vi "数据编码.vi"(0 "table输入":string(combo), 5 "错误常量 2":errorcluster caption="错误输入", 9 "QN":string, 13 "MN":string, 14 "PW":string) -> (4 "错误常量":errorcluster caption="错误输出", 15 "通讯包字符串":string)   [LabVIEW 2016, in "数据传输系统.lvlib"]
panel:
  in  "时间戳 2":string
  out "核查数据发送次数":i32
  out "小时数据发送次数":i32
  out "长度":i32
  in  "数据块":T1
  out "通讯包":T2={"包头（2）"="##", "数据段长度（4）"="", "数据段"="", "CRC校验"="", "包尾"=""}
  # "范例代码：\n\n##0101QN=20160801085857223;ST=32;CN=1062;PW=100000;MN=010000A8900016F000169DC0;Flag=5\n;CP=&&RtdInterval=30&&1C80\\r\\n"
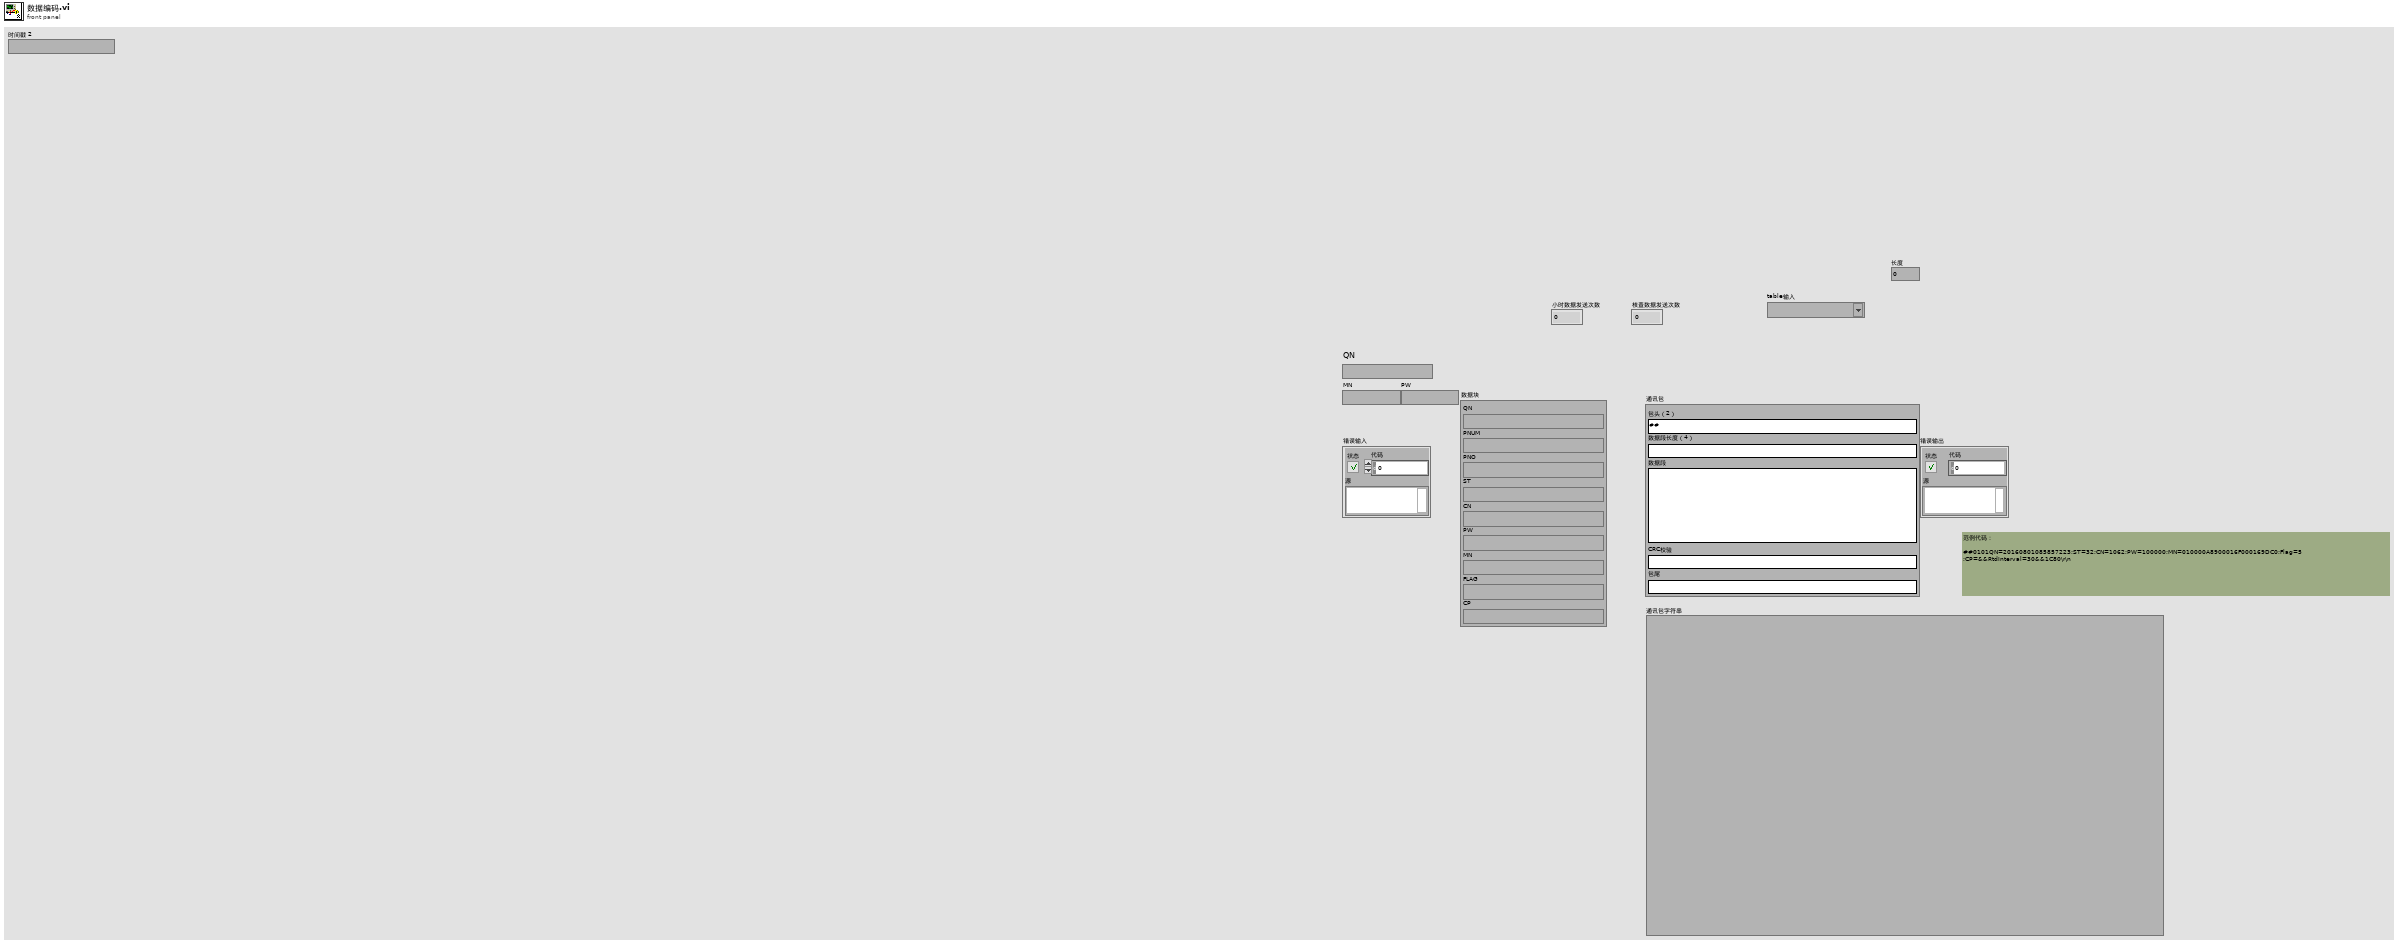
[diagram p1: front panel]
types:
  T1 = cluster{"QN":string, "ST":string, "CN":string, "PW":string, "MN":string, "FLAG":string, "PNUM":string, "PNO":string, "CP":string}
  T2 = cluster{"包头（2）":string, "数据段长度（4）":string, "数据段":string, "CRC校验":string, "包尾":string}
  T3 = cluster{"PH":string[][], "CODCr":string[][], "氨氮":string[][], "CODMn":string[][], "总氮":string[][], "总磷":string[][], "电导率":string[][], "水温":string[][], "DO":string[][], "浊度":string[][], "叶绿素":string[][], "藻密度":string[][], "铜":string[][], "盐度":string[][], "水位":string[][], "流速":string[][], "瞬时流量":string[][], "累计流量":string[][]}
  T4 = cluster{"PH":string[][], "CODCr":string[][], "氨氮":string[][], "CODMn":string[][], "总氮":string[][], "总磷":string[][], "电导率":string[][], "水温":string[][], "DO":string[][], "浊度":string[][], "叶绿素":string[][], "藻密度":string[][], "铜":string[][], "盐度":string[][], "水位":string[][], "流速":string[][], "瞬时流量":string[][], "累积流量":string[][]}
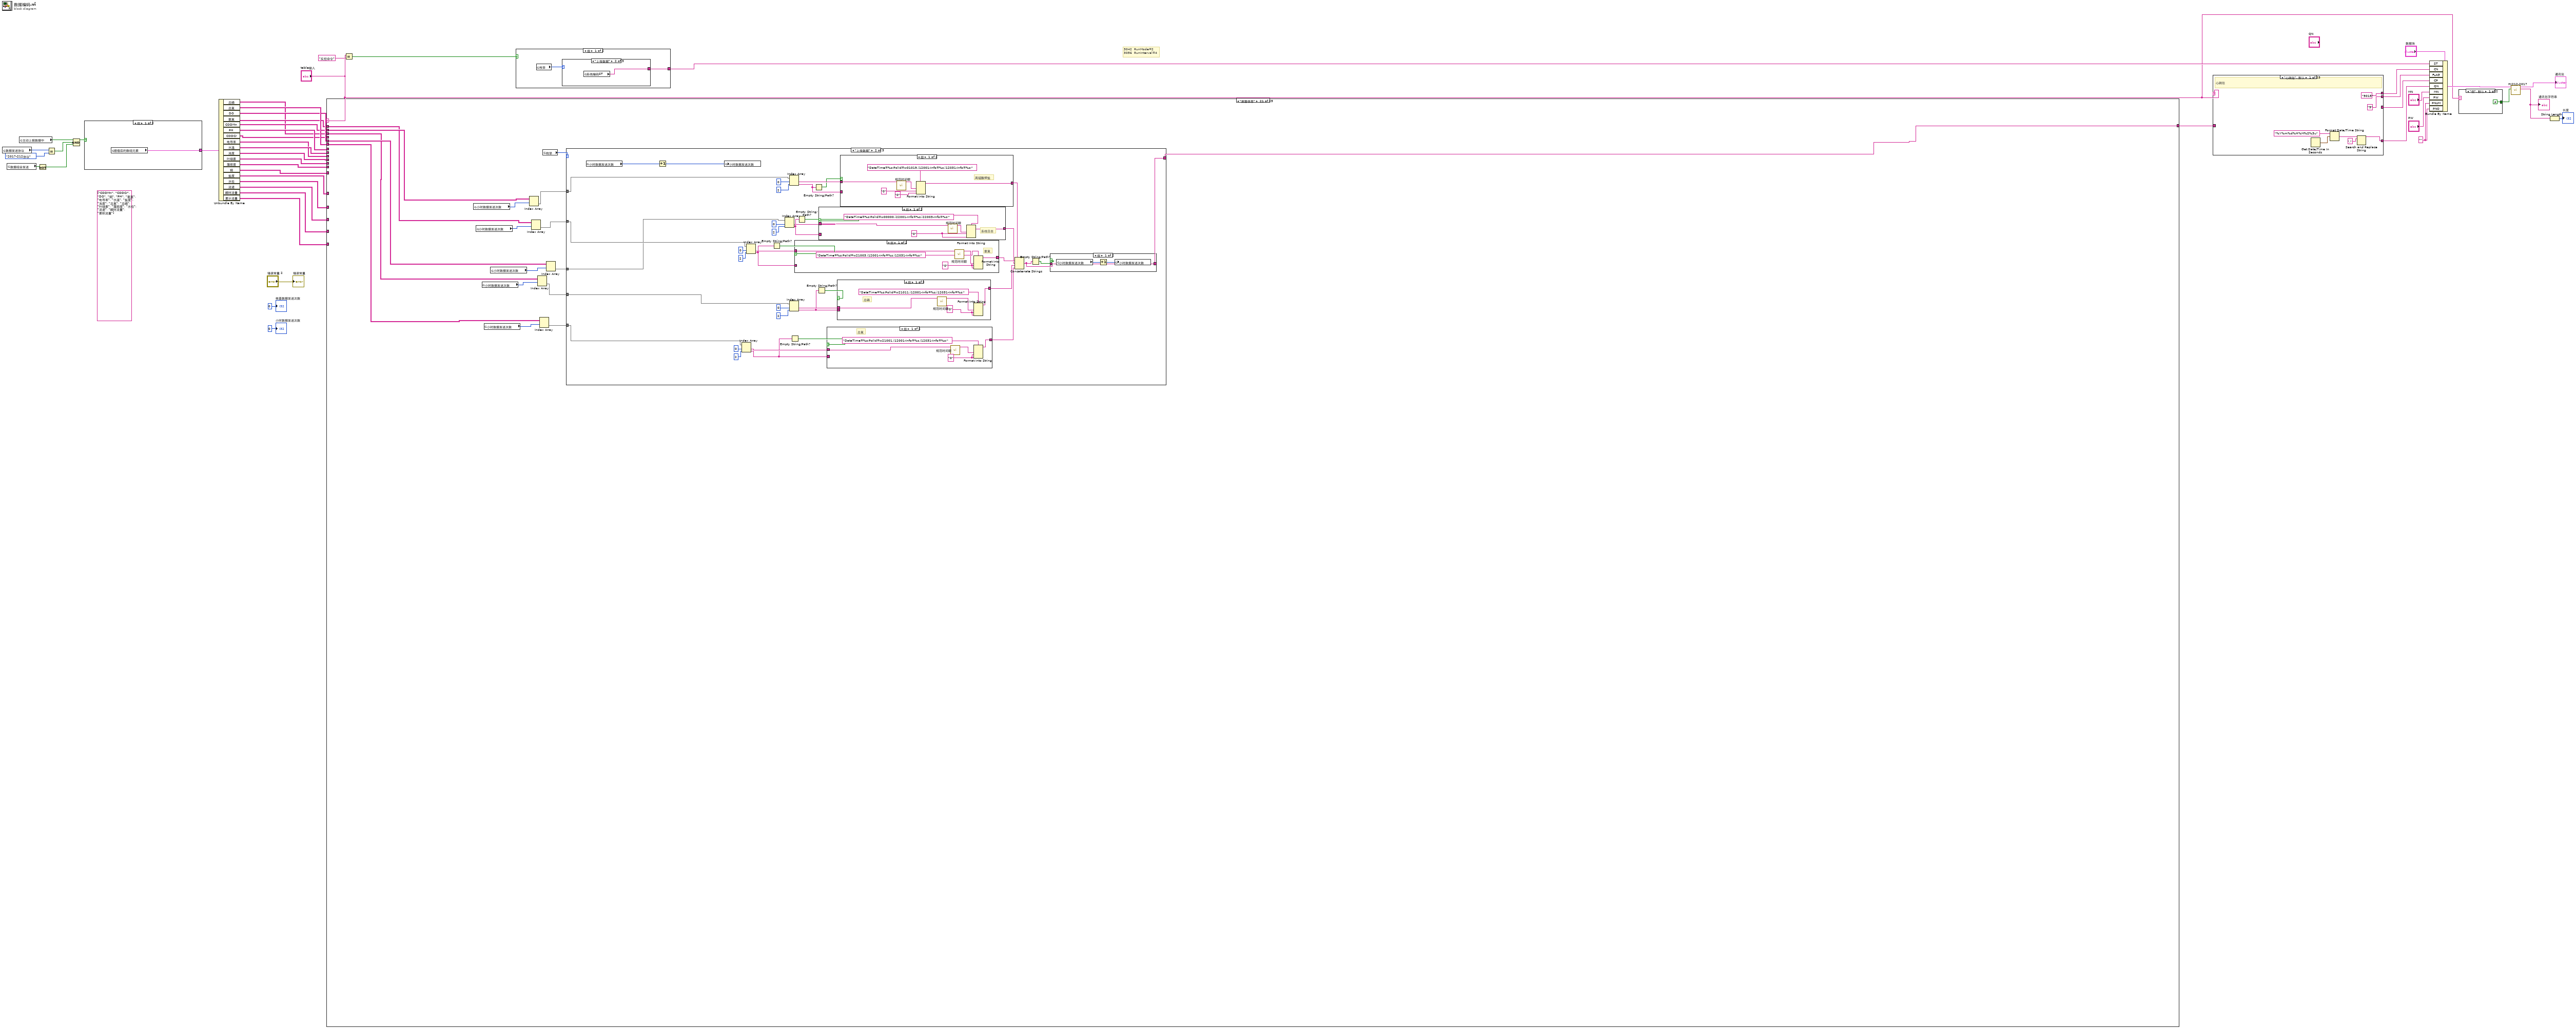
[diagram p0: block diagram]
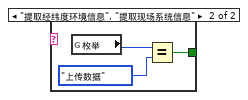
[diagram p2: hidden frame]
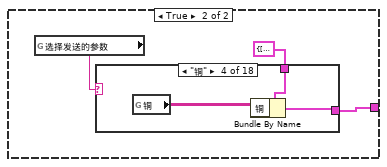
[diagram p3: hidden frame]
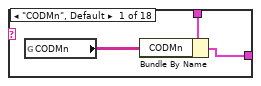
[diagram p4: hidden frame]
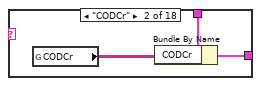
[diagram p5: hidden frame]
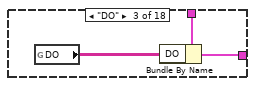
[diagram p6: hidden frame]
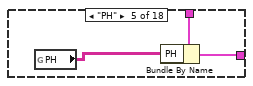
[diagram p7: hidden frame]
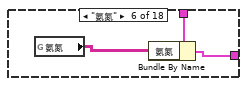
[diagram p8: hidden frame]
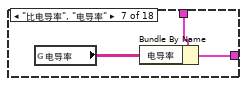
[diagram p9: hidden frame]
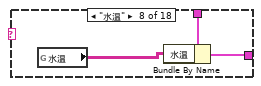
[diagram p10: hidden frame]
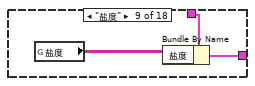
[diagram p11: hidden frame]
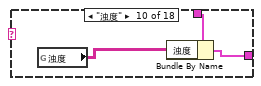
[diagram p12: hidden frame]
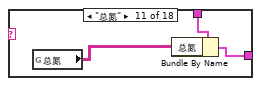
[diagram p13: hidden frame]
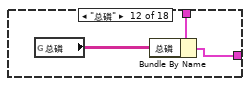
[diagram p14: hidden frame]
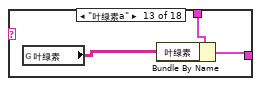
[diagram p15: hidden frame]
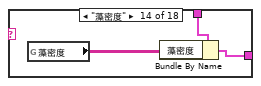
[diagram p16: hidden frame]
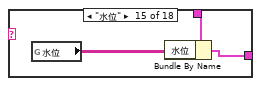
[diagram p17: hidden frame]
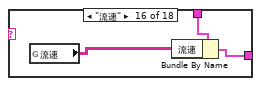
[diagram p18: hidden frame]
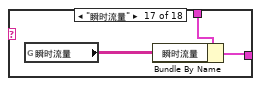
[diagram p19: hidden frame]
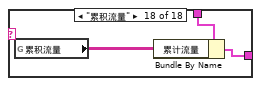
[diagram p20: hidden frame]
diagram:
  (unwired) string[] ["CODMn", "CODCr", "DO", "铜", "PH", "氨氮", "电导率", "水温", "盐度", "浊度", "总氮", "总磷", "叶绿素", "藻密度", "水位", "流速", "瞬时流量", "累积流量"] ("查询参数数组")
  w31 = ""
  # "3042  RunMode=2\n3056  RunInterval=4"
  n1 = global read "断电保存全局.vi" "数据发送协议"() -> (w1:enum16{"2005-212协议", "2017-212协议"})
  n2 = global read "断电保存全局.vi" "数据组合发送"() -> (w3:bool)
  n3 = global read "全局 数据发送重叠.vi" "主动上报数据中"() -> (w17:bool)
  n4 = Not(x=w3) -> (.not. x?=w2:bool)
  n5 = Equal?(x=w1, y=enum16{"2005-212协议", "2017-212协议"}."2017-212协议" ("数据发送版本")) -> (x = y?=w6:bool)
  n6 = Compound Arithmetic op=AND ("复合运算")(w17, w6, w2) -> (w7:bool)
  n7 = case shown="假" w7 {
    tunnel: [w48 w50] -> w18
    frame False {
      n8 = global read "插值后的新数组.vi" "插值后的数组元素"() -> (w48:T4)
    }
    frame True {
      n9 = global read "全局 水样时间.vi" "选择发送的参数"() -> (w51:string)
      n10 = case shown="\"铜\"" w51 {
        tunnel: T3 {"PH"=[], "CODCr"=[], "氨氮"=[], "CODMn"=[], "总氮"=[], "总磷"=[], "电导率"=[], "水温"=[], "DO"=[], "浊度"=[], "叶绿素"=[], "藻密度"=[], "铜"=[], "盐度"=[], "水位"=[], "流速"=[], "瞬时流量"=[], "累计流量"=[]} ("插值后的数组元素") -> [w53 w57 w60 w63 w66 w69 w72 w75 w78 w81 w84 w87 w90 w92 w96 w99 w101 w104]
        tunnel: [w52 w55 w58 w61 w64 w67 w71 w74 w76 w79 w82 w85 w88 w91 w94 w97 w100 w103] -> w50
        frame "CODMn", Default {
          n11 = global read "全局 所有参数.vi" "CODMn"() -> (w54:string[][])
          n12 = Bundle By Name(cluster=w53, "CODMn"=w54) -> (w52:T3)
        }
        frame "CODCr" {
          n13 = global read "全局 所有参数.vi" "CODCr"() -> (w56:string[][])
          n14 = Bundle By Name(cluster=w57, "CODCr"=w56) -> (w55:T3)
        }
        frame "DO" {
          n15 = global read "全局 所有参数.vi" "DO"() -> (w59:string[][])
          n16 = Bundle By Name(cluster=w60, "DO"=w59) -> (w58:T3)
        }
        frame "铜" {
          n17 = global read "全局 所有参数.vi" "铜"() -> (w62:string[][])
          n18 = Bundle By Name(cluster=w63, "铜"=w62) -> (w61:T3)
        }
        frame "PH" {
          n19 = global read "全局 所有参数.vi" "PH"() -> (w65:string[][])
          n20 = Bundle By Name(cluster=w66, "PH"=w65) -> (w64:T3)
        }
        frame "氨氮" {
          n21 = global read "全局 所有参数.vi" "氨氮"() -> (w68:string[][])
          n22 = Bundle By Name(cluster=w69, "氨氮"=w68) -> (w67:T3)
        }
        frame "比电导率", "电导率" {
          n23 = global read "全局 所有参数.vi" "电导率"() -> (w70:string[][])
          n24 = Bundle By Name(cluster=w72, "电导率"=w70) -> (w71:T3)
        }
        frame "水温" {
          n25 = global read "全局 所有参数.vi" "水温"() -> (w73:string[][])
          n26 = Bundle By Name(cluster=w75, "水温"=w73) -> (w74:T3)
        }
        frame "盐度" {
          n27 = global read "全局 所有参数.vi" "盐度"() -> (w77:string[][])
          n28 = Bundle By Name(cluster=w78, "盐度"=w77) -> (w76:T3)
        }
        frame "浊度" {
          n29 = global read "全局 所有参数.vi" "浊度"() -> (w80:string[][])
          n30 = Bundle By Name(cluster=w81, "浊度"=w80) -> (w79:T3)
        }
        frame "总氮" {
          n31 = global read "全局 所有参数.vi" "总氮"() -> (w83:string[][])
          n32 = Bundle By Name(cluster=w84, "总氮"=w83) -> (w82:T3)
        }
        frame "总磷" {
          n33 = global read "全局 所有参数.vi" "总磷"() -> (w86:string[][])
          n34 = Bundle By Name(cluster=w87, "总磷"=w86) -> (w85:T3)
        }
        frame "叶绿素a" {
          n35 = global read "全局 所有参数.vi" "叶绿素"() -> (w89:string[][])
          n36 = Bundle By Name(cluster=w90, "叶绿素"=w89) -> (w88:T3)
        }
        frame "藻密度" {
          n37 = global read "全局 所有参数.vi" "藻密度"() -> (w93:string[][])
          n38 = Bundle By Name(cluster=w92, "藻密度"=w93) -> (w91:T3)
        }
        frame "水位" {
          n39 = global read "全局 所有参数.vi" "水位"() -> (w95:string[][])
          n40 = Bundle By Name(cluster=w96, "水位"=w95) -> (w94:T3)
        }
        frame "流速" {
          n41 = global read "全局 所有参数.vi" "流速"() -> (w98:string[][])
          n42 = Bundle By Name(cluster=w99, "流速"=w98) -> (w97:T3)
        }
        frame "瞬时流量" {
          n43 = global read "全局 所有参数.vi" "瞬时流量"() -> (w102:string[][])
          n44 = Bundle By Name(cluster=w101, "瞬时流量"=w102) -> (w100:T3)
        }
        frame "累积流量" {
          n45 = global read "全局 所有参数.vi" "累积流量"() -> (w105:string[][])
          n46 = Bundle By Name(cluster=w104, "累计流量"=w105) -> (w103:T3)
        }
      }
    }
  }
  n47 = Unbundle By Name(w18) -> ("总磷"=w9:string[][], "总氮"=w14:string[][], "DO"=w13:string[][], "氨氮"=w12:string[][], "CODMn"=w10:string[][], "PH"=w30:string[][], "CODCr"=w11:string[][], "电导率"=w5:string[][], "水温"=w29:string[][], "浊度"=w4:string[][], "叶绿素"=w28:string[][], "藻密度"=w25:string[][], "铜"=w24:string[][], "盐度"=w23:string[][], "水位"=w22:string[][], "流速"=w21:string[][], "瞬时流量"=w20:string[][], "累计流量"=w19:string[][])
  n48 = case shown="\"报警信息\"" "table输入" {
    tunnel: [w107 w111 w126 w147 w170 _ w184 w193 w220 w1717 w2067 w2218 w2390 w2614 w2784 w3041 w3217 w3543 w3639 w3873 w4080 w4186 w4197 w4208 w4219] -> w26
    tunnel: w10 -> [_ _ _ _ _ _ _ _ w218 w1716 w2066 w2230 w2394 w2618 w2788 w3040 w3216 w3542 w3638 w3872 w4079 _ _ _ _]
    tunnel: w12 -> [_ _ _ _ _ _ _ _ w217 w1715 w2065 w2229 w2393 w2617 w2789 w3039 w3215 w3541 w3637 w3871 w4078 _ _ _ _]
    tunnel: w13 -> [_ _ _ _ _ _ _ _ w214 w1714 w2064 w2228 w2372 _ _ _ w3211 w3540 w3636 w3870 w4077 _ _ _ _]
    tunnel: w9 -> [_ _ _ _ _ _ _ _ w209 w1713 w2063 w2227 w2392 w2616 w2787 w3038 w3212 w3539 w3635 w3869 w4076 _ _ _ _]
    tunnel: w14 -> [_ _ _ _ _ _ _ _ w208 w1712 w2062 w2226 w2391 w2615 w2786 w3036 w3214 w3538 w3634 w3868 w4075 _ _ _ _]
    tunnel: w30 -> [_ _ _ _ _ _ _ _ w215 w1711 w2061 w2225 w2376 _ _ _ w3210 _ _ _ _ _ _ _ _]
    tunnel: w11 -> [_ _ _ _ _ _ _ _ w201 w1710 w2060 w2224 w2389 w2613 w2785 w3037 w3213 _ _ w3856 _ _ _ _ _]
    tunnel: w5 -> [_ _ _ _ _ _ _ _ w213 w1709 w2059 w2223 w2369 _ _ _ w3208 _ _ _ _ _ _ _ _]
    tunnel: w29 -> [_ _ _ _ _ _ _ _ w216 w1708 w2058 w2222 _ _ _ _ w3209 _ _ _ _ _ _ _ _]
    tunnel: w4 -> [_ _ _ _ _ _ _ _ w212 w1707 w2057 w2221 w2366 _ _ _ w3207 _ _ _ _ _ _ _ _]
    tunnel: w28 -> [_ _ _ _ _ _ _ _ w211 w1706 w2056 w2220 _ _ _ _ _ _ _ _ _ _ _ _ _]
    tunnel: w25 -> [_ _ _ _ _ _ _ _ w210 w1705 w2055 w2219 _ _ _ _ _ _ _ _ _ _ _ _ _]
    tunnel: w24 -> [_ _ _ _ _ _ _ _ w207 w1675 w2025 w2190 _ _ _ _ _ _ _ _ _ _ _ _ _]
    tunnel: w23 -> [_ _ _ _ _ _ _ _ w206 w1674 w2024 w2189 _ _ _ _ _ _ _ _ _ _ _ _ _]
    tunnel: w22 -> [_ _ _ _ _ _ _ _ w204 _ _ _ _ _ _ _ _ _ _ _ _ _ _ _ _]
    tunnel: w21 -> [_ _ _ _ _ _ _ _ w205 _ _ _ _ _ _ _ _ _ _ _ _ _ _ _ _]
    tunnel: w20 -> [_ _ _ _ _ _ _ _ w203 _ _ _ _ _ _ _ _ _ _ _ _ _ _ _ _]
    tunnel: w19 -> [_ _ _ _ _ _ _ _ w202 _ _ _ _ _ _ _ _ _ _ _ _ _ _ _ _]
    frame "反控命令" {
      n49 = global read "全局 反控命令枚举.vi" "反控命令枚举"() -> (w106:enum16{"返回请求应答", "返回执行结果"})
      n50 = case shown="\"返回请求应答\", 默认" w106 {
        tunnel: ["QnRtn=1" "ExeRtn=1"] -> w107
        frame "返回请求应答", Default {
        }
        frame "返回执行结果" {
        }
      }
    }
    frame "超标留样返回" {
      n51 = global read "全局1.vi" "枚举"() -> (w110:enum16{"返回请求应答", "上传数据", "返回执行结果"})
      n52 = case shown="\"返回请求应答\", 默认" w110 {
        tunnel: ["QnRtn=1" w113 "ExeRtn=1"] -> w111
        frame "返回请求应答", Default {
        }
        frame "上传数据" {
          n53 = global read "全局1.vi" "register values"() -> (w122:u16[])
          n54 = Index Array(array=w122, index=7 ("索引")) -> (element=w115:u16)
          n55 = Get Date/Time In Seconds() -> (seconds since 1Jan1904=w120:timestamp)
          n56 = Number To Decimal String(number=w115) -> (decimal integer string=w116:string)  [unwired: 1 in]
          n57 = Format Date/Time String(time format string (%c)="%Y%m%d%H%M%S" ("时间格式字符串(%c)"), seconds (now)=w120) -> (date/time string=w118:string)  [unwired: 1 in]
          n58 = Format Into String(format string="VaseNo=%s" ("格式字符串"), w116) -> (resulting string=w114:string)  [unwired: 2 in, 1 out]
          n59 = Format Into String(format string="DataTime=%s;%s" ("格式字符串"), w118, w114) -> (resulting string=w113:string)  [unwired: 2 in, 1 out]
        }
        frame "返回执行结果" {
        }
      }
    }
    frame "提取经纬度环境信息" {
      n60 = global read "全局1.vi" "枚举"() -> (w125:enum16{"返回请求应答", "上传数据", "返回执行结果"})
      n61 = case shown="\"返回请求应答\", 默认" w125 {
        tunnel: ["QnRtn=1" w138 "ExeRtn=1"] -> w126
        frame "返回请求应答", Default {
        }
        frame "上传数据" {
          n62 = global read "全局 环境参数.vi" "室温"() -> (w137:string[][])
          n63 = global read "全局 环境参数.vi" "湿度"() -> (w130:string[][])
          n64 = Index Array(array=w137, index (row)=0 ("索引 (行)"), index (col)=1 ("禁用的索引 (列)")) -> (element=w134:string)
          n65 = Index Array(array=w130, index (row)=0 ("索引 (行)"), index (col)=1 ("禁用的索引 (列)")) -> (element=w133:string)
          n66 = Get Date/Time In Seconds() -> (seconds since 1Jan1904=w142:timestamp)
          n67 = Format Date/Time String(time format string (%c)="%Y%m%d%H%M%S" ("时间格式字符串(%c)"), seconds (now)=w142) -> (date/time string=w141:string)  [unwired: 1 in]
          n68 = Format Into String(format string="Temp=%s;" ("格式字符串"), w134) -> (resulting string=w139:string)  [unwired: 2 in, 1 out]
          n69 = Format Into String(format string="Hum=%s;" ("格式字符串"), w133) -> (resulting string=w128:string)  [unwired: 2 in, 1 out]
          n70 = Format Into String(format string="DataTime=%s;%s%s" ("格式字符串"), w141, w139, w128) -> (resulting string=w138:string)  [unwired: 2 in, 1 out]
        }
        frame "返回执行结果" {
        }
      }
    }
    frame "提取现场系统信息" {
      n71 = global read "全局1.vi" "枚举"() -> (w146:enum16{"返回请求应答", "上传数据", "返回执行结果"})
      n72 = case shown="\"上传数据\"" w146 {
        tunnel: ["QnRtn=1" w167 "ExeRtn=1"] -> w147
        frame "返回请求应答", Default {
        }
        frame "上传数据" {
          n73 = global read "全局1.vi" "register values"() -> (w166:u16[])
          n74 = Get Date/Time In Seconds() -> (seconds since 1Jan1904=w152:timestamp)
          n75 = Index Array(array=w166, index #1=0 ("索引"), index #2=6 ("索引")) -> (element #1=w162:u16, element #2=w149:u16)
          n76 = Format Date/Time String(time format string (%c)="%Y%m%d%H%M%S%u" ("时间格式字符串(%c)"), seconds (now)=w152) -> (date/time string=w155:string)  [unwired: 1 in]
          n77 = Number To Decimal String(number=w162) -> (decimal integer string=w164:string)  [unwired: 1 in]
          n78 = Number To Decimal String(number=w149) -> (decimal integer string=w158:string)  [unwired: 1 in]
          n79 = Search and Replace String(input string=w155, search string="." ("搜索字符串")) -> (result string=w151:string)  [unwired: 6 in, 3 out]
          n80 = Format Into String(format string="RunMode=%s;" ("格式字符串"), w164) -> (resulting string=w161:string)  [unwired: 2 in, 1 out]
          n81 = Format Into String(format string="RunInterval=%s;" ("格式字符串"), w158) -> (resulting string=w159:string)  [unwired: 2 in, 1 out]
          n82 = Format Into String(format string="SystemTime=%s;" ("格式字符串"), w151) -> (resulting string=w156:string)  [unwired: 2 in, 1 out]
          n83 = Concatenate Strings(w161, w159, w156) -> (w167:string)
        }
        frame "返回执行结果" {
        }
      }
    }
    frame "提取监测仪表时间" {
      n84 = global read "全局1.vi" "枚举"() -> (w169:enum16{"返回请求应答", "上传数据", "返回执行结果"})
      n85 = case shown="\"上传数据\"" w169 {
        tunnel: ["QnRtn=1" w182 "ExeRtn=1"] -> w170
        frame "返回请求应答", Default {
        }
        frame "上传数据" {
          n86 = global read "全局 提取仪器参数.vi" "仪器编码"() -> (w172:string)
          n87 = Get Date/Time In Seconds() -> (seconds since 1Jan1904=w175:timestamp)
          n88 = Format Date/Time String(time format string (%c)="%Y%m%d%H%M%S%u" ("时间格式字符串(%c)"), seconds (now)=w175) -> (date/time string=w178:string)  [unwired: 1 in]
          n89 = Search and Replace String(input string=w178, search string="." ("搜索字符串")) -> (result string=w174:string)  [unwired: 6 in, 3 out]
          n90 = Format Into String(format string="PolId=%s;" ("格式字符串"), w172) -> (resulting string=w180:string)  [unwired: 2 in, 1 out]
          n91 = Format Into String(format string="SystemTime=%s;" ("格式字符串"), w174) -> (resulting string=w173:string)  [unwired: 2 in, 1 out]
          n92 = Concatenate Strings(w180, w173) -> (w182:string)
        }
        frame "返回执行结果" {
        }
      }
    }
    frame "心跳包", Default {
    }
    frame "提取数采仪时间" {
      (unwired) ""
      n93 = global read "全局1.vi" "枚举"() -> (w185:enum16{"返回请求应答", "上传数据", "返回执行结果"})
      n94 = case shown="\"上传数据\"" w185 {
        tunnel: ["QnRtn=1" w187 "ExeRtn=1"] -> w184
        frame "返回请求应答", Default {
        }
        frame "上传数据" {
          n95 = Get Date/Time In Seconds() -> (seconds since 1Jan1904=w191:timestamp)
          n96 = Format Date/Time String(time format string (%c)="%Y%m%d%H%M%S" ("时间格式字符串(%c)"), seconds (now)=w191) -> (date/time string=w188:string)  [unwired: 1 in]
          n97 = Concatenate Strings("SystemTime=", w188) -> (w187:string)
        }
        frame "返回执行结果" {
        }
      }
    }
    frame "提取实时数据间隔" {
      (unwired) ""
      n98 = global read "全局1.vi" "枚举"() -> (w194:enum16{"返回请求应答", "上传数据", "返回执行结果"})
      n99 = case shown="\"上传数据\"" w194 {
        tunnel: ["QnRtn=1" w198 "ExeRtn=1"] -> w193
        frame "返回请求应答", Default {
        }
        frame "上传数据" {
          n100 = global read "实时数据发送间隔全局.vi" "实时数据发送间隔"() -> (w197:u32)
          n101 = Number To Decimal String(number=w197) -> (decimal integer string=w196:string)  [unwired: 1 in]
          n102 = Concatenate Strings("RtdInterval=", w196) -> (w198:string)
        }
        frame "返回执行结果" {
        }
      }
    }
    frame "实时数据" {
      # "包含质控数据主动上传"
      n103 = global read "全局 实时数据参数.vi" "实时数据参数"() -> (w219:string)
      n104 = case shown="\"水样测试\", 默认" w219 {
        tunnel: [w239 w525 w701 w1022 w1274 w1494] -> w220
        tunnel: w218 -> [w238 w524 w700 w1009 w1272 w1492]
        tunnel: w217 -> [w237 w523 w699 w1010 w1271 w1491]
        tunnel: w216 -> [w236 w522 w698 w1011 _ _]
        tunnel: w215 -> [w235 w521 w697 w1012 w1267 _]
        tunnel: w214 -> [w234 w520 w696 w1013 w1266 _]
        tunnel: w213 -> [w233 w519 w695 w1014 w1265 _]
        tunnel: w212 -> [w232 w518 w694 w1015 w1264 _]
        tunnel: w211 -> [w231 w517 w693 w1016 _ _]
        tunnel: w210 -> [w230 w516 w692 w1017 _ _]
        tunnel: w209 -> [w229 w515 w691 w1018 w1270 w1490]
        tunnel: w208 -> [w228 w514 w690 w1019 w1269 w1489]
        tunnel: w201 -> [w227 w513 w689 w1020 w1268 w1488]
        tunnel: w207 -> [w226 w512 w688 w1008 _ _]
        tunnel: w206 -> [w225 w511 w687 w1007 _ _]
        tunnel: w204 -> [w224 _ _ _ _ _]
        tunnel: w203 -> [w223 _ _ _ _ _]
        tunnel: w202 -> [w222 _ _ _ _ _]
        tunnel: w205 -> [w221 _ _ _ _ _]
        frame "水样测试", Default {
          n105 = global read "全局1.vi" "枚举"() -> (w240:enum16{"返回请求应答", "上传数据", "返回执行结果"})
          n106 = case shown="\"上传数据\"" w240 {
            tunnel: ["QnRtn=1" w328 "ExeRtn=1"] -> w239
            tunnel: w238 -> [_ w340 _]
            tunnel: w237 -> [_ w339 _]
            tunnel: w236 -> [_ w338 _]
            tunnel: w235 -> [_ w337 _]
            tunnel: w234 -> [_ w336 _]
            tunnel: w233 -> [_ w335 _]
            tunnel: w232 -> [_ w334 _]
            tunnel: w231 -> [_ w333 _]
            tunnel: w230 -> [_ w332 _]
            tunnel: w229 -> [_ w331 _]
            tunnel: w228 -> [_ w330 _]
            tunnel: w227 -> [_ w329 _]
            tunnel: w226 -> [_ w287 _]
            tunnel: w225 -> [_ w286 _]
            tunnel: w224 -> [_ w283 _]
            tunnel: w221 -> [_ w282 _]
            tunnel: w223 -> [_ w281 _]
            tunnel: w222 -> [_ w280 _]
            frame "返回请求应答", Default {
            }
            frame "上传数据" {
              # "CODCr"
              # "总氮"
              # "总磷"
              # "PH"
              # "NH3"
              n107 = global read "断电保存全局.vi" "数据发送协议"() -> (w245:enum16{"2005-212协议", "2017-212协议"})
              n108 = global read "断电保存全局.vi" "数据发送协议"() -> (w247:enum16{"2005-212协议", "2017-212协议"})
              n109 = global read "断电保存全局.vi" "数据发送协议"() -> (w250:enum16{"2005-212协议", "2017-212协议"})
              n110 = global read "断电保存全局.vi" "数据发送协议"() -> (w243:enum16{"2005-212协议", "2017-212协议"})
              n111 = global read "断电保存全局.vi" "数据发送协议"() -> (w248:enum16{"2005-212协议", "2017-212协议"})
              n112 = global read "断电保存全局.vi" "数据发送协议"() -> (w249:enum16{"2005-212协议", "2017-212协议"})
              n113 = global read "断电保存全局.vi" "数据发送协议"() -> (w244:enum16{"2005-212协议", "2017-212协议"})
              n114 = global read "断电保存全局.vi" "数据发送协议"() -> (w246:enum16{"2005-212协议", "2017-212协议"})
              n115 = global read "断电保存全局.vi" "数据发送协议"() -> (w242:enum16{"2005-212协议", "2017-212协议"})
              n116 = case shown="\"2017-212协议\", 默认" w243 {
                tunnel: ["060" ("污染物编码") "w21003" ("污染物编码")] -> w324
                frame "2005-212协议" {
                }
                frame "2017-212协议", Default {
                }
              }
              n117 = case shown="\"2005-212协议\"" w245 {
                tunnel: ["001" ("污染物编码") "w01001" ("污染物编码")] -> w317
                frame "2005-212协议" {
                }
                frame "2017-212协议", Default {
                }
              }
              n118 = global read "全局 水样时间.vi" "选择发送的参数"() -> (w265:string)
              n119 = case shown="\"2005-212协议\"" w248 {
                tunnel: ["065" ("污染物编码") "w21001" ("污染物编码")] -> w302
                frame "2005-212协议" {
                }
                frame "2017-212协议", Default {
                }
              }
              n120 = case shown="\"2005-212协议\"" w247 {
                tunnel: ["011" ("污染物编码") "w01018" ("污染物编码")] -> w296
                frame "2005-212协议" {
                }
                frame "2017-212协议", Default {
                }
              }
              n121 = case shown="\"2005-212协议\"" w249 {
                tunnel: ["101" ("污染物编码") "w21011" ("污染物编码")] -> w306
                frame "2005-212协议" {
                }
                frame "2017-212协议", Default {
                }
              }
              n122 = case shown="\"2017-212协议\", 默认" w242 {
                tunnel: w340 -> [_ w352]
                tunnel: ["" ("编码输出") w349] -> w326
                frame "2005-212协议" {
                }
                frame "2017-212协议", Default {
                  # "CODMn"
                  n123 = global read "全局 小时数据发送次数.vi" "小时数据发送次数"() -> (w345:i32)
                  n124 = Index Array(array=w352, index (row)=w345) -> (element=w347:string[])  [unwired: 1 in]
                  n125 = Index Array(array=w347, index #1=3 ("索引"), index #2=0 ("索引"), index #3=5 ("索引")) -> (element #1=w346:string, element #3=w342:string)  [unwired: 1 out]
                  n126 = call "数据编码整合输出.vi"("数据标识"=w342, "数据类型"="-Rtd=", "污染物编码"="w01019", "数据值"=w346) -> ("编码输出"=w349:string)  [unwired: 7 in]
                }
              }
              n127 = case shown="\"铜\"" w265 {
                tunnel: [w486 w487 w488 w489 w490 w491 w492 w493 w494 w495 w496 w497 w498 w499 w500 w501 w502 w503] -> w263
                frame "CODMn", Default {
                  n128 = global read "全局 所有参数.vi" "CODMn"() -> (w486:string[][])
                }
                frame "CODCr" {
                  n129 = global read "全局 所有参数.vi" "CODCr"() -> (w487:string[][])
                }
                frame "DO" {
                  n130 = global read "全局 所有参数.vi" "DO"() -> (w488:string[][])
                }
                frame "铜" {
                  n131 = global read "全局 所有参数.vi" "铜"() -> (w489:string[][])
                }
                frame "PH" {
                  n132 = global read "全局 所有参数.vi" "PH"() -> (w490:string[][])
                }
                frame "氨氮" {
                  n133 = global read "全局 所有参数.vi" "氨氮"() -> (w491:string[][])
                }
                frame "比电导率", "电导率" {
                  n134 = global read "全局 所有参数.vi" "电导率"() -> (w492:string[][])
                }
                frame "水温" {
                  n135 = global read "全局 所有参数.vi" "水温"() -> (w493:string[][])
                }
                frame "盐度" {
                  n136 = global read "全局 所有参数.vi" "盐度"() -> (w494:string[][])
                }
                frame "浊度" {
                  n137 = global read "全局 所有参数.vi" "浊度"() -> (w495:string[][])
                }
                frame "总氮" {
                  n138 = global read "全局 所有参数.vi" "总氮"() -> (w496:string[][])
                }
                frame "总磷" {
                  n139 = global read "全局 所有参数.vi" "总磷"() -> (w497:string[][])
                }
                frame "叶绿素a" {
                  n140 = global read "全局 所有参数.vi" "叶绿素"() -> (w498:string[][])
                }
                frame "藻密度" {
                  n141 = global read "全局 所有参数.vi" "藻密度"() -> (w499:string[][])
                }
                frame "水位" {
                  n142 = global read "全局 所有参数.vi" "水位"() -> (w500:string[][])
                }
                frame "流速" {
                  n143 = global read "全局 所有参数.vi" "流速"() -> (w501:string[][])
                }
                frame "瞬时流量" {
                  n144 = global read "全局 所有参数.vi" "瞬时流量"() -> (w502:string[][])
                }
                frame "累积流量" {
                  n145 = global read "全局 所有参数.vi" "累积流量"() -> (w503:string[][])
                }
              }
              n146 = case shown="\"2017-212协议\", 默认" w246 {
                tunnel: w336 -> [_ w414]
                tunnel: w335 -> [_ w413]
                tunnel: w334 -> [_ w412]
                tunnel: w333 -> [_ w411]
                tunnel: w332 -> [_ w410]
                tunnel: [w364 w405] -> w313
                tunnel: [w364 w400] -> w312
                tunnel: [w364 w395] -> w311
                tunnel: [w364 w390] -> w310
                tunnel: [w364 w385] -> w309
                frame "2005-212协议" {
                  w364 = "" ("编码输出")
                }
                frame "2017-212协议", Default {
                  # "藻密度"
                  # "叶绿素a"
                  # "浊度"
                  # "电导率"
                  # "DO"
                  n147 = global read "全局 小时数据发送次数.vi" "小时数据发送次数"() -> (w380:i32)
                  n148 = global read "全局 小时数据发送次数.vi" "小时数据发送次数"() -> (w381:i32)
                  n149 = global read "全局 小时数据发送次数.vi" "小时数据发送次数"() -> (w382:i32)
                  n150 = global read "全局 小时数据发送次数.vi" "小时数据发送次数"() -> (w383:i32)
                  n151 = global read "全局 小时数据发送次数.vi" "小时数据发送次数"() -> (w384:i32)
                  n152 = Index Array(array=w414, index (row)=w380) -> (element=w409:string[])  [unwired: 1 in]
                  n153 = Index Array(array=w413, index (row)=w381) -> (element=w401:string[])  [unwired: 1 in]
                  n154 = Index Array(array=w412, index (row)=w382) -> (element=w399:string[])  [unwired: 1 in]
                  n155 = Index Array(array=w410, index (row)=w384) -> (element=w386:string[])  [unwired: 1 in]
                  n156 = Index Array(array=w411, index (row)=w383) -> (element=w394:string[])  [unwired: 1 in]
                  n157 = Index Array(array=w409, index #1=5 ("索引"), index #2=3 ("索引")) -> (element #1=w377:string, element #2=w378:string)
                  n158 = Index Array(array=w401, index #1=5 ("索引"), index #2=3 ("索引")) -> (element #1=w376:string, element #2=w375:string)
                  n159 = Index Array(array=w399, index #1=5 ("索引"), index #2=3 ("索引")) -> (element #1=w373:string, element #2=w374:string)
                  n160 = Index Array(array=w386, index #1=5 ("索引"), index #2=3 ("索引")) -> (element #1=w369:string, element #2=w370:string)
                  n161 = Index Array(array=w394, index #1=5 ("索引"), index #2=3 ("索引")) -> (element #1=w372:string, element #2=w371:string)
                  n162 = call "数据编码整合输出.vi"("数据标识"=w377, "数据类型"="-Rtd=", "污染物编码"="w01009", "数据值"=w378) -> ("编码输出"=w405:string)  [unwired: 7 in]
                  n163 = call "数据编码整合输出.vi"("数据标识"=w376, "数据类型"="-Rtd=", "污染物编码"="w01014", "数据值"=w375) -> ("编码输出"=w400:string)  [unwired: 7 in]
                  n164 = call "数据编码整合输出.vi"("数据标识"=w373, "数据类型"="-Rtd=", "污染物编码"="w01003", "数据值"=w374) -> ("编码输出"=w395:string)  [unwired: 7 in]
                  n165 = call "数据编码整合输出.vi"("数据标识"=w369, "数据类型"="-Rtd=", "污染物编码"="w19011", "数据值"=w370) -> ("编码输出"=w385:string)  [unwired: 7 in]
                  n166 = call "数据编码整合输出.vi"("数据标识"=w372, "数据类型"="-Rtd=", "污染物编码"="w01016", "数据值"=w371) -> ("编码输出"=w390:string)  [unwired: 7 in]
                }
              }
              n167 = case shown="\"2017-212协议\", 默认" w244 {
                tunnel: w338 -> [_ w363]
                tunnel: ["" ("编码输出") w358] -> w319
                frame "2005-212协议" {
                }
                frame "2017-212协议", Default {
                  # "水温"
                  n168 = global read "全局 小时数据发送次数.vi" "小时数据发送次数"() -> (w357:i32)
                  n169 = Index Array(array=w363, index (row)=w357) -> (element=w362:string[])  [unwired: 1 in]
                  n170 = Index Array(array=w362, index #1=5 ("索引"), index #2=3 ("索引")) -> (element #1=w355:string, element #2=w356:string)
                  n171 = call "数据编码整合输出.vi"("数据标识"=w355, "数据类型"="-Rtd=", "污染物编码"="w01010", "数据值"=w356) -> ("编码输出"=w358:string)  [unwired: 7 in]
                }
              }
              n172 = global read "全局 小时数据发送次数.vi" "小时数据发送次数"() -> (w291:i32)
              n173 = global read "全局 小时数据发送次数.vi" "小时数据发送次数"() -> (w290:i32)
              n174 = global read "全局 小时数据发送次数.vi" "小时数据发送次数"() -> (w264:i32)
              n175 = global read "全局 小时数据发送次数.vi" "小时数据发送次数"() -> (w289:i32)
              n176 = case shown="\"2017-212协议\", 默认" w250 {
                tunnel: w287 -> [_ w466]
                tunnel: w286 -> [_ w465]
                tunnel: [w415 w464] -> w285
                tunnel: [w415 w463] -> w284
                tunnel: w283 -> [_ w443]
                tunnel: w282 -> [_ w442]
                tunnel: w281 -> [_ w441]
                tunnel: w280 -> [_ w440]
                tunnel: [w415 w439] -> w279
                tunnel: [w415 w438] -> w278
                tunnel: [w415 w437] -> w277
                tunnel: [w415 w436] -> w276
                frame "2005-212协议" {
                  w415 = "" ("编码输出")
                }
                frame "2017-212协议", Default {
                  # "累计流量"
                  # "瞬时流量"
                  # "流速"
                  # "水位"
                  # "盐度"
                  # "总铜"
                  n177 = global read "全局 小时数据发送次数.vi" "小时数据发送次数"() -> (w468:i32)
                  n178 = global read "全局 小时数据发送次数.vi" "小时数据发送次数"() -> (w467:i32)
                  n179 = global read "全局 小时数据发送次数.vi" "小时数据发送次数"() -> (w462:i32)
                  n180 = global read "全局 小时数据发送次数.vi" "小时数据发送次数"() -> (w454:i32)
                  n181 = global read "全局 小时数据发送次数.vi" "小时数据发送次数"() -> (w444:i32)
                  n182 = global read "全局 小时数据发送次数.vi" "小时数据发送次数"() -> (w453:i32)
                  n183 = Index Array(array=w466, index (row)=w468) -> (element=w472:string[])  [unwired: 1 in]
                  n184 = Index Array(array=w465, index (row)=w467) -> (element=w471:string[])  [unwired: 1 in]
                  n185 = Index Array(array=w443, index (row)=w462) -> (element=w459:string[])  [unwired: 1 in]
                  n186 = Index Array(array=w442, index (row)=w454) -> (element=w458:string[])  [unwired: 1 in]
                  n187 = Index Array(array=w440, index (row)=w444) -> (element=w448:string[])  [unwired: 1 in]
                  n188 = Index Array(array=w441, index (row)=w453) -> (element=w449:string[])  [unwired: 1 in]
                  n189 = Index Array(array=w472, index #1=5 ("索引"), index #2=3 ("索引")) -> (element #1=w435:string, element #2=w434:string)
                  n190 = Index Array(array=w471, index #1=5 ("索引"), index #2=3 ("索引")) -> (element #1=w433:string, element #2=w432:string)
                  n191 = Index Array(array=w459, index #1=5 ("索引"), index #2=3 ("索引")) -> (element #1=w429:string, element #2=w430:string)
                  n192 = Index Array(array=w458, index #1=5 ("索引"), index #2=3 ("索引")) -> (element #1=w428:string, element #2=w427:string)
                  n193 = Index Array(array=w448, index #1=5 ("索引"), index #2=3 ("索引")) -> (element #1=w424:string, element #2=w423:string)
                  n194 = Index Array(array=w449, index #1=5 ("索引"), index #2=3 ("索引")) -> (element #1=w426:string, element #2=w425:string)
                  n195 = call "数据编码整合输出.vi"("数据标识"=w435, "数据类型"="-Rtd=", "污染物编码"="w20122", "数据值"=w434) -> ("编码输出"=w464:string)  [unwired: 7 in]
                  n196 = call "数据编码整合输出.vi"("数据标识"=w433, "数据类型"="-Rtd=", "污染物编码"="w01015", "数据值"=w432) -> ("编码输出"=w463:string)  [unwired: 7 in]
                  n197 = call "数据编码整合输出.vi"("数据标识"=w429, "数据类型"="-Rtd=", "污染物编码"="e01201", "数据值"=w430) -> ("编码输出"=w439:string)  [unwired: 7 in]
                  n198 = call "数据编码整合输出.vi"("数据标识"=w428, "数据类型"="-Rtd=", "污染物编码"="e01202", "数据值"=w427) -> ("编码输出"=w438:string)  [unwired: 7 in]
                  n199 = call "数据编码整合输出.vi"("数据标识"=w424, "数据类型"="-Rtd=", "污染物编码"="e01204", "数据值"=w423) -> ("编码输出"=w436:string)  [unwired: 7 in]
                  n200 = call "数据编码整合输出.vi"("数据标识"=w426, "数据类型"="-Rtd=", "污染物编码"="e01203", "数据值"=w425) -> ("编码输出"=w437:string)  [unwired: 7 in]
                }
              }
              n201 = global read "全局 小时数据发送次数.vi" "小时数据发送次数"() -> (w292:i32)
              n202 = global read "全局 小时数据发送次数.vi" "小时数据发送次数"() -> (w293:i32)
              n203 = Index Array(array=w263, index (row)=w264) -> (element=w262:string[])  [unwired: 1 in]
              n204 = Index Array(array=w339, index (row)=w291) -> (element=w321:string[])  [unwired: 1 in]
              n205 = Index Array(array=w337, index (row)=w290) -> (element=w315:string[])  [unwired: 1 in]
              n206 = Index Array(array=w262, index=0 ("索引")) -> (element=w260:string)
              n207 = Index Array(array=w331, index (row)=w292) -> (element=w308:string[])  [unwired: 1 in]
              n208 = Index Array(array=w321, index #1=3 ("索引"), index #2=5 ("索引")) -> (element #1=w320:string, element #2=w274:string)
              n209 = Index Array(array=w330, index (row)=w293) -> (element=w300:string[])  [unwired: 1 in]
              n210 = Index Array(array=w329, index (row)=w289) -> (element=w298:string[])  [unwired: 1 in]
              n211 = Index Array(array=w315, index #1=5 ("索引"), index #2=3 ("索引")) -> (element #1=w273:string, element #2=w272:string)
              n212 = Index Array(array=w308, index #1=5 ("索引"), index #2=3 ("索引")) -> (element #1=w271:string, element #2=w270:string)
              n213 = Index Array(array=w300, index #1=5 ("索引"), index #2=3 ("索引")) -> (element #1=w269:string, element #2=w268:string)
              n214 = Index Array(array=w298, index #1=5 ("索引"), index #2=3 ("索引")) -> (element #1=w267:string, element #2=w266:string)
              n215 = call "规范时间戳.vi"("字符串"=w260) -> ("result string"=w258:string)  [unwired: 10 in]
              n216 = call "数据编码整合输出.vi"("数据标识"=w274, "数据类型"="-Rtd=", "污染物编码"=w324, "数据值"=w320) -> ("编码输出"=w323:string)  [unwired: 7 in]
              n217 = call "数据编码整合输出.vi"("数据标识"=w273, "数据类型"="-Rtd=", "污染物编码"=w317, "数据值"=w272) -> ("编码输出"=w314:string)  [unwired: 7 in]
              n218 = call "数据编码整合输出.vi"("数据标识"=w271, "数据类型"="-Rtd=", "污染物编码"=w306, "数据值"=w270) -> ("编码输出"=w304:string)  [unwired: 7 in]
              n219 = call "数据编码整合输出.vi"("数据标识"=w269, "数据类型"="-Rtd=", "污染物编码"=w302, "数据值"=w268) -> ("编码输出"=w299:string)  [unwired: 7 in]
              n220 = call "数据编码整合输出.vi"("数据标识"=w267, "数据类型"="-Rtd=", "污染物编码"=w296, "数据值"=w266) -> ("编码输出"=w294:string)  [unwired: 7 in]
              n221 = Format Into String(format string="DataTime=%s;", w258) -> (resulting string=w257:string)  [unwired: 2 in, 1 out]
              n222 = Format Into String(format string="%s%s%s%s%s%s%s%s%s%s%s%s%s%s%s%s%s%s" ("格式字符串"), w326, w323, w319, w314, w313, w312, w311, w310, w309, w304, w299, w294, w285, w284, w279, w278, w277, w276) -> (resulting string=w255:string)  [unwired: 2 in, 1 out]
              n223 = Concatenate Strings(w257, w255) -> (w256:string)
              n224 = Empty String/Path?(string/path=w255) -> (empty?=w288:bool)
              n225 = case shown="假" w288 {
                tunnel: [w506 ""] -> w328
                tunnel: w256 -> [w506 _]
                frame False {
                  n226 = global read "全局 小时数据发送次数.vi" "小时数据发送次数"() -> (w505:i32)
                  n227 = Increment(x=w505) -> (x+1=w504:i32)
                  n228 = global write "全局 小时数据发送次数.vi" "小时数据发送次数"(w504) -> ()
                }
                frame True {
                  n229 = global read "全局 小时数据发送次数.vi" "小时数据发送次数"() -> (w508:i32)
                  n230 = Increment(x=w508) -> (x+1=w507:i32)
                  n231 = global write "全局 小时数据发送次数.vi" "小时数据发送次数"(w507) -> ()
                }
              }
            }
            frame "返回执行结果" {
            }
          }
        }
        frame "平行样测试" {
          n232 = global read "全局1.vi" "枚举"() -> (w526:enum16{"返回请求应答", "上传数据", "返回执行结果"})
          n233 = case shown="\"上传数据\"" w526 {
            tunnel: ["QnRtn=1" w580 "ExeRtn=1"] -> w525
            tunnel: w524 -> [_ w572 _]
            tunnel: w523 -> [_ w583 _]
            tunnel: w522 -> [_ _ _]
            tunnel: w521 -> [_ _ _]
            tunnel: w520 -> [_ _ _]
            tunnel: w519 -> [_ _ _]
            tunnel: w518 -> [_ _ _]
            tunnel: w517 -> [_ _ _]
            tunnel: w516 -> [_ _ _]
            tunnel: w515 -> [_ w582 _]
            tunnel: w514 -> [_ w540 _]
            tunnel: w513 -> [_ w530 _]
            tunnel: w512 -> [_ _ _]
            tunnel: w511 -> [_ _ _]
            frame "返回请求应答", Default {
            }
            frame "上传数据" {
              # "CODMn"
              n234 = global read "全局 小时数据发送次数.vi" "小时数据发送次数"() -> (w528:i32)
              n235 = Index Array(array=w572, index (row)=w528) -> (element=w577:string[])  [unwired: 1 in]
              n236 = Index Array(array=w530, index (row)=w528) -> (element=w534:string[])  [unwired: 1 in]
              n237 = Index Array(array=w582, index (row)=w528) -> (element=w553:string[])  [unwired: 1 in]
              n238 = Index Array(array=w540, index (row)=w528) -> (element=w545:string[])  [unwired: 1 in]
              n239 = Index Array(array=w583, index (row)=w528) -> (element=w562:string[])  [unwired: 1 in]
              n240 = Index Array(array=w534, index #1=0 ("索引"), index #2=2 ("索引"), index #3=3 ("索引"), index #4=4 ("索引")) -> (element #2=w531:string, element #3=w533:string, element #4=w532:string)  [unwired: 1 out]
              n241 = Index Array(array=w553, index #1=0 ("索引"), index #2=2 ("索引"), index #3=3 ("索引"), index #4=4 ("索引")) -> (element #2=w550:string, element #3=w552:string, element #4=w551:string)  [unwired: 1 out]
              n242 = Index Array(array=w545, index #1=0 ("索引"), index #2=2 ("索引"), index #3=3 ("索引"), index #4=4 ("索引")) -> (element #2=w548:string, element #3=w546:string, element #4=w547:string)  [unwired: 1 out]
              n243 = Index Array(array=w577, index #1=0 ("索引"), index #2=2 ("索引"), index #3=3 ("索引"), index #4=4 ("索引")) -> (element #1=w570:string, element #2=w568:string, element #3=w573:string, element #4=w575:string)
              n244 = Index Array(array=w562, index #1=0 ("索引"), index #2=2 ("索引"), index #3=3 ("索引"), index #4=4 ("索引")) -> (element #2=w559:string, element #3=w561:string, element #4=w560:string)  [unwired: 1 out]
              n245 = call "规范时间戳.vi"("字符串"=w570) -> ("result string"=w571:string)  [unwired: 10 in]
              n246 = case shown="\"真\", 默认" w531 {
                selector: w531 -> [w585 _]
                tunnel: w531 -> [_ w602]
                tunnel: w532 -> [_ w594]
                tunnel: w533 -> [_ w591]
                tunnel: [w585 w586] -> w529
                frame "" {
                }
                frame "真", Default {
                  # "CODCr"
                  n247 = call "规范时间戳.vi"("字符串"=w591) -> ("result string"=w590:string)  [unwired: 10 in]
                  n248 = call "核查数据编码整合输出.vi"("字段结束"=FALSE, "数据标识"="N" ("字符串"), "数据类型"="-Check=", "污染物编码"="w01018", "数据值"=w602) -> ("编码输出"=w589:string)  [unwired: 6 in]
                  n249 = call "核查数据编码整合输出.vi"("字段结束"=FALSE, "数据类型"="-WaterTime=", "污染物编码"="w01018", "数据值"=w590) -> ("编码输出"=w588:string)  [unwired: 7 in]
                  n250 = call "核查数据编码整合输出.vi"("字段结束"=TRUE, "数据类型"="-Water=", "污染物编码"="w01018", "数据值"=w594) -> ("编码输出"=w587:string)  [unwired: 7 in]
                  n251 = Concatenate Strings(w589, w588, w587) -> (w586:string)
                }
              }
              n252 = case shown="\"真\", 默认" w568 {
                selector: w568 -> [w661 _]
                tunnel: w568 -> [_ w678]
                tunnel: w575 -> [_ w670]
                tunnel: w573 -> [_ w667]
                tunnel: [w661 w662] -> w567
                frame "" {
                }
                frame "真", Default {
                  # "CODMn"
                  n253 = call "规范时间戳.vi"("字符串"=w667) -> ("result string"=w666:string)  [unwired: 10 in]
                  n254 = call "核查数据编码整合输出.vi"("字段结束"=FALSE, "数据标识"="N" ("字符串"), "数据类型"="-Check=", "污染物编码"="w01019", "数据值"=w678) -> ("编码输出"=w665:string)  [unwired: 6 in]
                  n255 = call "核查数据编码整合输出.vi"("字段结束"=FALSE, "数据类型"="-WaterTime=", "污染物编码"="w01019", "数据值"=w666) -> ("编码输出"=w664:string)  [unwired: 7 in]
                  n256 = call "核查数据编码整合输出.vi"("字段结束"=TRUE, "数据类型"="-Water=", "污染物编码"="w01019", "数据值"=w670) -> ("编码输出"=w663:string)  [unwired: 7 in]
                  n257 = Concatenate Strings(w665, w664, w663) -> (w662:string)
                }
              }
              n258 = case shown="\"真\", 默认" w559 {
                selector: w559 -> [w642 _]
                tunnel: w559 -> [_ w659]
                tunnel: w560 -> [_ w651]
                tunnel: w561 -> [_ w648]
                tunnel: [w642 w643] -> w558
                frame "" {
                }
                frame "真", Default {
                  # "NH3"
                  n259 = call "规范时间戳.vi"("字符串"=w648) -> ("result string"=w647:string)  [unwired: 10 in]
                  n260 = call "核查数据编码整合输出.vi"("字段结束"=FALSE, "数据标识"="N" ("字符串"), "数据类型"="-Check=", "污染物编码"="w21003", "数据值"=w659) -> ("编码输出"=w646:string)  [unwired: 6 in]
                  n261 = call "核查数据编码整合输出.vi"("字段结束"=FALSE, "数据类型"="-WaterTime=", "污染物编码"="w21003", "数据值"=w647) -> ("编码输出"=w645:string)  [unwired: 7 in]
                  n262 = call "核查数据编码整合输出.vi"("字段结束"=TRUE, "数据类型"="-Water=", "污染物编码"="w21003", "数据值"=w651) -> ("编码输出"=w644:string)  [unwired: 7 in]
                  n263 = Concatenate Strings(w646, w645, w644) -> (w643:string)
                }
              }
              n264 = case shown="\"真\", 默认" w550 {
                selector: w550 -> [w623 _]
                tunnel: w550 -> [_ w640]
                tunnel: w551 -> [_ w632]
                tunnel: w552 -> [_ w629]
                tunnel: [w623 w624] -> w549
                frame "" {
                }
                frame "真", Default {
                  # "总磷"
                  n265 = call "规范时间戳.vi"("字符串"=w629) -> ("result string"=w628:string)  [unwired: 10 in]
                  n266 = call "核查数据编码整合输出.vi"("字段结束"=FALSE, "数据标识"="N" ("字符串"), "数据类型"="-Check=", "污染物编码"="w21011", "数据值"=w640) -> ("编码输出"=w627:string)  [unwired: 6 in]
                  n267 = call "核查数据编码整合输出.vi"("字段结束"=FALSE, "数据类型"="-WaterTime=", "污染物编码"="w21011", "数据值"=w628) -> ("编码输出"=w626:string)  [unwired: 7 in]
                  n268 = call "核查数据编码整合输出.vi"("字段结束"=TRUE, "数据类型"="-Water=", "污染物编码"="w21011", "数据值"=w632) -> ("编码输出"=w625:string)  [unwired: 7 in]
                  n269 = Concatenate Strings(w627, w626, w625) -> (w624:string)
                }
              }
              n270 = case shown="\"真\", 默认" w548 {
                selector: w548 -> [w604 _]
                tunnel: w548 -> [_ w621]
                tunnel: w547 -> [_ w613]
                tunnel: w546 -> [_ w610]
                tunnel: [w604 w605] -> w539
                frame "" {
                }
                frame "真", Default {
                  # "总氮"
                  n271 = call "规范时间戳.vi"("字符串"=w610) -> ("result string"=w609:string)  [unwired: 10 in]
                  n272 = call "核查数据编码整合输出.vi"("字段结束"=FALSE, "数据标识"="N" ("字符串"), "数据类型"="-Check=", "污染物编码"="w21001", "数据值"=w621) -> ("编码输出"=w608:string)  [unwired: 6 in]
                  n273 = call "核查数据编码整合输出.vi"("字段结束"=FALSE, "数据类型"="-WaterTime=", "污染物编码"="w21001", "数据值"=w609) -> ("编码输出"=w607:string)  [unwired: 7 in]
                  n274 = call "核查数据编码整合输出.vi"("字段结束"=TRUE, "数据类型"="-Water=", "污染物编码"="w21001", "数据值"=w613) -> ("编码输出"=w606:string)  [unwired: 7 in]
                  n275 = Concatenate Strings(w608, w607, w606) -> (w605:string)
                }
              }
              n276 = Empty String/Path?(string/path=w570) -> (empty?=w579:bool)
              n277 = Format Into String(format string="DataTime=%s;%s%s%s%s%s" ("格式字符串"), w571, w567, w558, w549, w539, w529) -> (resulting string=w581:string)  [unwired: 2 in, 1 out]
              n278 = case shown="真" w579 {
                tunnel: [w682 ""] -> w580
                tunnel: w581 -> [w682 _]
                frame False {
                  n279 = global read "全局 小时数据发送次数.vi" "小时数据发送次数"() -> (w681:i32)
                  n280 = Increment(x=w681) -> (x+1=w680:i32)
                  n281 = global write "全局 小时数据发送次数.vi" "小时数据发送次数"(w680) -> ()
                }
                frame True {
                  n282 = global read "全局 小时数据发送次数.vi" "小时数据发送次数"() -> (w684:i32)
                  n283 = Increment(x=w684) -> (x+1=w683:i32)
                  n284 = global write "全局 小时数据发送次数.vi" "小时数据发送次数"(w683) -> ()
                }
              }
            }
            frame "返回执行结果" {
            }
          }
        }
        frame "集成干预测试" {
          n285 = global read "全局1.vi" "枚举"() -> (w702:enum16{"返回请求应答", "上传数据", "返回执行结果"})
          n286 = case shown="\"上传数据\"" w702 {
            tunnel: ["QnRtn=1" w807 "ExeRtn=1"] -> w701
            tunnel: w700 -> [_ w799 _]
            tunnel: w699 -> [_ w785 _]
            tunnel: w698 -> [_ w775 _]
            tunnel: w697 -> [_ w765 _]
            tunnel: w696 -> [_ w745 _]
            tunnel: w695 -> [_ w735 _]
            tunnel: w694 -> [_ w736 _]
            tunnel: w693 -> [_ _ _]
            tunnel: w692 -> [_ _ _]
            tunnel: w691 -> [_ w725 _]
            tunnel: w690 -> [_ w716 _]
            tunnel: w689 -> [_ w704 _]
            tunnel: w688 -> [_ _ _]
            tunnel: w687 -> [_ _ _]
            frame "返回请求应答", Default {
            }
            frame "上传数据" {
              # "CODMn"
              n287 = global read "全局 小时数据发送次数.vi" "小时数据发送次数"() -> (w715:i32)
              n288 = Index Array(array=w799, index (row)=w715) -> (element=w804:string[])  [unwired: 1 in]
              n289 = Index Array(array=w735, index (row)=w715) -> (element=w750:string[])  [unwired: 1 in]
              n290 = Index Array(array=w736, index (row)=w715) -> (element=w740:string[])  [unwired: 1 in]
              n291 = Index Array(array=w716, index (row)=w715) -> (element=w721:string[])  [unwired: 1 in]
              n292 = Index Array(array=w725, index (row)=w715) -> (element=w729:string[])  [unwired: 1 in]
              n293 = Index Array(array=w745, index (row)=w715) -> (element=w759:string[])  [unwired: 1 in]
              n294 = Index Array(array=w765, index (row)=w715) -> (element=w769:string[])  [unwired: 1 in]
              n295 = Index Array(array=w704) -> (element=w711:string[])  [unwired: 2 in]
              n296 = Index Array(array=w775, index (row)=w715) -> (element=w779:string[])  [unwired: 1 in]
              n297 = Index Array(array=w785, index (row)=w715) -> (element=w789:string[])  [unwired: 1 in]
              n298 = Index Array(array=w750, index #1=0 ("索引"), index #2=2 ("索引"), index #3=3 ("索引"), index #4=4 ("索引")) -> (element #2=w747:string, element #3=w749:string, element #4=w748:string)  [unwired: 1 out]
              n299 = Index Array(array=w740, index #1=0 ("索引"), index #2=2 ("索引"), index #3=3 ("索引"), index #4=4 ("索引")) -> (element #2=w737:string, element #3=w739:string, element #4=w738:string)  [unwired: 1 out]
              n300 = Index Array(array=w721, index #1=0 ("索引"), index #2=2 ("索引"), index #3=3 ("索引"), index #4=4 ("索引")) -> (element #2=w724:string, element #3=w722:string, element #4=w723:string)  [unwired: 1 out]
              n301 = Index Array(array=w729, index #1=0 ("索引"), index #2=2 ("索引"), index #3=3 ("索引"), index #4=4 ("索引")) -> (element #2=w726:string, element #3=w728:string, element #4=w727:string)  [unwired: 1 out]
              n302 = Index Array(array=w759, index #1=0 ("索引"), index #2=2 ("索引"), index #3=3 ("索引"), index #4=4 ("索引")) -> (element #2=w756:string, element #3=w758:string, element #4=w757:string)  [unwired: 1 out]
              n303 = Index Array(array=w769, index #1=0 ("索引"), index #2=2 ("索引"), index #3=3 ("索引"), index #4=4 ("索引")) -> (element #2=w766:string, element #3=w768:string, element #4=w767:string)  [unwired: 1 out]
              n304 = Index Array(array=w711, index #1=0 ("索引"), index #2=2 ("索引"), index #4=4 ("索引")) -> (element #2=w714:string, element #3=w712:string, element #4=w713:string)  [unwired: 1 in, 1 out]
              n305 = Index Array(array=w779, index #1=0 ("索引"), index #2=2 ("索引"), index #3=3 ("索引"), index #4=4 ("索引")) -> (element #2=w776:string, element #3=w778:string, element #4=w777:string)  [unwired: 1 out]
              n306 = Index Array(array=w789, index #1=0 ("索引"), index #2=2 ("索引"), index #3=3 ("索引"), index #4=4 ("索引")) -> (element #2=w786:string, element #3=w788:string, element #4=w787:string)  [unwired: 1 out]
              n307 = Index Array(array=w804, index #1=0 ("索引"), index #2=2 ("索引"), index #3=3 ("索引"), index #4=4 ("索引")) -> (element #1=w797:string, element #2=w795:string, element #3=w800:string, element #4=w802:string)
              n308 = call "规范时间戳.vi"("字符串"=w797) -> ("result string"=w798:string)  [unwired: 10 in]
              n309 = case shown="\"真\", 默认" w747 {
                selector: w747 -> [w886 _]
                tunnel: w747 -> [_ w903]
                tunnel: w748 -> [_ w895]
                tunnel: w749 -> [_ w892]
                tunnel: [w886 w887] -> w746
                frame "" {
                }
                frame "真", Default {
                  # "电导率"
                  n310 = call "规范时间戳.vi"("字符串"=w892) -> ("result string"=w891:string)  [unwired: 10 in]
                  n311 = call "核查数据编码整合输出.vi"("字段结束"=FALSE, "数据标识"="N" ("字符串"), "数据类型"="-Check=", "污染物编码"="w01014", "数据值"=w903) -> ("编码输出"=w890:string)  [unwired: 6 in]
                  n312 = call "核查数据编码整合输出.vi"("字段结束"=FALSE, "数据类型"="-WaterTime=", "污染物编码"="w01014", "数据值"=w891) -> ("编码输出"=w889:string)  [unwired: 7 in]
                  n313 = call "核查数据编码整合输出.vi"("字段结束"=TRUE, "数据类型"="-Water=", "污染物编码"="w01014", "数据值"=w895) -> ("编码输出"=w888:string)  [unwired: 7 in]
                  n314 = Concatenate Strings(w890, w889, w888) -> (w887:string)
                }
              }
              n315 = case shown="\"真\", 默认" w737 {
                selector: w737 -> [w867 _]
                tunnel: w737 -> [_ w884]
                tunnel: w738 -> [_ w876]
                tunnel: w739 -> [_ w873]
                tunnel: [w867 w868] -> w734
                frame "" {
                }
                frame "真", Default {
                  # "浊度"
                  n316 = call "规范时间戳.vi"("字符串"=w873) -> ("result string"=w872:string)  [unwired: 10 in]
                  n317 = call "核查数据编码整合输出.vi"("字段结束"=FALSE, "数据标识"="N" ("字符串"), "数据类型"="-Check=", "污染物编码"="w01003", "数据值"=w884) -> ("编码输出"=w871:string)  [unwired: 6 in]
                  n318 = call "核查数据编码整合输出.vi"("字段结束"=FALSE, "数据类型"="-WaterTime=", "污染物编码"="w01003", "数据值"=w872) -> ("编码输出"=w870:string)  [unwired: 7 in]
                  n319 = call "核查数据编码整合输出.vi"("字段结束"=TRUE, "数据类型"="-Water=", "污染物编码"="w01003", "数据值"=w876) -> ("编码输出"=w869:string)  [unwired: 7 in]
                  n320 = Concatenate Strings(w871, w870, w869) -> (w868:string)
                }
              }
              n321 = case shown="\"真\", 默认" w724 {
                selector: w724 -> [w829 _]
                tunnel: w724 -> [_ w846]
                tunnel: w723 -> [_ w838]
                tunnel: w722 -> [_ w835]
                tunnel: [w829 w830] -> w706
                frame "" {
                }
                frame "真", Default {
                  # "总氮"
                  n322 = call "规范时间戳.vi"("字符串"=w835) -> ("result string"=w834:string)  [unwired: 10 in]
                  n323 = call "核查数据编码整合输出.vi"("字段结束"=FALSE, "数据标识"="N" ("字符串"), "数据类型"="-Check=", "污染物编码"="w21001", "数据值"=w846) -> ("编码输出"=w833:string)  [unwired: 6 in]
                  n324 = call "核查数据编码整合输出.vi"("字段结束"=FALSE, "数据类型"="-WaterTime=", "污染物编码"="w21001", "数据值"=w834) -> ("编码输出"=w832:string)  [unwired: 7 in]
                  n325 = call "核查数据编码整合输出.vi"("字段结束"=TRUE, "数据类型"="-Water=", "污染物编码"="w21001", "数据值"=w838) -> ("编码输出"=w831:string)  [unwired: 7 in]
                  n326 = Concatenate Strings(w833, w832, w831) -> (w830:string)
                }
              }
              n327 = case shown="\"真\", 默认" w726 {
                selector: w726 -> [w848 _]
                tunnel: w726 -> [_ w865]
                tunnel: w727 -> [_ w857]
                tunnel: w728 -> [_ w854]
                tunnel: [w848 w849] -> w707
                frame "" {
                }
                frame "真", Default {
                  # "总磷"
                  n328 = call "规范时间戳.vi"("字符串"=w854) -> ("result string"=w853:string)  [unwired: 10 in]
                  n329 = call "核查数据编码整合输出.vi"("字段结束"=FALSE, "数据标识"="N" ("字符串"), "数据类型"="-Check=", "污染物编码"="w21011", "数据值"=w865) -> ("编码输出"=w852:string)  [unwired: 6 in]
                  n330 = call "核查数据编码整合输出.vi"("字段结束"=FALSE, "数据类型"="-WaterTime=", "污染物编码"="w21011", "数据值"=w853) -> ("编码输出"=w851:string)  [unwired: 7 in]
                  n331 = call "核查数据编码整合输出.vi"("字段结束"=TRUE, "数据类型"="-Water=", "污染物编码"="w21011", "数据值"=w857) -> ("编码输出"=w850:string)  [unwired: 7 in]
                  n332 = Concatenate Strings(w852, w851, w850) -> (w849:string)
                }
              }
              n333 = case shown="\"真\", 默认" w756 {
                selector: w756 -> [w905 _]
                tunnel: w756 -> [_ w922]
                tunnel: w757 -> [_ w914]
                tunnel: w758 -> [_ w911]
                tunnel: [w905 w906] -> w755
                frame "" {
                }
                frame "真", Default {
                  # "DO"
                  n334 = call "规范时间戳.vi"("字符串"=w911) -> ("result string"=w910:string)  [unwired: 10 in]
                  n335 = call "核查数据编码整合输出.vi"("字段结束"=FALSE, "数据标识"="N" ("字符串"), "数据类型"="-Check=", "污染物编码"="w01009", "数据值"=w922) -> ("编码输出"=w909:string)  [unwired: 6 in]
                  n336 = call "核查数据编码整合输出.vi"("字段结束"=FALSE, "数据类型"="-WaterTime=", "污染物编码"="w01009", "数据值"=w910) -> ("编码输出"=w908:string)  [unwired: 7 in]
                  n337 = call "核查数据编码整合输出.vi"("字段结束"=TRUE, "数据类型"="-Water=", "污染物编码"="w01009", "数据值"=w914) -> ("编码输出"=w907:string)  [unwired: 7 in]
                  n338 = Concatenate Strings(w909, w908, w907) -> (w906:string)
                }
              }
              n339 = case shown="\"真\", 默认" w766 {
                selector: w766 -> [w924 _]
                tunnel: w766 -> [_ w941]
                tunnel: w767 -> [_ w933]
                tunnel: w768 -> [_ w930]
                tunnel: [w924 w925] -> w764
                frame "" {
                }
                frame "真", Default {
                  # "PH"
                  n340 = call "规范时间戳.vi"("字符串"=w930) -> ("result string"=w929:string)  [unwired: 10 in]
                  n341 = call "核查数据编码整合输出.vi"("字段结束"=FALSE, "数据标识"="N" ("字符串"), "数据类型"="-Check=", "污染物编码"="w01001", "数据值"=w941) -> ("编码输出"=w928:string)  [unwired: 6 in]
                  n342 = call "核查数据编码整合输出.vi"("字段结束"=FALSE, "数据类型"="-WaterTime=", "污染物编码"="w01001", "数据值"=w929) -> ("编码输出"=w927:string)  [unwired: 7 in]
                  n343 = call "核查数据编码整合输出.vi"("字段结束"=TRUE, "数据类型"="-Water=", "污染物编码"="w01001", "数据值"=w933) -> ("编码输出"=w926:string)  [unwired: 7 in]
                  n344 = Concatenate Strings(w928, w927, w926) -> (w925:string)
                }
              }
              n345 = case shown="\"真\", 默认" w714 {
                selector: w714 -> [w810 _]
                tunnel: w714 -> [_ w827]
                tunnel: w713 -> [_ w819]
                tunnel: w712 -> [_ w816]
                tunnel: [w810 w811] -> w705
                frame "" {
                }
                frame "真", Default {
                  # "CODCr"
                  n346 = call "规范时间戳.vi"("字符串"=w816) -> ("result string"=w815:string)  [unwired: 10 in]
                  n347 = call "核查数据编码整合输出.vi"("字段结束"=FALSE, "数据标识"="N" ("字符串"), "数据类型"="-Check=", "污染物编码"="w01018", "数据值"=w827) -> ("编码输出"=w814:string)  [unwired: 6 in]
                  n348 = call "核查数据编码整合输出.vi"("字段结束"=FALSE, "数据类型"="-WaterTime=", "污染物编码"="w01018", "数据值"=w815) -> ("编码输出"=w813:string)  [unwired: 7 in]
                  n349 = call "核查数据编码整合输出.vi"("字段结束"=TRUE, "数据类型"="-Water=", "污染物编码"="w01018", "数据值"=w819) -> ("编码输出"=w812:string)  [unwired: 7 in]
                  n350 = Concatenate Strings(w814, w813, w812) -> (w811:string)
                }
              }
              n351 = case shown="\"真\", 默认" w776 {
                selector: w776 -> [w943 _]
                tunnel: w776 -> [_ w960]
                tunnel: w777 -> [_ w952]
                tunnel: w778 -> [_ w949]
                tunnel: [w943 w944] -> w774
                frame "" {
                }
                frame "真", Default {
                  # "水温"
                  n352 = call "规范时间戳.vi"("字符串"=w949) -> ("result string"=w948:string)  [unwired: 10 in]
                  n353 = call "核查数据编码整合输出.vi"("字段结束"=FALSE, "数据标识"="N" ("字符串"), "数据类型"="-Check=", "污染物编码"="w01010", "数据值"=w960) -> ("编码输出"=w947:string)  [unwired: 6 in]
                  n354 = call "核查数据编码整合输出.vi"("字段结束"=FALSE, "数据类型"="-WaterTime=", "污染物编码"="w01010", "数据值"=w948) -> ("编码输出"=w946:string)  [unwired: 7 in]
                  n355 = call "核查数据编码整合输出.vi"("字段结束"=TRUE, "数据类型"="-Water=", "污染物编码"="w01010", "数据值"=w952) -> ("编码输出"=w945:string)  [unwired: 7 in]
                  n356 = Concatenate Strings(w947, w946, w945) -> (w944:string)
                }
              }
              n357 = case shown="\"真\", 默认" w786 {
                selector: w786 -> [w962 _]
                tunnel: w786 -> [_ w979]
                tunnel: w787 -> [_ w971]
                tunnel: w788 -> [_ w968]
                tunnel: [w962 w963] -> w784
                frame "" {
                }
                frame "真", Default {
                  # "NH3"
                  n358 = call "规范时间戳.vi"("字符串"=w968) -> ("result string"=w967:string)  [unwired: 10 in]
                  n359 = call "核查数据编码整合输出.vi"("字段结束"=FALSE, "数据标识"="N" ("字符串"), "数据类型"="-Check=", "污染物编码"="w21003", "数据值"=w979) -> ("编码输出"=w966:string)  [unwired: 6 in]
                  n360 = call "核查数据编码整合输出.vi"("字段结束"=FALSE, "数据类型"="-WaterTime=", "污染物编码"="w21003", "数据值"=w967) -> ("编码输出"=w965:string)  [unwired: 7 in]
                  n361 = call "核查数据编码整合输出.vi"("字段结束"=TRUE, "数据类型"="-Water=", "污染物编码"="w21003", "数据值"=w971) -> ("编码输出"=w964:string)  [unwired: 7 in]
                  n362 = Concatenate Strings(w966, w965, w964) -> (w963:string)
                }
              }
              n363 = case shown="\"真\", 默认" w795 {
                selector: w795 -> [w981 _]
                tunnel: w795 -> [_ w998]
                tunnel: w802 -> [_ w990]
                tunnel: w800 -> [_ w987]
                tunnel: [w981 w982] -> w794
                frame "" {
                }
                frame "真", Default {
                  # "CODMn"
                  n364 = call "规范时间戳.vi"("字符串"=w987) -> ("result string"=w986:string)  [unwired: 10 in]
                  n365 = call "核查数据编码整合输出.vi"("字段结束"=FALSE, "数据标识"="N" ("字符串"), "数据类型"="-Check=", "污染物编码"="w01019", "数据值"=w998) -> ("编码输出"=w985:string)  [unwired: 6 in]
                  n366 = call "核查数据编码整合输出.vi"("字段结束"=FALSE, "数据类型"="-WaterTime=", "污染物编码"="w01019", "数据值"=w986) -> ("编码输出"=w984:string)  [unwired: 7 in]
                  n367 = call "核查数据编码整合输出.vi"("字段结束"=TRUE, "数据类型"="-Water=", "污染物编码"="w01019", "数据值"=w990) -> ("编码输出"=w983:string)  [unwired: 7 in]
                  n368 = Concatenate Strings(w985, w984, w983) -> (w982:string)
                }
              }
              n369 = Empty String/Path?(string/path=w797) -> (empty?=w806:bool)
              n370 = Format Into String(format string="DataTime=%s;%s%s%s%s%s%s%s%s%s%s" ("格式字符串"), w798, w794, w784, w774, w764, w755, w746, w734, w707, w706, w705) -> (resulting string=w808:string)  [unwired: 2 in, 1 out]
              n371 = case shown="真" w806 {
                tunnel: [w1002 ""] -> w807
                tunnel: w808 -> [w1002 _]
                frame False {
                  n372 = global read "全局 小时数据发送次数.vi" "小时数据发送次数"() -> (w1001:i32)
                  n373 = Increment(x=w1001) -> (x+1=w1000:i32)
                  n374 = global write "全局 小时数据发送次数.vi" "小时数据发送次数"(w1000) -> ()
                }
                frame True {
                  n375 = global read "全局 小时数据发送次数.vi" "小时数据发送次数"() -> (w1004:i32)
                  n376 = Increment(x=w1004) -> (x+1=w1003:i32)
                  n377 = global write "全局 小时数据发送次数.vi" "小时数据发送次数"(w1003) -> ()
                }
              }
            }
            frame "返回执行结果" {
            }
          }
        }
        frame "加标回收测试" {
          n378 = global read "全局1.vi" "枚举"() -> (w1021:enum16{"返回请求应答", "上传数据", "返回执行结果"})
          n379 = case shown="\"上传数据\"" w1021 {
            tunnel: ["QnRtn=1" w1239 "ExeRtn=1"] -> w1022
            tunnel: w1020 -> [_ w1245 _]
            tunnel: w1019 -> [_ w1244 _]
            tunnel: w1018 -> [_ w1243 _]
            tunnel: w1017 -> [_ _ _]
            tunnel: w1016 -> [_ _ _]
            tunnel: w1015 -> [_ _ _]
            tunnel: w1014 -> [_ _ _]
            tunnel: w1013 -> [_ _ _]
            tunnel: w1012 -> [_ _ _]
            tunnel: w1011 -> [_ _ _]
            tunnel: w1010 -> [_ w1242 _]
            tunnel: w1009 -> [_ w1241 _]
            tunnel: w1008 -> [_ _ _]
            tunnel: w1007 -> [_ _ _]
            frame "返回请求应答", Default {
            }
            frame "上传数据" {
              # "w01001-Check=63.0,w01001-WaterTime=20160801080000,w01001-Water=45.23,w01001-Chroma=1000,w01001-Volume=0.2,w01001-DVolume=200,w01003-Flag=N;"
              # "CODCr"
              # "总氮"
              # "总磷"
              # "NH3"
              # "CODMn"
              n380 = global read "全局 小时数据发送次数.vi" "小时数据发送次数"() -> (w1246:i32)
              n381 = Index Array(array=w1244, index (row)=w1246) -> (element=w1251:string[])  [unwired: 1 in]
              n382 = Index Array(array=w1241, index (row)=w1246) -> (element=w1253:string[])  [unwired: 1 in]
              n383 = Index Array(array=w1242, index (row)=w1246) -> (element=w1255:string[])  [unwired: 1 in]
              n384 = Index Array(array=w1251, index #1=4 ("索引"), index #2=2 ("索引"), index #3=3 ("索引"), index #4=5 ("索引"), index #5=6 ("索引"), index #6=7 ("索引")) -> (element #1=w1140:string, element #2=w1034:string, element #3=w1125:string, element #4=w1124:string, element #5=w1123:string, element #6=w1122:string)
              n385 = Index Array(array=w1243, index (row)=w1246) -> (element=w1252:string[])  [unwired: 1 in]
              n386 = Index Array(array=w1245, index (row)=w1246) -> (element=w1250:string[])  [unwired: 1 in]
              n387 = Index Array(array=w1255, index #1=4 ("索引"), index #2=2 ("索引"), index #3=3 ("索引"), index #4=5 ("索引"), index #5=6 ("索引"), index #6=7 ("索引")) -> (element #1=w1210:string, element #2=w1038:string, element #3=w1190:string, element #4=w1189:string, element #5=w1188:string, element #6=w1187:string)
              n388 = Index Array(array=w1253, index #1=0 ("索引"), index #2=4 ("索引"), index #3=2 ("索引"), index #4=3 ("索引"), index #5=5 ("索引"), index #6=6 ("索引"), index #7=7 ("索引")) -> (element #1=w1248:string, element #2=w1236:string, element #3=w1060:string, element #4=w1228:string, element #5=w1225:string, element #6=w1221:string, element #7=w1220:string)
              n389 = Index Array(array=w1252, index #1=4 ("索引"), index #2=2 ("索引"), index #3=3 ("索引"), index #4=5 ("索引"), index #5=6 ("索引"), index #6=7 ("索引")) -> (element #1=w1168:string, element #2=w1036:string, element #3=w1145:string, element #4=w1144:string, element #5=w1143:string, element #6=w1142:string)
              n390 = Index Array(array=w1250, index #1=4 ("索引"), index #2=2 ("索引"), index #3=3 ("索引"), index #4=5 ("索引"), index #5=6 ("索引"), index #6=7 ("索引")) -> (element #1=w1138:string, element #2=w1032:string, element #3=w1075:string, element #4=w1076:string, element #5=w1077:string, element #6=w1078:string)
              n391 = call "规范时间戳.vi"("字符串"=w1248) -> ("result string"=w1247:string)  [unwired: 10 in]
              n392 = call "规范时间戳.vi"("字符串"=w1060) -> ("result string"=w1059:string)  [unwired: 10 in]
              n393 = call "规范时间戳.vi"("字符串"=w1034) -> ("result string"=w1033:string)  [unwired: 10 in]
              n394 = call "规范时间戳.vi"("字符串"=w1036) -> ("result string"=w1035:string)  [unwired: 10 in]
              n395 = call "规范时间戳.vi"("字符串"=w1038) -> ("result string"=w1037:string)  [unwired: 10 in]
              n396 = call "规范时间戳.vi"("字符串"=w1032) -> ("result string"=w1031:string)  [unwired: 10 in]
              n397 = call "核查数据编码整合输出.vi"("字段结束"=FALSE, "数据标识"="N" ("字符串"), "数据类型"="-Check=", "污染物编码"="w21011", "数据值"=w1168) -> ("编码输出"=w1167:string)  [unwired: 6 in]
              n398 = call "核查数据编码整合输出.vi"("字段结束"=FALSE, "数据标识"="N" ("字符串"), "数据类型"="-WaterTime=", "污染物编码"="w21011", "数据值"=w1035) -> ("编码输出"=w1150:string)  [unwired: 6 in]
              n399 = call "核查数据编码整合输出.vi"("字段结束"=FALSE, "数据标识"="N" ("字符串"), "数据类型"="-Water=", "污染物编码"="w21011", "数据值"=w1145) -> ("编码输出"=w1149:string)  [unwired: 6 in]
              n400 = call "核查数据编码整合输出.vi"("字段结束"=TRUE, "数据标识"="N" ("字符串"), "数据类型"="-DVolume=", "污染物编码"="w21011", "数据值"=w1142) -> ("编码输出"=w1146:string)  [unwired: 6 in]
              n401 = call "核查数据编码整合输出.vi"("字段结束"=FALSE, "数据标识"="N" ("字符串"), "数据类型"="-Chroma=", "污染物编码"="w21011", "数据值"=w1144) -> ("编码输出"=w1148:string)  [unwired: 6 in]
              n402 = call "核查数据编码整合输出.vi"("字段结束"=FALSE, "数据标识"="N" ("字符串"), "数据类型"="-Volume=", "污染物编码"="w21011", "数据值"=w1143) -> ("编码输出"=w1147:string)  [unwired: 6 in]
              n403 = call "核查数据编码整合输出.vi"("字段结束"=FALSE, "数据标识"="N" ("字符串"), "数据类型"="-WaterTime=", "污染物编码"="w21001", "数据值"=w1033) -> ("编码输出"=w1120:string)  [unwired: 6 in]
              n404 = call "核查数据编码整合输出.vi"("字段结束"=FALSE, "数据类型"="-Volume=", "污染物编码"="w01019", "数据值"=w1221) -> ("编码输出"=w1213:string)  [unwired: 7 in]
              n405 = call "核查数据编码整合输出.vi"("字段结束"=FALSE, "数据标识"="N" ("字符串"), "数据类型"="-Check=", "污染物编码"="w21001", "数据值"=w1140) -> ("编码输出"=w1121:string)  [unwired: 6 in]
              n406 = call "核查数据编码整合输出.vi"("字段结束"=FALSE, "数据标识"="N" ("字符串"), "数据类型"="-Water=", "污染物编码"="w21001", "数据值"=w1125) -> ("编码输出"=w1119:string)  [unwired: 6 in]
              n407 = call "核查数据编码整合输出.vi"("字段结束"=FALSE, "数据标识"="N" ("字符串"), "数据类型"="-Chroma=", "污染物编码"="w21001", "数据值"=w1124) -> ("编码输出"=w1118:string)  [unwired: 6 in]
              n408 = call "核查数据编码整合输出.vi"("字段结束"=FALSE, "数据标识"="N" ("字符串"), "数据类型"="-Volume=", "污染物编码"="w21001", "数据值"=w1123) -> ("编码输出"=w1117:string)  [unwired: 6 in]
              n409 = call "核查数据编码整合输出.vi"("字段结束"=TRUE, "数据标识"="N" ("字符串"), "数据类型"="-DVolume=", "污染物编码"="w21001", "数据值"=w1122) -> ("编码输出"=w1116:string)  [unwired: 6 in]
              n410 = call "核查数据编码整合输出.vi"("字段结束"=TRUE, "数据类型"="-DVolume=", "污染物编码"="w01019", "数据值"=w1220) -> ("编码输出"=w1212:string)  [unwired: 7 in]
              n411 = call "核查数据编码整合输出.vi"("字段结束"=FALSE, "数据类型"="-Chroma=", "污染物编码"="w01019", "数据值"=w1225) -> ("编码输出"=w1214:string)  [unwired: 7 in]
              n412 = call "核查数据编码整合输出.vi"("字段结束"=FALSE, "数据标识"="N" ("字符串"), "数据类型"="-Check=", "污染物编码"="w21003", "数据值"=w1210) -> ("编码输出"=w1181:string)  [unwired: 6 in]
              n413 = call "核查数据编码整合输出.vi"("字段结束"=FALSE, "数据标识"="N" ("字符串"), "数据类型"="-WaterTime=", "污染物编码"="w21003", "数据值"=w1037) -> ("编码输出"=w1180:string)  [unwired: 6 in]
              n414 = call "核查数据编码整合输出.vi"("字段结束"=FALSE, "数据标识"="N" ("字符串"), "数据类型"="-Check=", "污染物编码"="w01019", "数据值"=w1236) -> ("编码输出"=w1217:string)  [unwired: 6 in]
              n415 = call "核查数据编码整合输出.vi"("字段结束"=FALSE, "数据类型"="-WaterTime=", "污染物编码"="w01019", "数据值"=w1059) -> ("编码输出"=w1216:string)  [unwired: 7 in]
              n416 = call "核查数据编码整合输出.vi"("字段结束"=FALSE, "数据标识"="N" ("字符串"), "数据类型"="-Water=", "污染物编码"="w21003", "数据值"=w1190) -> ("编码输出"=w1179:string)  [unwired: 6 in]
              n417 = call "核查数据编码整合输出.vi"("字段结束"=FALSE, "数据类型"="-Water=", "污染物编码"="w01019", "数据值"=w1228) -> ("编码输出"=w1215:string)  [unwired: 7 in]
              n418 = call "核查数据编码整合输出.vi"("字段结束"=FALSE, "数据标识"="N" ("字符串"), "数据类型"="-Chroma=", "污染物编码"="w21003", "数据值"=w1189) -> ("编码输出"=w1178:string)  [unwired: 6 in]
              n419 = call "核查数据编码整合输出.vi"("字段结束"=FALSE, "数据标识"="N" ("字符串"), "数据类型"="-Volume=", "污染物编码"="w21003", "数据值"=w1188) -> ("编码输出"=w1177:string)  [unwired: 6 in]
              n420 = call "核查数据编码整合输出.vi"("字段结束"=TRUE, "数据标识"="N" ("字符串"), "数据类型"="-DVolume=", "污染物编码"="w21003", "数据值"=w1187) -> ("编码输出"=w1176:string)  [unwired: 6 in]
              n421 = call "核查数据编码整合输出.vi"("字段结束"=FALSE, "数据标识"="N" ("字符串"), "数据类型"="-Check=", "污染物编码"="w01018", "数据值"=w1138) -> ("编码输出"=w1093:string)  [unwired: 6 in]
              n422 = call "核查数据编码整合输出.vi"("字段结束"=FALSE, "数据标识"="N" ("字符串"), "数据类型"="-Water=", "污染物编码"="w01018", "数据值"=w1075) -> ("编码输出"=w1091:string)  [unwired: 6 in]
              n423 = call "核查数据编码整合输出.vi"("字段结束"=FALSE, "数据标识"="N" ("字符串"), "数据类型"="-WaterTime=", "污染物编码"="w01018", "数据值"=w1031) -> ("编码输出"=w1092:string)  [unwired: 6 in]
              n424 = call "核查数据编码整合输出.vi"("字段结束"=FALSE, "数据标识"="N" ("字符串"), "数据类型"="-Chroma=", "污染物编码"="w01018", "数据值"=w1076) -> ("编码输出"=w1090:string)  [unwired: 6 in]
              n425 = call "核查数据编码整合输出.vi"("字段结束"=FALSE, "数据标识"="N" ("字符串"), "数据类型"="-Volume=", "污染物编码"="w01018", "数据值"=w1077) -> ("编码输出"=w1089:string)  [unwired: 6 in]
              n426 = call "核查数据编码整合输出.vi"("字段结束"=TRUE, "数据标识"="N" ("字符串"), "数据类型"="-DVolume=", "污染物编码"="w01018", "数据值"=w1078) -> ("编码输出"=w1088:string)  [unwired: 6 in]
              n427 = Concatenate Strings(w1167, w1150, w1149, w1148, w1147, w1146) -> (w1136:string)
              n428 = Concatenate Strings(w1217, w1216, w1215, w1214, w1213, w1212) -> (w1211:string)
              n429 = Concatenate Strings(w1181, w1180, w1179, w1178, w1177, w1176) -> (w1175:string)
              n430 = Concatenate Strings(w1121, w1120, w1119, w1118, w1117, w1116) -> (w1071:string)
              n431 = Empty String/Path?(string/path=w1247) -> (empty?=w1238:bool)
              n432 = Concatenate Strings(w1093, w1092, w1091, w1090, w1089, w1088) -> (w1070:string)
              n433 = Format Into String(format string="DataTime=%s;%s%s%s%s%s" ("格式字符串"), w1247, w1211, w1175, w1136, w1071, w1070) -> (resulting string=w1240:string)  [unwired: 2 in, 1 out]
              n434 = case shown="真" w1238 {
                tunnel: [w1259 ""] -> w1239
                tunnel: w1240 -> [w1259 _]
                frame False {
                  n435 = global read "全局 小时数据发送次数.vi" "小时数据发送次数"() -> (w1258:i32)
                  n436 = Increment(x=w1258) -> (x+1=w1257:i32)
                  n437 = global write "全局 小时数据发送次数.vi" "小时数据发送次数"(w1257) -> ()
                }
                frame True {
                  n438 = global read "全局 小时数据发送次数.vi" "小时数据发送次数"() -> (w1261:i32)
                  n439 = Increment(x=w1261) -> (x+1=w1260:i32)
                  n440 = global write "全局 小时数据发送次数.vi" "小时数据发送次数"(w1260) -> ()
                }
              }
            }
            frame "返回执行结果" {
            }
          }
        }
        frame "核查数据" {
          n441 = global read "全局1.vi" "枚举"() -> (w1273:enum16{"返回请求应答", "上传数据", "返回执行结果"})
          n442 = case shown="\"上传数据\"" w1273 {
            tunnel: ["QnRtn=1" w1297 "ExeRtn=1"] -> w1274
            tunnel: w1272 -> [_ w1295 _]
            tunnel: w1271 -> [_ w1294 _]
            tunnel: w1270 -> [_ w1291 _]
            tunnel: w1269 -> [_ w1283 _]
            tunnel: w1268 -> [_ w1282 _]
            tunnel: w1267 -> [_ w1281 _]
            tunnel: w1266 -> [_ w1280 _]
            tunnel: w1265 -> [_ w1279 _]
            tunnel: w1264 -> [_ w1278 _]
            frame "返回请求应答", Default {
            }
            frame "上传数据" {
              # "将非空数组的时间戳写入"
              n443 = global read "全局 小时数据发送次数.vi" "小时数据发送次数"() -> (w1289:i32)
              n444 = Index Array(array=w1295, index (row)=w1289) -> (element=w1296:string[])  [unwired: 1 in]
              n445 = Index Array(array=w1294, index (row)=w1289) -> (element=w1293:string[])  [unwired: 1 in]
              n446 = Index Array(array=w1291, index (row)=w1289) -> (element=w1292:string[])  [unwired: 1 in]
              n447 = Index Array(array=w1283, index (row)=w1289) -> (element=w1290:string[])  [unwired: 1 in]
              n448 = Index Array(array=w1282, index (row)=w1289) -> (element=w1284:string[])  [unwired: 1 in]
              n449 = Index Array(array=w1281, index (row)=w1289) -> (element=w1285:string[])  [unwired: 1 in]
              n450 = Index Array(array=w1280, index (row)=w1289) -> (element=w1286:string[])  [unwired: 1 in]
              n451 = Index Array(array=w1279, index (row)=w1289) -> (element=w1287:string[])  [unwired: 1 in]
              n452 = Index Array(array=w1278, index (row)=w1289) -> (element=w1288:string[])  [unwired: 1 in]
              n453 = Index Array(array=w1296, index #1=0 ("索引"), index #2=3 ("索引"), index #3=7 ("索引")) -> (element #1=w1277:string, element #2=w1336:string, element #3=w1335:string)
              n454 = Index Array(array=w1293, index #1=0 ("索引"), index #2=3 ("索引"), index #3=7 ("索引")) -> (element #2=w1333:string, element #3=w1332:string)  [unwired: 1 out]
              n455 = Index Array(array=w1290, index #1=0 ("索引"), index #2=3 ("索引"), index #3=7 ("索引")) -> (element #2=w1327:string, element #3=w1326:string)  [unwired: 1 out]
              n456 = Index Array(array=w1284, index #1=0 ("索引"), index #2=3 ("索引"), index #3=7 ("索引")) -> (element #2=w1322:string, element #3=w1324:string)  [unwired: 1 out]
              n457 = Index Array(array=w1285, index #1=0 ("索引"), index #2=3 ("索引"), index #3=7 ("索引")) -> (element #2=w1318:string, element #3=w1317:string)  [unwired: 1 out]
              n458 = Index Array(array=w1292, index #1=0 ("索引"), index #2=3 ("索引"), index #3=7 ("索引")) -> (element #2=w1329:string, element #3=w1328:string)  [unwired: 1 out]
              n459 = Index Array(array=w1288, index #1=0 ("索引"), index #2=3 ("索引"), index #3=7 ("索引")) -> (element #2=w1302:string, element #3=w1303:string)  [unwired: 1 out]
              n460 = Index Array(array=w1286, index #1=0 ("索引"), index #2=3 ("索引"), index #3=7 ("索引")) -> (element #2=w1312:string, element #3=w1313:string)  [unwired: 1 out]
              n461 = Index Array(array=w1287, index #1=0 ("索引"), index #2=3 ("索引"), index #3=7 ("索引")) -> (element #2=w1308:string, element #3=w1307:string)  [unwired: 1 out]
              n462 = case shown="\"真\", 默认" w1302 {
                tunnel: [w1355 w1365] -> w1298
                tunnel: w1302 -> [w1355 w1359]
                tunnel: w1303 -> [_ w1358]
                frame "" {
                }
                frame "真", Default {
                  n463 = call "核查数据编码整合输出.vi"("字段结束"=FALSE, "数据标识"="N" ("字符串"), "数据类型"="-Check=", "污染物编码"="w01003", "数据值"=w1359) -> ("编码输出"=w1366:string)  [unwired: 6 in]
                  n464 = call "核查数据编码整合输出.vi"("字段结束"=TRUE, "数据标识"="N" ("字符串"), "数据类型"="-StandardValue=", "污染物编码"="w01003", "数据值"=w1358) -> ("编码输出"=w1362:string)  [unwired: 6 in]
                  n465 = Concatenate Strings(w1366, w1362) -> (w1365:string)
                }
              }
              n466 = case shown="\"真\", 默认" w1312 {
                tunnel: w1312 -> [w1383 w1395]
                tunnel: [w1383 w1392] -> w1300
                tunnel: w1313 -> [_ w1388]
                frame "" {
                }
                frame "真", Default {
                  n467 = call "核查数据编码整合输出.vi"("字段结束"=FALSE, "数据标识"="N" ("字符串"), "数据类型"="-Check=", "污染物编码"="w01009", "数据值"=w1395) -> ("编码输出"=w1393:string)  [unwired: 6 in]
                  n468 = call "核查数据编码整合输出.vi"("字段结束"=TRUE, "数据标识"="N" ("字符串"), "数据类型"="-StandardValue=", "污染物编码"="w01009", "数据值"=w1388) -> ("编码输出"=w1389:string)  [unwired: 6 in]
                  n469 = Concatenate Strings(w1393, w1389) -> (w1392:string)
                }
              }
              n470 = case shown="\"真\", 默认" w1308 {
                tunnel: [w1369 w1379] -> w1299
                tunnel: w1308 -> [w1369 w1371]
                tunnel: w1307 -> [_ w1370]
                frame "" {
                }
                frame "真", Default {
                  n471 = call "核查数据编码整合输出.vi"("字段结束"=FALSE, "数据标识"="N" ("字符串"), "数据类型"="-Check=", "污染物编码"="w01014", "数据值"=w1371) -> ("编码输出"=w1380:string)  [unwired: 6 in]
                  n472 = call "核查数据编码整合输出.vi"("字段结束"=TRUE, "数据标识"="N" ("字符串"), "数据类型"="-StandardValue=", "污染物编码"="w01014", "数据值"=w1370) -> ("编码输出"=w1376:string)  [unwired: 6 in]
                  n473 = Concatenate Strings(w1380, w1376) -> (w1379:string)
                }
              }
              n474 = case shown="\"真\", 默认" w1318 {
                tunnel: w1318 -> [w1397 w1409]
                tunnel: [w1397 w1406] -> w1301
                tunnel: w1317 -> [_ w1402]
                frame "" {
                }
                frame "真", Default {
                  n475 = call "核查数据编码整合输出.vi"("字段结束"=FALSE, "数据标识"="N" ("字符串"), "数据类型"="-Check=", "污染物编码"="w01001", "数据值"=w1409) -> ("编码输出"=w1407:string)  [unwired: 6 in]
                  n476 = call "核查数据编码整合输出.vi"("字段结束"=TRUE, "数据标识"="N" ("字符串"), "数据类型"="-StandardValue=", "污染物编码"="w01001", "数据值"=w1402) -> ("编码输出"=w1403:string)  [unwired: 6 in]
                  n477 = Concatenate Strings(w1407, w1403) -> (w1406:string)
                }
              }
              n478 = case shown="\"真\", 默认" w1336 {
                tunnel: w1336 -> [w1467 w1479]
                tunnel: [w1467 w1475] -> w1334
                tunnel: w1335 -> [_ w1470]
                frame "" {
                }
                frame "真", Default {
                  # "CODMn"
                  n479 = call "核查数据编码整合输出.vi"("字段结束"=FALSE, "数据标识"="N" ("字符串"), "数据类型"="-Check=", "污染物编码"="w01019", "数据值"=w1479) -> ("编码输出"=w1476:string)  [unwired: 6 in]
                  n480 = call "核查数据编码整合输出.vi"("字段结束"=TRUE, "数据标识"="N" ("字符串"), "数据类型"="-StandardValue=", "污染物编码"="w01019", "数据值"=w1470) -> ("编码输出"=w1471:string)  [unwired: 6 in]
                  n481 = Concatenate Strings(w1476, w1471) -> (w1475:string)
                }
              }
              n482 = case shown="\"真\", 默认" w1322 {
                tunnel: w1322 -> [w1411 w1423]
                tunnel: [w1411 w1420] -> w1323
                tunnel: w1324 -> [_ w1416]
                frame "" {
                }
                frame "真", Default {
                  n483 = call "核查数据编码整合输出.vi"("字段结束"=FALSE, "数据标识"="N" ("字符串"), "数据类型"="-Check=", "污染物编码"="w01018", "数据值"=w1423) -> ("编码输出"=w1421:string)  [unwired: 6 in]
                  n484 = call "核查数据编码整合输出.vi"("字段结束"=TRUE, "数据标识"="N" ("字符串"), "数据类型"="-StandardValue=", "污染物编码"="w01018", "数据值"=w1416) -> ("编码输出"=w1417:string)  [unwired: 6 in]
                  n485 = Concatenate Strings(w1421, w1417) -> (w1420:string)
                }
              }
              n486 = case shown="\"真\", 默认" w1333 {
                tunnel: w1333 -> [w1453 w1465]
                tunnel: [w1453 w1462] -> w1331
                tunnel: w1332 -> [_ w1458]
                frame "" {
                }
                frame "真", Default {
                  n487 = call "核查数据编码整合输出.vi"("字段结束"=FALSE, "数据标识"="N" ("字符串"), "数据类型"="-Check=", "污染物编码"="w21003", "数据值"=w1465) -> ("编码输出"=w1463:string)  [unwired: 6 in]
                  n488 = call "核查数据编码整合输出.vi"("字段结束"=TRUE, "数据标识"="N" ("字符串"), "数据类型"="-StandardValue=", "污染物编码"="w21003", "数据值"=w1458) -> ("编码输出"=w1459:string)  [unwired: 6 in]
                  n489 = Concatenate Strings(w1463, w1459) -> (w1462:string)
                }
              }
              n490 = case shown="\"真\", 默认" w1329 {
                tunnel: w1329 -> [w1439 w1451]
                tunnel: [w1439 w1448] -> w1330
                tunnel: w1328 -> [_ w1444]
                frame "" {
                }
                frame "真", Default {
                  n491 = call "核查数据编码整合输出.vi"("字段结束"=FALSE, "数据标识"="N" ("字符串"), "数据类型"="-Check=", "污染物编码"="w21011", "数据值"=w1451) -> ("编码输出"=w1449:string)  [unwired: 6 in]
                  n492 = call "核查数据编码整合输出.vi"("字段结束"=TRUE, "数据标识"="N" ("字符串"), "数据类型"="-StandardValue=", "污染物编码"="w21011", "数据值"=w1444) -> ("编码输出"=w1445:string)  [unwired: 6 in]
                  n493 = Concatenate Strings(w1449, w1445) -> (w1448:string)
                }
              }
              n494 = case shown="\"真\", 默认" w1327 {
                tunnel: w1327 -> [w1425 w1437]
                tunnel: [w1425 w1434] -> w1325
                tunnel: w1326 -> [_ w1430]
                frame "" {
                }
                frame "真", Default {
                  n495 = call "核查数据编码整合输出.vi"("字段结束"=FALSE, "数据标识"="N" ("字符串"), "数据类型"="-Check=", "污染物编码"="w21001", "数据值"=w1437) -> ("编码输出"=w1435:string)  [unwired: 6 in]
                  n496 = call "核查数据编码整合输出.vi"("字段结束"=TRUE, "数据标识"="N" ("字符串"), "数据类型"="-StandardValue=", "污染物编码"="w21001", "数据值"=w1430) -> ("编码输出"=w1431:string)  [unwired: 6 in]
                  n497 = Concatenate Strings(w1435, w1431) -> (w1434:string)
                }
              }
              n498 = call "规范小时时间戳.vi"("字符串"=w1277) -> ("result string"=w1276:string)  [unwired: 10 in]
              n499 = Format Into String(format string="DataTime=%s;%s%s%s%s%s%s%s%s%s" ("格式字符串"), w1276, w1334, w1331, w1330, w1325, w1323, w1301, w1300, w1299, w1298) -> (resulting string=w1337:string)  [unwired: 2 in, 1 out]
              n500 = Empty String/Path?(string/path=w1276) -> (empty?=w1338:bool)
              n501 = case shown="假" w1338 {
                tunnel: [w1483 ""] -> w1297
                tunnel: w1337 -> [w1483 _]
                frame False {
                  n502 = global read "全局 小时数据发送次数.vi" "小时数据发送次数"() -> (w1482:i32)
                  n503 = Increment(x=w1482) -> (x+1=w1481:i32)
                  n504 = global write "全局 小时数据发送次数.vi" "小时数据发送次数"(w1481) -> ()
                }
                frame True {
                  n505 = global read "全局 小时数据发送次数.vi" "小时数据发送次数"() -> (w1485:i32)
                  n506 = Increment(x=w1485) -> (x+1=w1484:i32)
                  n507 = global write "全局 小时数据发送次数.vi" "小时数据发送次数"(w1484) -> ()
                }
              }
            }
            frame "返回执行结果" {
            }
          }
        }
        frame "空白测试", "跨度核查" {
          n508 = global read "全局1.vi" "枚举"() -> (w1493:enum16{"返回请求应答", "上传数据", "返回执行结果"})
          n509 = case shown="\"上传数据\"" w1493 {
            tunnel: ["QnRtn=1" w1510 "ExeRtn=1"] -> w1494
            tunnel: w1492 -> [_ w1516 _]
            tunnel: w1491 -> [_ w1515 _]
            tunnel: w1490 -> [_ w1514 _]
            tunnel: w1489 -> [_ w1513 _]
            tunnel: w1488 -> [_ w1512 _]
            frame "返回请求应答", Default {
            }
            frame "上传数据" {
              n510 = global read "全局 小时数据发送次数.vi" "小时数据发送次数"() -> (w1503:i32)
              n511 = global read "全局 小时数据发送次数.vi" "小时数据发送次数"() -> (w1504:i32)
              n512 = global read "全局 小时数据发送次数.vi" "小时数据发送次数"() -> (w1507:i32)
              n513 = global read "全局 小时数据发送次数.vi" "小时数据发送次数"() -> (w1506:i32)
              n514 = global read "全局 小时数据发送次数.vi" "小时数据发送次数"() -> (w1505:i32)
              n515 = Index Array(array=w1515, index (row)=w1504) -> (element=w1540:string[])  [unwired: 1 in]
              n516 = Index Array(array=w1516, index (row)=w1503) -> (element=w1538:string[])  [unwired: 1 in]
              n517 = Index Array(array=w1513, index (row)=w1507) -> (element=w1534:string[])  [unwired: 1 in]
              n518 = Index Array(array=w1512, index (row)=w1506) -> (element=w1533:string[])  [unwired: 1 in]
              n519 = Index Array(array=w1514, index (row)=w1505) -> (element=w1537:string[])  [unwired: 1 in]
              n520 = Index Array(array=w1540, index #1=3 ("索引"), index #2=7 ("索引")) -> (element #1=w1501:string, element #2=w1528:string)
              n521 = Index Array(array=w1538, index #1=0 ("索引"), index #2=3 ("索引"), index #3=7 ("索引")) -> (element #1=w1497:string, element #2=w1502:string, element #3=w1508:string)
              n522 = Index Array(array=w1534, index #1=3 ("索引"), index #2=7 ("索引")) -> (element #1=w1499:string, element #2=w1523:string)
              n523 = Index Array(array=w1533, index #1=3 ("索引"), index #2=7 ("索引")) -> (element #1=w1498:string, element #2=w1521:string)
              n524 = Index Array(array=w1537, index #1=3 ("索引"), index #2=7 ("索引")) -> (element #1=w1500:string, element #2=w1525:string)
              n525 = case shown="\"真\", 默认" w1499 {
                tunnel: w1499 -> [w1566 w1578]
                tunnel: w1523 -> [_ w1577]
                tunnel: [w1566 w1576] -> w1519
                frame "" {
                }
                frame "真", Default {
                  # "总氮"
                  n526 = call "核查数据编码整合输出.vi"("字段结束"=TRUE, "数据标识"="N" ("字符串"), "数据类型"="-SpanValue=", "污染物编码"="w21001", "数据精度"=3 ("精度"), "数据值"="0") -> ("编码输出"=w1568:string)  [unwired: 5 in]
                  n527 = call "核查数据编码整合输出.vi"("字段结束"=FALSE, "数据标识"="N" ("字符串"), "数据类型"="-StandardValue=", "污染物编码"="w21001", "数据精度"=3 ("精度"), "数据值"=w1577) -> ("编码输出"=w1580:string)  [unwired: 5 in]
                  n528 = call "核查数据编码整合输出.vi"("字段结束"=FALSE, "数据标识"="N" ("字符串"), "数据类型"="-Check=", "污染物编码"="w21001", "数据精度"=3 ("精度"), "数据值"=w1578) -> ("编码输出"=w1579:string)  [unwired: 5 in]
                  n529 = Concatenate Strings(w1579, w1580, w1568) -> (w1576:string)
                }
              }
              n530 = case shown="\"真\", 默认" w1500 {
                tunnel: w1500 -> [w1589 w1601]
                tunnel: w1525 -> [_ w1600]
                tunnel: [w1589 w1599] -> w1520
                frame "" {
                }
                frame "真", Default {
                  # "总磷"
                  n531 = call "核查数据编码整合输出.vi"("字段结束"=TRUE, "数据标识"="N" ("字符串"), "数据类型"="-SpanValue=", "污染物编码"="w21011", "数据精度"=3 ("精度"), "数据值"="0") -> ("编码输出"=w1594:string)  [unwired: 5 in]
                  n532 = call "核查数据编码整合输出.vi"("字段结束"=FALSE, "数据标识"="N" ("字符串"), "数据类型"="-StandardValue=", "污染物编码"="w21011", "数据精度"=3 ("精度"), "数据值"=w1600) -> ("编码输出"=w1610:string)  [unwired: 5 in]
                  n533 = call "核查数据编码整合输出.vi"("字段结束"=FALSE, "数据标识"="N" ("字符串"), "数据类型"="-Check=", "污染物编码"="w21011", "数据精度"=3 ("精度"), "数据值"=w1601) -> ("编码输出"=w1611:string)  [unwired: 5 in]
                  n534 = Concatenate Strings(w1611, w1610, w1594) -> (w1599:string)
                }
              }
              n535 = case shown="\"真\", 默认" w1502 {
                tunnel: w1502 -> [w1635 w1653]
                tunnel: [w1635 w1649] -> w1530
                tunnel: w1508 -> [_ w1641]
                frame "" {
                }
                frame "真", Default {
                  # "CODMn"
                  n536 = call "核查数据编码整合输出.vi"("字段结束"=FALSE, "数据标识"="N" ("字符串"), "数据类型"="-Check=", "污染物编码"="w01019", "数据值"=w1653) -> ("编码输出"=w1650:string)  [unwired: 6 in]
                  n537 = call "核查数据编码整合输出.vi"("字段结束"=FALSE, "数据标识"="N" ("字符串"), "数据类型"="-StandardValue=", "污染物编码"="w01019", "数据值"=w1641) -> ("编码输出"=w1645:string)  [unwired: 6 in]
                  n538 = call "核查数据编码整合输出.vi"("字段结束"=TRUE, "数据标识"="N" ("字符串"), "数据类型"="-SpanValue=", "污染物编码"="w01019", "数据值"="0") -> ("编码输出"=w1640:string)  [unwired: 6 in]
                  n539 = Concatenate Strings(w1650, w1645, w1640) -> (w1649:string)
                }
              }
              n540 = case shown="\"真\", 默认" w1501 {
                tunnel: w1501 -> [w1612 w1626]
                tunnel: w1528 -> [_ w1625]
                tunnel: [w1612 w1622] -> w1527
                frame "" {
                }
                frame "真", Default {
                  # "NH3"
                  n541 = call "核查数据编码整合输出.vi"("字段结束"=FALSE, "数据标识"="N" ("字符串"), "数据类型"="-Check=", "污染物编码"="w21003", "数据精度"=3 ("精度"), "数据值"=w1626) -> ("编码输出"=w1623:string)  [unwired: 5 in]
                  n542 = call "核查数据编码整合输出.vi"("字段结束"=FALSE, "数据标识"="N" ("字符串"), "数据类型"="-StandardValue=", "污染物编码"="w21003", "数据精度"=3 ("精度"), "数据值"=w1625) -> ("编码输出"=w1624:string)  [unwired: 5 in]
                  n543 = call "核查数据编码整合输出.vi"("字段结束"=TRUE, "数据标识"="N" ("字符串"), "数据类型"="-SpanValue=", "污染物编码"="w21003", "数据精度"=3 ("精度"), "数据值"="0") -> ("编码输出"=w1615:string)  [unwired: 5 in]
                  n544 = Concatenate Strings(w1623, w1624, w1615) -> (w1622:string)
                }
              }
              n545 = case shown="\"真\", 默认" w1498 {
                tunnel: w1498 -> [w1543 w1555]
                tunnel: w1521 -> [_ w1554]
                tunnel: [w1543 w1553] -> w1518
                frame "" {
                }
                frame "真", Default {
                  # "CODCr"
                  n546 = call "核查数据编码整合输出.vi"("字段结束"=TRUE, "数据标识"="N" ("字符串"), "数据类型"="-SpanValue=", "污染物编码"="w01018", "数据精度"=3 ("精度"), "数据值"="0") -> ("编码输出"=w1545:string)  [unwired: 5 in]
                  n547 = call "核查数据编码整合输出.vi"("字段结束"=FALSE, "数据标识"="N" ("字符串"), "数据类型"="-StandardValue=", "污染物编码"="w01018", "数据精度"=3 ("精度"), "数据值"=w1554) -> ("编码输出"=w1564:string)  [unwired: 5 in]
                  n548 = call "核查数据编码整合输出.vi"("字段结束"=FALSE, "数据标识"="N" ("字符串"), "数据类型"="-Check=", "污染物编码"="w01018", "数据精度"=3 ("精度"), "数据值"=w1555) -> ("编码输出"=w1565:string)  [unwired: 5 in]
                  n549 = Concatenate Strings(w1565, w1564, w1545) -> (w1553:string)
                }
              }
              n550 = call "规范小时时间戳.vi"("字符串"=w1497) -> ("result string"=w1496:string)  [unwired: 10 in]
              n551 = Format Into String(format string="DataTime=%s;%s%s%s%s%s" ("格式字符串"), w1496, w1530, w1527, w1520, w1519, w1518) -> (resulting string=w1509:string)  [unwired: 2 in, 1 out]
              n552 = Empty String/Path?(string/path=w1496) -> (empty?=w1511:bool)
              n553 = case shown="假" w1511 {
                tunnel: [w1655 ""] -> w1510
                tunnel: w1509 -> [w1655 _]
                frame False {
                  n554 = global read "全局 小时数据发送次数.vi" "小时数据发送次数"() -> (w1657:i32)
                  n555 = Increment(x=w1657) -> (x+1=w1656:i32)
                  n556 = global write "全局 小时数据发送次数.vi" "小时数据发送次数"(w1656) -> ()
                }
                frame True {
                  n557 = global read "全局 小时数据发送次数.vi" "小时数据发送次数"() -> (w1659:i32)
                  n558 = Increment(x=w1659) -> (x+1=w1658:i32)
                  n559 = global write "全局 小时数据发送次数.vi" "小时数据发送次数"(w1658) -> ()
                }
              }
            }
            frame "返回执行结果" {
            }
          }
        }
      }
    }
    frame "小时数据" {
      # "藻密度"
      # "叶绿素"
      # "浊度"
      # "水温"
      # "发送小时数据"
      n560 = global read "全局流量数据小时.vi" "累积流量"() -> (w1665:string[][])
      n561 = global read "全局流量数据小时.vi" "瞬时流量"() -> (w1664:string[][])
      n562 = global read "全局流量数据小时.vi" "流速"() -> (w1663:string[][])
      n563 = global read "全局流量数据小时.vi" "水位"() -> (w1662:string[][])
      n564 = global read "全局 小时数据发送次数.vi" "小时数据发送次数"() -> (w1689:i32)
      n565 = global read "全局 小时数据发送次数.vi" "小时数据发送次数"() -> (w1690:i32)
      n566 = global read "全局 小时数据发送次数.vi" "小时数据发送次数"() -> (w1677:i32)
      n567 = global read "全局 小时数据发送次数.vi" "小时数据发送次数"() -> (w1673:i32)
      n568 = global read "全局 小时数据发送次数.vi" "小时数据发送次数"() -> (w1693:i32)
      n569 = global read "全局 小时数据发送次数.vi" "小时数据发送次数"() -> (w1672:i32)
      n570 = global read "全局 小时数据发送次数.vi" "小时数据发送次数"() -> (w1671:i32)
      n571 = global read "全局 小时数据发送次数.vi" "小时数据发送次数"() -> (w1670:i32)
      n572 = global read "全局 小时数据发送次数.vi" "小时数据发送次数"() -> (w1679:i32)
      n573 = global read "全局 小时数据发送次数.vi" "小时数据发送次数"() -> (w1699:i32)
      n574 = global read "全局 小时数据发送次数.vi" "小时数据发送次数"() -> (w1685:i32)
      n575 = global read "全局 小时数据发送次数.vi" "小时数据发送次数"() -> (w1697:i32)
      n576 = global read "全局 小时数据发送次数.vi" "小时数据发送次数"() -> (w1682:i32)
      n577 = global read "全局 小时数据发送次数.vi" "小时数据发送次数"() -> (w1701:i32)
      n578 = global read "全局 小时数据发送次数.vi" "小时数据发送次数"() -> (w1687:i32)
      n579 = global read "全局 小时数据发送次数.vi" "小时数据发送次数"() -> (w1695:i32)
      n580 = global read "全局 小时数据发送次数.vi" "小时数据发送次数"() -> (w1683:i32)
      n581 = global read "全局 小时数据发送次数.vi" "小时数据发送次数"() -> (w1703:i32)
      n582 = Index Array(array=w1710, index (row)=w1690) -> (element=w1691:string[])  [unwired: 1 in]
      n583 = Index Array(array=w1674, index (row)=w1677) -> (element=w1676:string[])  [unwired: 1 in]
      n584 = Index Array(array=w1662, index (row)=w1673) -> (element=w1669:string[])  [unwired: 1 in]
      n585 = Index Array(array=w1711, index (row)=w1693) -> (element=w1692:string[])  [unwired: 1 in]
      n586 = Index Array(array=w1663, index (row)=w1672) -> (element=w1668:string[])  [unwired: 1 in]
      n587 = Index Array(array=w1664, index (row)=w1671) -> (element=w1667:string[])  [unwired: 1 in]
      n588 = Index Array(array=w1665, index (row)=w1670) -> (element=w1666:string[])  [unwired: 1 in]
      n589 = Index Array(array=w1675, index (row)=w1679) -> (element=w1678:string[])  [unwired: 1 in]
      n590 = Index Array(array=w1715, index (row)=w1701) -> (element=w1700:string[])  [unwired: 1 in]
      n591 = Index Array(array=w1714, index (row)=w1699) -> (element=w1698:string[])  [unwired: 1 in]
      n592 = Index Array(array=w1713, index (row)=w1697) -> (element=w1696:string[])  [unwired: 1 in]
      n593 = Index Array(array=w1716, index (row)=w1703) -> (element=w1702:string[])  [unwired: 1 in]
      n594 = Index Array(array=w1709, index (row)=w1689) -> (element=w1688:string[])  [unwired: 1 in]
      n595 = Index Array(array=w1707, index (row)=w1685) -> (element=w1684:string[])  [unwired: 1 in]
      n596 = Index Array(array=w1708, index (row)=w1687) -> (element=w1686:string[])  [unwired: 1 in]
      n597 = Index Array(array=w1712, index (row)=w1695) -> (element=w1694:string[])  [unwired: 1 in]
      n598 = Index Array(array=w1705, index (row)=w1682) -> (element=w1680:string[])  [unwired: 1 in]
      n599 = Index Array(array=w1706, index (row)=w1683) -> (element=w1681:string[])  [unwired: 1 in]
      n600 = global read "全局1.vi" "枚举"() -> (w1704:enum16{"返回请求应答", "上传数据", "返回执行结果"})
      n601 = case shown="\"上传数据\"" w1704 {
        tunnel: ["QnRtn=1" w1783 "ExeRtn=1"] -> w1717
        tunnel: w1702 -> [_ w1810 _]
        tunnel: w1698 -> [_ w1824 _]
        tunnel: w1696 -> [_ w1823 _]
        tunnel: w1694 -> [_ w1822 _]
        tunnel: w1700 -> [_ w1820 _]
        tunnel: w1692 -> [_ w1809 _]
        tunnel: w1691 -> [_ w1815 _]
        tunnel: w1688 -> [_ w1812 _]
        tunnel: w1686 -> [_ w1811 _]
        tunnel: w1684 -> [_ w1808 _]
        tunnel: w1681 -> [_ w1807 _]
        tunnel: w1680 -> [_ w1806 _]
        tunnel: w1678 -> [_ w1788 _]
        tunnel: w1676 -> [_ w1787 _]
        tunnel: w1669 -> [_ w1782 _]
        tunnel: w1668 -> [_ w1781 _]
        tunnel: w1667 -> [_ w1780 _]
        tunnel: w1666 -> [_ w1779 _]
        frame "返回请求应答", Default {
          (unwired) 0 ("当前包数")
          n602 = global read "全局 数据数组大小.vi" "数据数组大小"() -> (w1718:i32)
          n603 = global write "全局1.vi" "枚举"(enum16{"返回请求应答", "上传数据", "返回执行结果"}."上传数据" ("枚举")) -> ()
          n604 = Equal To 0?(x=w1718) -> (x = 0?=w1719:bool)
          n605 = case shown="真" w1719 {
            frame False {
            }
            frame True {
              n606 = global read "全局 小时数据发送次数.vi" "小时数据发送次数"() -> (w1723:i32)
              n607 = Increment(x=w1723) -> (x+1=w1722:i32)
              n608 = global write "全局 小时数据发送次数.vi" "小时数据发送次数"(w1722) -> ()
            }
          }
        }
        frame "上传数据" {
          (unwired) 2 ("数据精度")
          (unwired) 3 ("数据精度")
          (unwired) 3 ("数据精度")
          (unwired) 3 ("数据精度")
          # "PH"
          # "总氮"
          # "总磷"
          # "CODCr"
          # "NH3"
          n609 = global read "断电保存全局.vi" "数据发送协议"() -> (w1730:enum16{"2005-212协议", "2017-212协议"})
          n610 = global read "断电保存全局.vi" "数据发送协议"() -> (w1727:enum16{"2005-212协议", "2017-212协议"})
          n611 = global read "断电保存全局.vi" "数据发送协议"() -> (w1728:enum16{"2005-212协议", "2017-212协议"})
          n612 = global read "断电保存全局.vi" "数据发送协议"() -> (w1729:enum16{"2005-212协议", "2017-212协议"})
          n613 = case shown="\"2017-212协议\", 默认" w1727 {
            tunnel: w1788 -> [_ w1977]
            tunnel: w1787 -> [_ w1976]
            tunnel: [w1931 w1975] -> w1786
            tunnel: [w1931 w1974] -> w1785
            tunnel: w1782 -> [_ w1961]
            tunnel: w1781 -> [_ w1960]
            tunnel: w1780 -> [_ w1959]
            tunnel: w1779 -> [_ w1958]
            tunnel: [w1931 w1957] -> w1778
            tunnel: [w1931 w1956] -> w1777
            tunnel: [w1931 w1955] -> w1776
            tunnel: [w1931 w1954] -> w1775
            frame "2005-212协议" {
              w1931 = "" ("编码输出")
            }
            frame "2017-212协议", Default {
              # "盐度"
              # "总铜"
              n614 = Index Array(array=w1976, index #1=2 ("索引"), index #2=3 ("索引"), index #3=5 ("索引")) -> (element #1=w1948:string, element #2=w1947:string, element #3=w1932:string)
              n615 = Index Array(array=w1960, index=1 ("索引")) -> (element=w1936:string)
              n616 = Index Array(array=w1961, index=1 ("索引")) -> (element=w1937:string)
              n617 = Index Array(array=w1959, index=1 ("索引")) -> (element=w1938:string)
              n618 = Index Array(array=w1977, index #1=2 ("索引"), index #2=3 ("索引"), index #3=5 ("索引")) -> (element #1=w1951:string, element #2=w1950:string, element #3=w1934:string)
              n619 = Index Array(array=w1958, index=1 ("索引")) -> (element=w1939:string)
              n620 = case shown="\"M\", \"hd\"" w1951 {
                tunnel: [w1984 ""] -> w1949
                tunnel: w1950 -> [w1984 _]
                frame "N", Default {
                }
                frame "M", "hd" {
                }
              }
              n621 = case shown="\"M\", \"hd\"" w1948 {
                tunnel: [w1982 ""] -> w1946
                tunnel: w1947 -> [w1982 _]
                frame "N", Default {
                }
                frame "M", "hd" {
                }
              }
              n622 = call "数据编码整合输出.vi"("数据标识"="N" ("字符串"), "数据类型"="-Avg=", "污染物编码"="e01204", "数据值"=w1939) -> ("编码输出"=w1954:string)  [unwired: 7 in]
              n623 = call "数据编码整合输出.vi"("数据标识"="N" ("字符串"), "数据类型"="-Avg=", "污染物编码"="e01203", "数据值"=w1938) -> ("编码输出"=w1955:string)  [unwired: 7 in]
              n624 = call "数据编码整合输出.vi"("数据标识"=w1934, "数据类型"="-Avg=", "污染物编码"="w20122", "数据值"=w1949) -> ("编码输出"=w1975:string)  [unwired: 7 in]
              n625 = call "数据编码整合输出.vi"("数据标识"="N" ("字符串"), "数据类型"="-Avg=", "污染物编码"="e01201", "数据值"=w1937) -> ("编码输出"=w1957:string)  [unwired: 7 in]
              n626 = call "数据编码整合输出.vi"("数据标识"="N" ("字符串"), "数据类型"="-Avg=", "污染物编码"="e01202", "数据值"=w1936) -> ("编码输出"=w1956:string)  [unwired: 7 in]
              n627 = call "数据编码整合输出.vi"("数据标识"=w1932, "数据类型"="-Avg=", "污染物编码"="w01015", "数据值"=w1946) -> ("编码输出"=w1974:string)  [unwired: 7 in]
            }
          }
          n628 = case shown="\"2017-212协议\", 默认" w1728 {
            tunnel: w1824 -> [_ w1913]
            tunnel: w1812 -> [_ w1912]
            tunnel: w1808 -> [_ w1911]
            tunnel: w1807 -> [_ w1910]
            tunnel: w1806 -> [_ w1909]
            tunnel: [w1859 w1906] -> w1799
            tunnel: [w1859 w1903] -> w1798
            tunnel: [w1859 w1900] -> w1797
            tunnel: [w1859 w1897] -> w1796
            tunnel: [w1859 w1894] -> w1795
            frame "2005-212协议" {
              w1859 = "" ("编码输出")
            }
            frame "2017-212协议", Default {
              # "藻密度"
              # "叶绿素"
              # "浊度"
              # "电导率"
              # "DO"
              n629 = Index Array(array=w1910, index #1=2 ("索引"), index #2=3 ("索引"), index #3=5 ("索引")) -> (element #1=w1875:string, element #2=w1877:string, element #3=w1862:string)
              n630 = Index Array(array=w1912, index #1=2 ("索引"), index #2=3 ("索引"), index #3=5 ("索引")) -> (element #1=w1882:string, element #2=w1883:string, element #3=w1866:string)
              n631 = Index Array(array=w1911, index #1=2 ("索引"), index #2=3 ("索引"), index #3=5 ("索引")) -> (element #1=w1880:string, element #2=w1879:string, element #3=w1864:string)
              n632 = Index Array(array=w1909, index #1=2 ("索引"), index #2=3 ("索引"), index #3=5 ("索引")) -> (element #1=w1874:string, element #2=w1873:string, element #3=w1860:string)
              n633 = Index Array(array=w1913, index #1=2 ("索引"), index #2=3 ("索引"), index #3=5 ("索引")) -> (element #1=w1886:string, element #2=w1885:string, element #3=w1868:string)
              n634 = case shown="\"M\", \"hd\"" w1886 {
                tunnel: [w1923 ""] -> w1884
                tunnel: w1885 -> [w1923 _]
                frame "N", Default {
                }
                frame "M", "hd" {
                }
              }
              n635 = case shown="\"M\", \"hd\"" w1882 {
                tunnel: [w1921 ""] -> w1881
                tunnel: w1883 -> [w1921 _]
                frame "N", Default {
                }
                frame "M", "hd" {
                }
              }
              n636 = case shown="\"M\", \"hd\"" w1880 {
                tunnel: [w1919 ""] -> w1878
                tunnel: w1879 -> [w1919 _]
                frame "N", Default {
                }
                frame "M", "hd" {
                }
              }
              n637 = case shown="\"M\", \"hd\"" w1875 {
                tunnel: [w1917 ""] -> w1876
                tunnel: w1877 -> [w1917 _]
                frame "N", Default {
                }
                frame "M", "hd" {
                }
              }
              n638 = case shown="\"M\", \"hd\"" w1874 {
                tunnel: [w1915 ""] -> w1872
                tunnel: w1873 -> [w1915 _]
                frame "N", Default {
                }
                frame "M", "hd" {
                }
              }
              n639 = call "数据编码整合输出.vi"("数据标识"=w1866, "数据类型"="-Avg=", "污染物编码"="w01014", "数据值"=w1881) -> ("编码输出"=w1903:string)  [unwired: 7 in]
              n640 = call "数据编码整合输出.vi"("数据标识"=w1868, "数据类型"="-Avg=", "污染物编码"="w01009", "数据值"=w1884) -> ("编码输出"=w1906:string)  [unwired: 7 in]
              n641 = call "数据编码整合输出.vi"("数据标识"=w1860, "数据类型"="-Avg=", "污染物编码"="w19011", "数据值"=w1872) -> ("编码输出"=w1894:string)  [unwired: 7 in]
              n642 = call "数据编码整合输出.vi"("数据标识"=w1864, "数据类型"="-Avg=", "污染物编码"="w01003", "数据值"=w1878) -> ("编码输出"=w1900:string)  [unwired: 7 in]
              n643 = call "数据编码整合输出.vi"("数据标识"=w1862, "数据类型"="-Avg=", "污染物编码"="w01016", "数据值"=w1876) -> ("编码输出"=w1897:string)  [unwired: 7 in]
            }
          }
          n644 = case shown="\"2017-212协议\", 默认" w1730 {
            tunnel: w1810 -> [_ w1854]
            tunnel: ["" ("编码输出") w1853] -> w1805
            frame "2005-212协议" {
            }
            frame "2017-212协议", Default {
              # "CODMn"
              n645 = Index Array(array=w1854, index #1=2 ("索引"), index #2=3 ("索引"), index #3=5 ("索引")) -> (element #1=w1850:string, element #2=w1849:string, element #3=w1846:string)
              n646 = case shown="\"N\", 默认" w1850 {
                tunnel: [w1857 ""] -> w1848
                tunnel: w1849 -> [w1857 _]
                frame "N", Default {
                }
                frame "M", "hd" {
                }
              }
              n647 = call "数据编码整合输出.vi"("数据标识"=w1846, "数据类型"="-Avg=", "污染物编码"="w01019", "数据值"=w1848) -> ("编码输出"=w1853:string)  [unwired: 7 in]
            }
          }
          n648 = case shown="\"2017-212协议\", 默认" w1729 {
            tunnel: w1811 -> [_ w1842]
            tunnel: ["" ("编码输出") w1839] -> w1802
            frame "2005-212协议" {
            }
            frame "2017-212协议", Default {
              # "水温"
              n649 = Index Array(array=w1842, index #1=2 ("索引"), index #2=3 ("索引"), index #3=5 ("索引")) -> (element #1=w1836:string, element #2=w1837:string, element #3=w1832:string)
              n650 = case shown="\"M\", \"hd\"" w1836 {
                tunnel: [w1843 ""] -> w1835
                tunnel: w1837 -> [w1843 _]
                frame "N", Default {
                }
                frame "M", "hd" {
                }
              }
              n651 = call "数据编码整合输出.vi"("数据标识"=w1832, "数据类型"="-Avg=", "污染物编码"="w01010", "数据值"=w1835) -> ("编码输出"=w1839:string)  [unwired: 7 in]
            }
          }
          n652 = Index Array(array=w1809, index #1=2 ("索引"), index #2=3 ("索引"), index #3=5 ("索引")) -> (element #1=w1754:string, element #2=w1753:string, element #3=w1736:string)
          n653 = Index Array(array=w1820, index #1=2 ("索引"), index #2=3 ("索引"), index #3=5 ("索引")) -> (element #1=w1764:string, element #2=w1766:string, element #3=w1744:string)
          n654 = Index Array(array=w1815, index #1=2 ("索引"), index #2=3 ("索引"), index #3=5 ("索引")) -> (element #1=w1762:string, element #2=w1763:string, element #3=w1742:string)
          n655 = Index Array(array=w1823, index #1=2 ("索引"), index #2=3 ("索引"), index #3=5 ("索引")) -> (element #1=w1760:string, element #2=w1759:string, element #3=w1740:string)
          n656 = global read "全局 水样时间.vi" "选择发送的参数"() -> (w1773:string)
          n657 = Index Array(array=w1822, index #1=2 ("索引"), index #2=3 ("索引"), index #3=5 ("索引")) -> (element #1=w1757:string, element #2=w1756:string, element #3=w1738:string)
          n658 = case shown="\"M\", \"hd\"" w1760 {
            tunnel: [w1990 ""] -> w1758
            tunnel: w1759 -> [w1990 _]
            frame "N", Default {
            }
            frame "M", "hd" {
            }
          }
          n659 = case shown="\"M\", \"hd\"" w1762 {
            tunnel: [w1992 ""] -> w1761
            tunnel: w1763 -> [w1992 _]
            frame "N", Default {
            }
            frame "M", "hd" {
            }
          }
          n660 = case shown="\"M\", \"hd\"" w1754 {
            tunnel: [w1986 ""] -> w1752
            tunnel: w1753 -> [w1986 _]
            frame "N", Default {
            }
            frame "M", "hd" {
            }
          }
          n661 = case shown="\"M\", \"hd\"" w1757 {
            tunnel: [w1988 ""] -> w1755
            tunnel: w1756 -> [w1988 _]
            frame "N", Default {
            }
            frame "M", "hd" {
            }
          }
          n662 = case shown="\"M\", \"hd\"" w1764 {
            tunnel: [w1994 ""] -> w1765
            tunnel: w1766 -> [w1994 _]
            frame "N", Default {
            }
            frame "M", "hd" {
            }
          }
          n663 = case shown="\"铜\"" w1773 {
            tunnel: [w1996 w1997 w1998 w1999 w2000 w2001 w2002 w2003 w2004 w2005 w2006 w2007 w2008 w2009 w2010 w2011 w2012 w2013] -> w1771
            frame "CODMn", Default {
              n664 = global read "全局 所有参数.vi" "CODMn"() -> (w1996:string[][])
            }
            frame "CODCr" {
              n665 = global read "全局 所有参数.vi" "CODCr"() -> (w1997:string[][])
            }
            frame "DO" {
              n666 = global read "全局 所有参数.vi" "DO"() -> (w1998:string[][])
            }
            frame "铜" {
              n667 = global read "全局 所有参数.vi" "铜"() -> (w1999:string[][])
            }
            frame "PH" {
              n668 = global read "全局 所有参数.vi" "PH"() -> (w2000:string[][])
            }
            frame "氨氮" {
              n669 = global read "全局 所有参数.vi" "氨氮"() -> (w2001:string[][])
            }
            frame "比电导率", "电导率" {
              n670 = global read "全局 所有参数.vi" "电导率"() -> (w2002:string[][])
            }
            frame "水温" {
              n671 = global read "全局 所有参数.vi" "水温"() -> (w2003:string[][])
            }
            frame "盐度" {
              n672 = global read "全局 所有参数.vi" "盐度"() -> (w2004:string[][])
            }
            frame "浊度" {
              n673 = global read "全局 所有参数.vi" "浊度"() -> (w2005:string[][])
            }
            frame "总氮" {
              n674 = global read "全局 所有参数.vi" "总氮"() -> (w2006:string[][])
            }
            frame "总磷" {
              n675 = global read "全局 所有参数.vi" "总磷"() -> (w2007:string[][])
            }
            frame "叶绿素a" {
              n676 = global read "全局 所有参数.vi" "叶绿素"() -> (w2008:string[][])
            }
            frame "藻密度" {
              n677 = global read "全局 所有参数.vi" "藻密度"() -> (w2009:string[][])
            }
            frame "水位" {
              n678 = global read "全局流量数据小时.vi" "水位"() -> (w2010:string[][])
            }
            frame "流速" {
              n679 = global read "全局流量数据小时.vi" "流速"() -> (w2011:string[][])
            }
            frame "瞬时流量" {
              n680 = global read "全局流量数据小时.vi" "瞬时流量"() -> (w2012:string[][])
            }
            frame "累积流量" {
              n681 = global read "全局流量数据小时.vi" "累积流量"() -> (w2013:string[][])
            }
          }
          n682 = global read "全局 小时数据发送次数.vi" "小时数据发送次数"() -> (w1772:i32)
          n683 = global read "断电保存全局.vi" "数据发送协议"() -> (w1726:enum16{"2005-212协议", "2017-212协议"})
          n684 = global read "断电保存全局.vi" "数据发送协议"() -> (w1724:enum16{"2005-212协议", "2017-212协议"})
          n685 = global read "断电保存全局.vi" "数据发送协议"() -> (w1725:enum16{"2005-212协议", "2017-212协议"})
          n686 = Index Array(array=w1771, index (row)=w1772) -> (element=w1770:string[])  [unwired: 1 in]
          n687 = Index Array(array=w1770, index=0 ("索引")) -> (element=w1768:string)
          n688 = case shown="\"2005-212协议\"" w1724 {
            tunnel: ["011" ("污染物编码") "w01018" ("污染物编码")] -> w1731
            frame "2005-212协议" {
            }
            frame "2017-212协议", Default {
            }
          }
          n689 = case shown="\"2005-212协议\"" w1726 {
            tunnel: ["101" ("污染物编码") "w21011" ("污染物编码")] -> w1735
            tunnel: ["065" ("污染物编码") "w21001" ("污染物编码")] -> w1734
            tunnel: ["001" ("污染物编码") "w01001" ("污染物编码")] -> w1733
            frame "2005-212协议" {
            }
            frame "2017-212协议", Default {
            }
          }
          n690 = case shown="\"2005-212协议\"" w1725 {
            tunnel: ["060" ("污染物编码") "w21003" ("污染物编码")] -> w1732
            frame "2005-212协议" {
            }
            frame "2017-212协议", Default {
            }
          }
          n691 = call "规范小时时间戳.vi"("字符串"=w1768) -> ("result string"=w1747:string)  [unwired: 10 in]
          n692 = call "数据编码整合输出.vi"("数据标识"=w1742, "数据类型"="-Avg=", "污染物编码"=w1731, "数据值"=w1761) -> ("编码输出"=w1800:string)  [unwired: 7 in]
          n693 = call "数据编码整合输出.vi"("数据标识"=w1744, "数据类型"="-Avg=", "污染物编码"=w1732, "数据值"=w1765) -> ("编码输出"=w1803:string)  [unwired: 7 in]
          n694 = call "数据编码整合输出.vi"("数据标识"=w1738, "数据类型"="-Avg=", "污染物编码"=w1734, "数据值"=w1755) -> ("编码输出"=w1791:string)  [unwired: 7 in]
          n695 = call "数据编码整合输出.vi"("数据标识"=w1736, "数据类型"="-Avg=", "污染物编码"=w1733, "数据值"=w1752) -> ("编码输出"=w1789:string)  [unwired: 7 in]
          n696 = call "数据编码整合输出.vi"("数据标识"=w1740, "数据类型"="-Avg=", "污染物编码"=w1735, "数据值"=w1758) -> ("编码输出"=w1793:string)  [unwired: 7 in]
          n697 = Format Into String(format string="DataTime=%s;", w1747) -> (resulting string=w1751:string)  [unwired: 2 in, 1 out]
          n698 = Format Into String(format string="%s%s%s%s%s%s%s%s%s%s%s%s%s%s%s%s%s%s" ("格式字符串"), w1805, w1803, w1802, w1800, w1799, w1798, w1797, w1796, w1795, w1793, w1791, w1789, w1786, w1785, w1778, w1777, w1776, w1775) -> (resulting string=w1749:string)  [unwired: 2 in, 1 out]
          n699 = Empty String/Path?(string/path=w1749) -> (empty?=w1784:bool)
          n700 = Concatenate Strings(w1751, w1749) -> (w1748:string)
          n701 = global read "全局 数据发送重叠.vi" "主动上报数据中"() -> (w1767:bool)
          n702 = case shown="假" w1784 {
            tunnel: [w2015 ""] -> w1783
            tunnel: w1748 -> [w2015 _]
            tunnel: w1767 -> [w2014 w2018]
            frame False {
              n703 = case shown="真" w2014 {
                frame False {
                  n704 = global read "全局 小时数据发送次数.vi" "小时数据发送次数"() -> (w2017:i32)
                  n705 = Increment(x=w2017) -> (x+1=w2016:i32)
                  n706 = global write "全局 小时数据发送次数.vi" "小时数据发送次数"(w2016) -> ()
                }
                frame True {
                }
              }
            }
            frame True {
              n707 = case shown="假" w2018 {
                frame False {
                  n708 = global read "全局 小时数据发送次数.vi" "小时数据发送次数"() -> (w2021:i32)
                  n709 = Increment(x=w2021) -> (x+1=w2020:i32)
                  n710 = global write "全局 小时数据发送次数.vi" "小时数据发送次数"(w2020) -> ()
                }
                frame True {
                }
              }
            }
          }
        }
        frame "返回执行结果" {
          (unwired) 0 ("当前包数")
          n711 = global write "全局1.vi" "枚举"(enum16{"返回请求应答", "上传数据", "返回执行结果"}."返回请求应答" ("枚举")) -> ()
        }
      }
    }
    frame "提取小时数据" {
      # "藻密度"
      # "叶绿素"
      # "浊度"
      # "水温"
      # "发送小时数据"
      n712 = global read "全局 小时数据发送次数.vi" "小时数据发送次数"() -> (w2039:i32)
      n713 = global read "全局 小时数据发送次数.vi" "小时数据发送次数"() -> (w2040:i32)
      n714 = global read "全局 小时数据发送次数.vi" "小时数据发送次数"() -> (w2027:i32)
      n715 = global read "全局 小时数据发送次数.vi" "小时数据发送次数"() -> (w2043:i32)
      n716 = global read "全局 小时数据发送次数.vi" "小时数据发送次数"() -> (w2029:i32)
      n717 = global read "全局 小时数据发送次数.vi" "小时数据发送次数"() -> (w2049:i32)
      n718 = global read "全局 小时数据发送次数.vi" "小时数据发送次数"() -> (w2035:i32)
      n719 = global read "全局 小时数据发送次数.vi" "小时数据发送次数"() -> (w2047:i32)
      n720 = global read "全局 小时数据发送次数.vi" "小时数据发送次数"() -> (w2032:i32)
      n721 = global read "全局 小时数据发送次数.vi" "小时数据发送次数"() -> (w2051:i32)
      n722 = global read "全局 小时数据发送次数.vi" "小时数据发送次数"() -> (w2037:i32)
      n723 = global read "全局 小时数据发送次数.vi" "小时数据发送次数"() -> (w2045:i32)
      n724 = global read "全局 小时数据发送次数.vi" "小时数据发送次数"() -> (w2033:i32)
      n725 = global read "全局 小时数据发送次数.vi" "小时数据发送次数"() -> (w2053:i32)
      n726 = Index Array(array=w2060, index (row)=w2040) -> (element=w2041:string[])  [unwired: 1 in]
      n727 = Index Array(array=w2024, index (row)=w2027) -> (element=w2026:string[])  [unwired: 1 in]
      n728 = Index Array(array=w2061, index (row)=w2043) -> (element=w2042:string[])  [unwired: 1 in]
      n729 = Index Array(array=w2025, index (row)=w2029) -> (element=w2028:string[])  [unwired: 1 in]
      n730 = Index Array(array=w2065, index (row)=w2051) -> (element=w2050:string[])  [unwired: 1 in]
      n731 = Index Array(array=w2064, index (row)=w2049) -> (element=w2048:string[])  [unwired: 1 in]
      n732 = Index Array(array=w2063, index (row)=w2047) -> (element=w2046:string[])  [unwired: 1 in]
      n733 = Index Array(array=w2066, index (row)=w2053) -> (element=w2052:string[])  [unwired: 1 in]
      n734 = Index Array(array=w2059, index (row)=w2039) -> (element=w2038:string[])  [unwired: 1 in]
      n735 = Index Array(array=w2057, index (row)=w2035) -> (element=w2034:string[])  [unwired: 1 in]
      n736 = Index Array(array=w2058, index (row)=w2037) -> (element=w2036:string[])  [unwired: 1 in]
      n737 = Index Array(array=w2062, index (row)=w2045) -> (element=w2044:string[])  [unwired: 1 in]
      n738 = Index Array(array=w2055, index (row)=w2032) -> (element=w2030:string[])  [unwired: 1 in]
      n739 = Index Array(array=w2056, index (row)=w2033) -> (element=w2031:string[])  [unwired: 1 in]
      n740 = global read "全局1.vi" "枚举"() -> (w2054:enum16{"返回请求应答", "上传数据", "返回执行结果"})
      n741 = case shown="\"上传数据\"" w2054 {
        tunnel: ["QnRtn=1" w2102 "ExeRtn=1"] -> w2067
        tunnel: w2052 -> [_ w2166 _]
        tunnel: w2048 -> [_ w2179 _]
        tunnel: w2046 -> [_ w2178 _]
        tunnel: w2044 -> [_ w2177 _]
        tunnel: w2050 -> [_ w2176 _]
        tunnel: w2042 -> [_ w2165 _]
        tunnel: w2041 -> [_ w2170 _]
        tunnel: w2038 -> [_ w2168 _]
        tunnel: w2036 -> [_ w2167 _]
        tunnel: w2034 -> [_ w2164 _]
        tunnel: w2031 -> [_ w2163 _]
        tunnel: w2030 -> [_ w2162 _]
        tunnel: w2028 -> [_ w2107 _]
        tunnel: w2026 -> [_ w2106 _]
        frame "返回请求应答", Default {
          n742 = global read "全局 数据数组大小.vi" "数据数组大小"() -> (w2068:i32)
          n743 = Equal To 0?(x=w2068) -> (x = 0?=w2069:bool)
          n744 = case shown="真" w2069 {
            frame False {
            }
            frame True {
              n745 = global read "全局 小时数据发送次数.vi" "小时数据发送次数"() -> (w2072:i32)
              n746 = Increment(x=w2072) -> (x+1=w2071:i32)
              n747 = global write "全局 小时数据发送次数.vi" "小时数据发送次数"(w2071) -> ()
            }
          }
        }
        frame "上传数据" {
          (unwired) 2 ("数据精度")
          (unwired) 3 ("数据精度")
          (unwired) 3 ("数据精度")
          (unwired) 3 ("数据精度")
          (unwired) 3 ("数据精度")
          # "盐度"
          # "总铜"
          # "PH"
          # "总氮"
          # "总磷"
          # "藻密度"
          # "叶绿素"
          # "浊度"
          # "电导率"
          # "DO"
          # "CODCr"
          # "水温"
          # "NH3"
          # "CODMn"
          n748 = Index Array(array=w2163, index #2=1 ("索引")) -> (element #2=w2088:string)  [unwired: 1 in, 1 out]
          n749 = Index Array(array=w2168, index #2=1 ("索引")) -> (element #2=w2090:string)  [unwired: 1 in, 1 out]
          n750 = Index Array(array=w2164, index #2=1 ("索引")) -> (element #2=w2089:string)  [unwired: 1 in, 1 out]
          n751 = Index Array(array=w2162, index #2=1 ("索引")) -> (element #2=w2087:string)  [unwired: 1 in, 1 out]
          n752 = Index Array(array=w2167, index #2=1 ("索引")) -> (element #2=w2093:string)  [unwired: 1 in, 1 out]
          n753 = Index Array(array=w2179, index #2=1 ("索引")) -> (element #2=w2091:string)  [unwired: 1 in, 1 out]
          n754 = Index Array(array=w2166, index #2=1 ("索引")) -> (element #1=w2076:string, element #2=w2095:string)  [unwired: 1 in]
          n755 = Index Array(array=w2165, index #2=1 ("索引")) -> (element #2=w2084:string)  [unwired: 1 in, 1 out]
          n756 = Index Array(array=w2106, index #2=1 ("索引")) -> (element #2=w2082:string)  [unwired: 1 in, 1 out]
          n757 = Index Array(array=w2107, index #2=1 ("索引")) -> (element #2=w2083:string)  [unwired: 1 in, 1 out]
          n758 = Index Array(array=w2176, index #2=1 ("索引")) -> (element #2=w2094:string)  [unwired: 1 in, 1 out]
          n759 = Index Array(array=w2170, index #2=1 ("索引")) -> (element #2=w2092:string)  [unwired: 1 in, 1 out]
          n760 = Index Array(array=w2178, index #2=1 ("索引")) -> (element #2=w2086:string)  [unwired: 1 in, 1 out]
          n761 = Index Array(array=w2177, index #2=1 ("索引")) -> (element #2=w2085:string)  [unwired: 1 in, 1 out]
          n762 = call "规范小时时间戳.vi"("字符串"=w2076) -> ("result string"=w2077:string)  [unwired: 10 in]
          n763 = call "数据编码整合输出.vi"("数据标识"="N" ("字符串"), "数据类型"="-Avg=", "污染物编码"="w01019", "数据值"=w2095) -> ("编码输出"=w2161:string)  [unwired: 7 in]
          n764 = call "数据编码整合输出.vi"("数据标识"="N" ("字符串"), "数据类型"="-Avg=", "污染物编码"="w01010", "数据值"=w2093) -> ("编码输出"=w2150:string)  [unwired: 7 in]
          n765 = call "数据编码整合输出.vi"("数据标识"="N" ("字符串"), "数据类型"="-Avg=", "污染物编码"="w01018", "数据值"=w2092) -> ("编码输出"=w2146:string)  [unwired: 7 in]
          n766 = call "数据编码整合输出.vi"("数据标识"="N" ("字符串"), "数据类型"="-Avg=", "污染物编码"="w21003", "数据值"=w2094) -> ("编码输出"=w2154:string)  [unwired: 7 in]
          n767 = call "数据编码整合输出.vi"("数据标识"="N" ("字符串"), "数据类型"="-Avg=", "污染物编码"="w20122", "数据值"=w2083) -> ("编码输出"=w2105:string)  [unwired: 7 in]
          n768 = call "数据编码整合输出.vi"("数据标识"="N" ("字符串"), "数据类型"="-Avg=", "污染物编码"="w21001", "数据值"=w2085) -> ("编码输出"=w2118:string)  [unwired: 7 in]
          n769 = call "数据编码整合输出.vi"("数据标识"="N" ("字符串"), "数据类型"="-Avg=", "污染物编码"="w01001", "数据值"=w2084) -> ("编码输出"=w2114:string)  [unwired: 7 in]
          n770 = call "数据编码整合输出.vi"("数据标识"="N" ("字符串"), "数据类型"="-Avg=", "污染物编码"="w01015", "数据值"=w2082) -> ("编码输出"=w2104:string)  [unwired: 7 in]
          n771 = call "数据编码整合输出.vi"("数据标识"="N" ("字符串"), "数据类型"="-Avg=", "污染物编码"="w01014", "数据值"=w2090) -> ("编码输出"=w2138:string)  [unwired: 7 in]
          n772 = call "数据编码整合输出.vi"("数据标识"="N" ("字符串"), "数据类型"="-Avg=", "污染物编码"="w01009", "数据值"=w2091) -> ("编码输出"=w2142:string)  [unwired: 7 in]
          n773 = call "数据编码整合输出.vi"("数据标识"="N" ("字符串"), "数据类型"="-Avg=", "污染物编码"="w19011", "数据值"=w2087) -> ("编码输出"=w2126:string)  [unwired: 7 in]
          n774 = call "数据编码整合输出.vi"("数据标识"="N" ("字符串"), "数据类型"="-Avg=", "污染物编码"="w01003", "数据值"=w2089) -> ("编码输出"=w2134:string)  [unwired: 7 in]
          n775 = call "数据编码整合输出.vi"("数据标识"="N" ("字符串"), "数据类型"="-Avg=", "污染物编码"="w01016", "数据值"=w2088) -> ("编码输出"=w2130:string)  [unwired: 7 in]
          n776 = call "数据编码整合输出.vi"("数据标识"="N" ("字符串"), "数据类型"="-Avg=", "污染物编码"="w21011", "数据值"=w2086) -> ("编码输出"=w2122:string)  [unwired: 7 in]
          n777 = Format Into String(format string="DataTime=%s;", w2077) -> (resulting string=w2081:string)  [unwired: 2 in, 1 out]
          n778 = Format Into String(format string="%s%s%s%s%s%s%s%s%s%s%s%s%s%s" ("格式字符串"), w2161, w2154, w2150, w2146, w2142, w2138, w2134, w2130, w2126, w2122, w2118, w2114, w2105, w2104) -> (resulting string=w2079:string)  [unwired: 2 in, 1 out]
          n779 = Empty String/Path?(string/path=w2079) -> (empty?=w2103:bool)
          n780 = Concatenate Strings(w2081, w2079) -> (w2078:string)
          n781 = case shown="假" w2103 {
            tunnel: [w2182 ""] -> w2102
            tunnel: w2078 -> [w2182 _]
            frame False {
              n782 = global read "全局 小时数据发送次数.vi" "小时数据发送次数"() -> (w2181:i32)
              n783 = Increment(x=w2181) -> (x+1=w2180:i32)
              n784 = global write "全局 小时数据发送次数.vi" "小时数据发送次数"(w2180) -> ()
            }
            frame True {
              n785 = global read "全局 小时数据发送次数.vi" "小时数据发送次数"() -> (w2184:i32)
              n786 = Increment(x=w2184) -> (x+1=w2183:i32)
              n787 = global write "全局 小时数据发送次数.vi" "小时数据发送次数"(w2183) -> ()
            }
          }
        }
        frame "返回执行结果" {
        }
      }
    }
    frame "提取实时数据" {
      # "叶绿素"
      # "浊度"
      # "电导率"
      # "提取实时数据"
      n788 = global read "全局 小时数据发送次数.vi" "小时数据发送次数"() -> (w2191:i32)
      n789 = global read "全局 小时数据发送次数.vi" "小时数据发送次数"() -> (w2192:i32)
      n790 = global read "全局 小时数据发送次数.vi" "小时数据发送次数"() -> (w2206:i32)
      n791 = global read "全局 小时数据发送次数.vi" "小时数据发送次数"() -> (w2202:i32)
      n792 = global read "全局 小时数据发送次数.vi" "小时数据发送次数"() -> (w2196:i32)
      n793 = global read "全局 小时数据发送次数.vi" "小时数据发送次数"() -> (w2214:i32)
      n794 = global read "全局 小时数据发送次数.vi" "小时数据发送次数"() -> (w2216:i32)
      n795 = global read "全局 小时数据发送次数.vi" "小时数据发送次数"() -> (w2210:i32)
      n796 = global read "全局 小时数据发送次数.vi" "小时数据发送次数"() -> (w2198:i32)
      n797 = global read "全局 小时数据发送次数.vi" "小时数据发送次数"() -> (w2212:i32)
      n798 = global read "全局 小时数据发送次数.vi" "小时数据发送次数"() -> (w2195:i32)
      n799 = global read "全局 小时数据发送次数.vi" "小时数据发送次数"() -> (w2200:i32)
      n800 = global read "全局 小时数据发送次数.vi" "小时数据发送次数"() -> (w2208:i32)
      n801 = global read "全局 小时数据发送次数.vi" "小时数据发送次数"() -> (w2203:i32)
      n802 = Index Array(array=w2189, index (row)=w2191) -> (element=w2187:string[])  [unwired: 1 in]
      n803 = Index Array(array=w2190, index (row)=w2192) -> (element=w2188:string[])  [unwired: 1 in]
      n804 = Index Array(array=w2225, index (row)=w2206) -> (element=w2205:string[])  [unwired: 1 in]
      n805 = Index Array(array=w2230, index (row)=w2216) -> (element=w2215:string[])  [unwired: 1 in]
      n806 = Index Array(array=w2229, index (row)=w2214) -> (element=w2213:string[])  [unwired: 1 in]
      n807 = Index Array(array=w2222, index (row)=w2200) -> (element=w2199:string[])  [unwired: 1 in]
      n808 = Index Array(array=w2224, index (row)=w2203) -> (element=w2204:string[])  [unwired: 1 in]
      n809 = Index Array(array=w2228, index (row)=w2212) -> (element=w2211:string[])  [unwired: 1 in]
      n810 = Index Array(array=w2223, index (row)=w2202) -> (element=w2201:string[])  [unwired: 1 in]
      n811 = Index Array(array=w2227, index (row)=w2210) -> (element=w2209:string[])  [unwired: 1 in]
      n812 = Index Array(array=w2221, index (row)=w2198) -> (element=w2197:string[])  [unwired: 1 in]
      n813 = Index Array(array=w2220, index (row)=w2196) -> (element=w2194:string[])  [unwired: 1 in]
      n814 = Index Array(array=w2226, index (row)=w2208) -> (element=w2207:string[])  [unwired: 1 in]
      n815 = Index Array(array=w2219, index (row)=w2195) -> (element=w2193:string[])  [unwired: 1 in]
      n816 = global read "全局1.vi" "枚举"() -> (w2217:enum16{"返回请求应答", "上传数据", "返回执行结果"})
      n817 = case shown="\"上传数据\"" w2217 {
        tunnel: ["QnRtn=1" w2237 "ExeRtn=1"] -> w2218
        tunnel: w2215 -> [_ w2339 _]
        tunnel: w2211 -> [_ w2354 _]
        tunnel: w2209 -> [_ w2353 _]
        tunnel: w2207 -> [_ w2352 _]
        tunnel: w2213 -> [_ w2350 _]
        tunnel: w2205 -> [_ w2338 _]
        tunnel: w2204 -> [_ w2344 _]
        tunnel: w2201 -> [_ w2341 _]
        tunnel: w2199 -> [_ w2340 _]
        tunnel: w2197 -> [_ w2337 _]
        tunnel: w2194 -> [_ w2336 _]
        tunnel: w2193 -> [_ w2335 _]
        tunnel: w2188 -> [_ w2251 _]
        tunnel: w2187 -> [_ w2250 _]
        frame "返回请求应答", Default {
          n818 = global read "全局 数据数组大小.vi" "数据数组大小"() -> (w2231:i32)
          n819 = Equal To 0?(x=w2231) -> (x = 0?=w2232:bool)
          n820 = case shown="假" w2232 {
            frame False {
            }
            frame True {
              n821 = global read "全局 小时数据发送次数.vi" "小时数据发送次数"() -> (w2235:i32)
              n822 = Increment(x=w2235) -> (x+1=w2234:i32)
              n823 = global write "全局 小时数据发送次数.vi" "小时数据发送次数"(w2234) -> ()
            }
          }
        }
        frame "上传数据" {
          (unwired) 2 ("数据精度")
          (unwired) 3 ("数据精度")
          (unwired) 3 ("数据精度")
          (unwired) "-Rtd=" ("数据类型")
          (unwired) 3 ("数据精度")
          (unwired) 3 ("精度")
          # "盐度"
          # "总铜"
          # "PH"
          # "总氮"
          # "总磷"
          # "藻密度"
          # "叶绿素"
          # "浊度"
          # "电导率"
          # "DO"
          # "CODCr"
          # "水温"
          # "NH3"
          # "CODMn"
          n824 = Index Array(array=w2250, index #2=3 ("索引"), index #3=5 ("索引")) -> (element #2=w2243:string, element #3=w2242:string)  [unwired: 1 in, 1 out]
          n825 = Index Array(array=w2251, index #2=3 ("索引"), index #3=5 ("索引")) -> (element #2=w2245:string, element #3=w2244:string)  [unwired: 1 in, 1 out]
          n826 = Index Array(array=w2338, index #2=3 ("索引"), index #3=5 ("索引")) -> (element #2=w2258:string, element #3=w2259:string)  [unwired: 1 in, 1 out]
          n827 = Index Array(array=w2352, index #1=0 ("索引"), index #2=3 ("索引"), index #3=5 ("索引")) -> (element #2=w2261:string, element #3=w2262:string)  [unwired: 1 out]
          n828 = Index Array(array=w2336, index #2=3 ("索引"), index #3=5 ("索引")) -> (element #2=w2270:string, element #3=w2271:string)  [unwired: 1 in, 1 out]
          n829 = Index Array(array=w2335, index #2=3 ("索引"), index #3=5 ("索引")) -> (element #2=w2267:string, element #3=w2268:string)  [unwired: 1 in, 1 out]
          n830 = Index Array(array=w2340, index #2=3 ("索引"), index #3=5 ("索引")) -> (element #2=w2303:string, element #3=w2304:string)  [unwired: 1 in, 1 out]
          n831 = Index Array(array=w2341, index #2=3 ("索引"), index #3=5 ("索引")) -> (element #2=w2288:string, element #3=w2289:string)  [unwired: 1 in, 1 out]
          n832 = Index Array(array=w2337, index #2=3 ("索引"), index #3=5 ("索引")) -> (element #2=w2274:string, element #3=w2275:string)  [unwired: 1 in, 1 out]
          n833 = Index Array(array=w2353, index #1=0 ("索引"), index #2=3 ("索引"), index #3=5 ("索引")) -> (element #2=w2264:string, element #3=w2265:string)  [unwired: 1 out]
          n834 = Index Array(array=w2339, index #1=0 ("索引"), index #2=3 ("索引"), index #3=5 ("索引")) -> (element #1=w2257:string, element #2=w2313:string, element #3=w2312:string)
          n835 = Index Array(array=w2350, index #1=0 ("索引"), index #2=3 ("索引"), index #3=5 ("索引")) -> (element #2=w2306:string, element #3=w2307:string)  [unwired: 1 out]
          n836 = Index Array(array=w2344, index #1=0 ("索引"), index #2=3 ("索引"), index #3=5 ("索引")) -> (element #2=w2294:string, element #3=w2295:string)  [unwired: 1 out]
          n837 = Index Array(array=w2354, index #1=0 ("索引"), index #2=3 ("索引"), index #3=5 ("索引")) -> (element #2=w2291:string, element #3=w2292:string)  [unwired: 1 out]
          n838 = call "规范时间戳.vi"("字符串"=w2257) -> ("result string"=w2256:string)  [unwired: 10 in]
          n839 = call "数据编码整合输出.vi"("数据标识"=w2243, "数据类型"="-Rtd=", "污染物编码"="w01015", "数据值"=w2242) -> ("编码输出"=w2240:string)  [unwired: 7 in]
          n840 = call "数据编码整合输出.vi"("数据标识"=w2245, "数据类型"="-Rtd=", "污染物编码"="w20122", "数据值"=w2244) -> ("编码输出"=w2241:string)  [unwired: 7 in]
          n841 = call "数据编码整合输出.vi"("数据标识"=w2259, "数据类型"="-Rtd=", "污染物编码"="w01001", "数据值"=w2258) -> ("编码输出"=w2260:string)  [unwired: 7 in]
          n842 = call "数据编码整合输出.vi"("数据标识"=w2312, "数据类型"="-Rtd=", "污染物编码"="w01019", "数据值"=w2313) -> ("编码输出"=w2311:string)  [unwired: 7 in]
          n843 = call "数据编码整合输出.vi"("数据标识"=w2307, "数据类型"="-Rtd=", "污染物编码"="w21003", "数据值"=w2306) -> ("编码输出"=w2305:string)  [unwired: 7 in]
          n844 = call "数据编码整合输出.vi"("数据标识"=w2262, "数据类型"="-Rtd=", "污染物编码"="w21001", "数据值"=w2261) -> ("编码输出"=w2263:string)  [unwired: 7 in]
          n845 = call "数据编码整合输出.vi"("数据标识"=w2271, "数据类型"="-Rtd=", "污染物编码"="w01016", "数据值"=w2270) -> ("编码输出"=w2272:string)  [unwired: 7 in]
          n846 = call "数据编码整合输出.vi"("数据标识"=w2268, "数据类型"="-Rtd=", "污染物编码"="w19011", "数据值"=w2267) -> ("编码输出"=w2269:string)  [unwired: 7 in]
          n847 = call "数据编码整合输出.vi"("数据标识"=w2265, "污染物编码"="w21011", "数据值"=w2264) -> ("编码输出"=w2266:string)  [unwired: 8 in]
          n848 = call "数据编码整合输出.vi"("数据标识"=w2295, "数据类型"="-Rtd=", "污染物编码"="w01018", "数据值"=w2294) -> ("编码输出"=w2293:string)  [unwired: 7 in]
          n849 = call "数据编码整合输出.vi"("数据标识"=w2304, "数据类型"="-Rtd=", "污染物编码"="w01010", "数据值"=w2303) -> ("编码输出"=w2302:string)  [unwired: 7 in]
          n850 = call "数据编码整合输出.vi"("数据标识"=w2275, "数据类型"="-Rtd=", "污染物编码"="w01003", "数据值"=w2274) -> ("编码输出"=w2273:string)  [unwired: 7 in]
          n851 = call "数据编码整合输出.vi"("数据标识"=w2289, "数据类型"="-Rtd=", "污染物编码"="w01014", "数据值"=w2288) -> ("编码输出"=w2287:string)  [unwired: 7 in]
          n852 = call "数据编码整合输出.vi"("数据标识"=w2292, "数据类型"="-Rtd=", "污染物编码"="w01009", "数据值"=w2291) -> ("编码输出"=w2290:string)  [unwired: 7 in]
          n853 = Empty String/Path?(string/path=w2256) -> (empty?=w2239:bool)
          n854 = Format Into String(format string="DataTime=%s;%s%s%s%s%s%s%s%s%s%s%s%s%s%s" ("格式字符串"), w2256, w2311, w2305, w2302, w2293, w2290, w2287, w2273, w2272, w2269, w2266, w2263, w2260, w2241, w2240) -> (resulting string=w2238:string)  [unwired: 2 in, 1 out]
          n855 = case shown="真" w2239 {
            tunnel: [w2359 ""] -> w2237
            tunnel: w2238 -> [w2359 _]
            frame False {
              n856 = global read "全局 小时数据发送次数.vi" "小时数据发送次数"() -> (w2361:i32)
              n857 = Increment(x=w2361) -> (x+1=w2360:i32)
              n858 = global write "全局 小时数据发送次数.vi" "小时数据发送次数"(w2360) -> ()
            }
            frame True {
              n859 = global read "全局 小时数据发送次数.vi" "小时数据发送次数"() -> (w2363:i32)
              n860 = Increment(x=w2363) -> (x+1=w2362:i32)
              n861 = global write "全局 小时数据发送次数.vi" "小时数据发送次数"(w2362) -> ()
            }
          }
        }
        frame "返回执行结果" {
        }
      }
    }
    frame "核查数据" {
      # "提取标样核查数据"
      n862 = global read "全局 小时数据发送次数.vi" "小时数据发送次数"() -> (w2368:i32)
      n863 = global read "全局 小时数据发送次数.vi" "小时数据发送次数"() -> (w2385:i32)
      n864 = global read "全局 小时数据发送次数.vi" "小时数据发送次数"() -> (w2387:i32)
      n865 = global read "全局 小时数据发送次数.vi" "小时数据发送次数"() -> (w2383:i32)
      n866 = global read "全局 小时数据发送次数.vi" "小时数据发送次数"() -> (w2379:i32)
      n867 = global read "全局 小时数据发送次数.vi" "小时数据发送次数"() -> (w2371:i32)
      n868 = global read "全局 小时数据发送次数.vi" "小时数据发送次数"() -> (w2377:i32)
      n869 = global read "全局 小时数据发送次数.vi" "小时数据发送次数"() -> (w2374:i32)
      n870 = global read "全局 小时数据发送次数.vi" "小时数据发送次数"() -> (w2381:i32)
      n871 = Index Array(array=w2366, index (row)=w2368) -> (element=w2367:string[])  [unwired: 1 in]
      n872 = Index Array(array=w2393, index (row)=w2385) -> (element=w2384:string[])  [unwired: 1 in]
      n873 = Index Array(array=w2394, index (row)=w2387) -> (element=w2386:string[])  [unwired: 1 in]
      n874 = Index Array(array=w2392, index (row)=w2383) -> (element=w2382:string[])  [unwired: 1 in]
      n875 = Index Array(array=w2389, index (row)=w2379) -> (element=w2378:string[])  [unwired: 1 in]
      n876 = Index Array(array=w2369, index (row)=w2371) -> (element=w2370:string[])  [unwired: 1 in]
      n877 = Index Array(array=w2376, index (row)=w2377) -> (element=w2375:string[])  [unwired: 1 in]
      n878 = Index Array(array=w2372, index (row)=w2374) -> (element=w2373:string[])  [unwired: 1 in]
      n879 = Index Array(array=w2391, index (row)=w2381) -> (element=w2380:string[])  [unwired: 1 in]
      n880 = global read "全局1.vi" "枚举"() -> (w2388:enum16{"返回请求应答", "上传数据", "返回执行结果"})
      n881 = case shown="\"上传数据\"" w2388 {
        tunnel: ["QnRtn=1" w2445 "ExeRtn=1"] -> w2390
        tunnel: w2386 -> [_ w2465 _]
        tunnel: w2382 -> [_ w2464 _]
        tunnel: w2380 -> [_ w2463 _]
        tunnel: w2384 -> [_ w2461 _]
        tunnel: w2378 -> [_ w2449 _]
        tunnel: w2375 -> [_ w2424 _]
        tunnel: w2373 -> [_ w2416 _]
        tunnel: w2370 -> [_ w2412 _]
        tunnel: w2367 -> [_ w2404 _]
        frame "返回请求应答", Default {
          n882 = global read "全局 数据数组大小.vi" "数据数组大小"() -> (w2396:i32)
          n883 = Equal To 0?(x=w2396) -> (x = 0?=w2395:bool)
          n884 = case shown="真" w2395 {
            frame False {
            }
            frame True {
              n885 = global read "全局 小时数据发送次数.vi" "小时数据发送次数"() -> (w2399:i32)
              n886 = Increment(x=w2399) -> (x+1=w2398:i32)
              n887 = global write "全局 小时数据发送次数.vi" "小时数据发送次数"(w2398) -> ()
            }
          }
        }
        frame "上传数据" {
          # "将非空数组的时间戳写入"
          n888 = Index Array(array=w2404, index #1=0 ("索引"), index #2=3 ("索引"), index #3=7 ("索引")) -> (element #2=w2405:string, element #3=w2406:string)  [unwired: 1 out]
          n889 = Index Array(array=w2412, index #1=0 ("索引"), index #2=3 ("索引"), index #3=7 ("索引")) -> (element #2=w2411:string, element #3=w2410:string)  [unwired: 1 out]
          n890 = Index Array(array=w2424, index #1=0 ("索引"), index #2=3 ("索引"), index #3=7 ("索引")) -> (element #2=w2423:string, element #3=w2422:string)  [unwired: 1 out]
          n891 = Index Array(array=w2416, index #1=0 ("索引"), index #2=3 ("索引"), index #3=7 ("索引")) -> (element #2=w2417:string, element #3=w2418:string)  [unwired: 1 out]
          n892 = Index Array(array=w2463, index #1=0 ("索引"), index #2=3 ("索引"), index #3=7 ("索引")) -> (element #2=w2433:string, element #3=w2432:string)  [unwired: 1 out]
          n893 = Index Array(array=w2461, index #1=0 ("索引"), index #2=3 ("索引"), index #3=7 ("索引")) -> (element #1=w2444:string, element #2=w2439:string, element #3=w2438:string)
          n894 = Index Array(array=w2465, index #1=0 ("索引"), index #2=3 ("索引"), index #3=7 ("索引")) -> (element #2=w2442:string, element #3=w2441:string)  [unwired: 1 out]
          n895 = Index Array(array=w2464, index #1=0 ("索引"), index #2=3 ("索引"), index #3=7 ("索引")) -> (element #2=w2435:string, element #3=w2434:string)  [unwired: 1 out]
          n896 = Index Array(array=w2449, index #1=0 ("索引"), index #2=3 ("索引"), index #3=7 ("索引")) -> (element #2=w2428:string, element #3=w2430:string)  [unwired: 1 out]
          n897 = case shown="\"真\", 默认" w2405 {
            tunnel: [w2469 w2479] -> w2400
            tunnel: w2405 -> [w2469 w2473]
            tunnel: w2406 -> [_ w2472]
            frame "" {
            }
            frame "真", Default {
              n898 = call "核查数据编码整合输出.vi"("字段结束"=FALSE, "数据标识"="N" ("字符串"), "数据类型"="-Check=", "污染物编码"="w01003", "数据值"=w2473) -> ("编码输出"=w2480:string)  [unwired: 6 in]
              n899 = call "核查数据编码整合输出.vi"("字段结束"=TRUE, "数据标识"="N" ("字符串"), "数据类型"="-StandardValue=", "污染物编码"="w01003", "数据值"=w2472) -> ("编码输出"=w2476:string)  [unwired: 6 in]
              n900 = Concatenate Strings(w2480, w2476) -> (w2479:string)
            }
          }
          n901 = case shown="\"真\", 默认" w2417 {
            tunnel: w2417 -> [w2497 w2509]
            tunnel: [w2497 w2506] -> w2402
            tunnel: w2418 -> [_ w2502]
            frame "" {
            }
            frame "真", Default {
              n902 = call "核查数据编码整合输出.vi"("字段结束"=FALSE, "数据标识"="N" ("字符串"), "数据类型"="-Check=", "污染物编码"="w01009", "数据值"=w2509) -> ("编码输出"=w2507:string)  [unwired: 6 in]
              n903 = call "核查数据编码整合输出.vi"("字段结束"=TRUE, "数据标识"="N" ("字符串"), "数据类型"="-StandardValue=", "污染物编码"="w01009", "数据值"=w2502) -> ("编码输出"=w2503:string)  [unwired: 6 in]
              n904 = Concatenate Strings(w2507, w2503) -> (w2506:string)
            }
          }
          n905 = case shown="\"真\", 默认" w2411 {
            tunnel: [w2483 w2493] -> w2401
            tunnel: w2411 -> [w2483 w2485]
            tunnel: w2410 -> [_ w2484]
            frame "" {
            }
            frame "真", Default {
              n906 = call "核查数据编码整合输出.vi"("字段结束"=FALSE, "数据标识"="N" ("字符串"), "数据类型"="-Check=", "污染物编码"="w01014", "数据值"=w2485) -> ("编码输出"=w2494:string)  [unwired: 6 in]
              n907 = call "核查数据编码整合输出.vi"("字段结束"=TRUE, "数据标识"="N" ("字符串"), "数据类型"="-StandardValue=", "污染物编码"="w01014", "数据值"=w2484) -> ("编码输出"=w2490:string)  [unwired: 6 in]
              n908 = Concatenate Strings(w2494, w2490) -> (w2493:string)
            }
          }
          n909 = case shown="\"真\", 默认" w2423 {
            tunnel: w2423 -> [w2511 w2523]
            tunnel: [w2511 w2520] -> w2403
            tunnel: w2422 -> [_ w2516]
            frame "" {
            }
            frame "真", Default {
              n910 = call "核查数据编码整合输出.vi"("字段结束"=FALSE, "数据标识"="N" ("字符串"), "数据类型"="-Check=", "污染物编码"="w01001", "数据值"=w2523) -> ("编码输出"=w2521:string)  [unwired: 6 in]
              n911 = call "核查数据编码整合输出.vi"("字段结束"=TRUE, "数据标识"="N" ("字符串"), "数据类型"="-StandardValue=", "污染物编码"="w01001", "数据值"=w2516) -> ("编码输出"=w2517:string)  [unwired: 6 in]
              n912 = Concatenate Strings(w2521, w2517) -> (w2520:string)
            }
          }
          n913 = case shown="\"真\", 默认" w2442 {
            tunnel: w2442 -> [w2581 w2593]
            tunnel: [w2581 w2589] -> w2440
            tunnel: w2441 -> [_ w2584]
            frame "" {
            }
            frame "真", Default {
              # "CODMn"
              n914 = call "核查数据编码整合输出.vi"("字段结束"=FALSE, "数据标识"="N" ("字符串"), "数据类型"="-Check=", "污染物编码"="w01019", "数据值"=w2593) -> ("编码输出"=w2590:string)  [unwired: 6 in]
              n915 = call "核查数据编码整合输出.vi"("字段结束"=TRUE, "数据标识"="N" ("字符串"), "数据类型"="-StandardValue=", "污染物编码"="w01019", "数据值"=w2584) -> ("编码输出"=w2585:string)  [unwired: 6 in]
              n916 = Concatenate Strings(w2590, w2585) -> (w2589:string)
            }
          }
          n917 = case shown="\"真\", 默认" w2428 {
            tunnel: w2428 -> [w2525 w2537]
            tunnel: [w2525 w2534] -> w2429
            tunnel: w2430 -> [_ w2530]
            frame "" {
            }
            frame "真", Default {
              n918 = call "核查数据编码整合输出.vi"("字段结束"=FALSE, "数据标识"="N" ("字符串"), "数据类型"="-Check=", "污染物编码"="w01018", "数据值"=w2537) -> ("编码输出"=w2535:string)  [unwired: 6 in]
              n919 = call "核查数据编码整合输出.vi"("字段结束"=TRUE, "数据标识"="N" ("字符串"), "数据类型"="-StandardValue=", "污染物编码"="w01018", "数据值"=w2530) -> ("编码输出"=w2531:string)  [unwired: 6 in]
              n920 = Concatenate Strings(w2535, w2531) -> (w2534:string)
            }
          }
          n921 = case shown="\"真\", 默认" w2439 {
            tunnel: w2439 -> [w2567 w2579]
            tunnel: [w2567 w2576] -> w2437
            tunnel: w2438 -> [_ w2572]
            frame "" {
            }
            frame "真", Default {
              n922 = call "核查数据编码整合输出.vi"("字段结束"=FALSE, "数据标识"="N" ("字符串"), "数据类型"="-Check=", "污染物编码"="w21003", "数据值"=w2579) -> ("编码输出"=w2577:string)  [unwired: 6 in]
              n923 = call "核查数据编码整合输出.vi"("字段结束"=TRUE, "数据标识"="N" ("字符串"), "数据类型"="-StandardValue=", "污染物编码"="w21003", "数据值"=w2572) -> ("编码输出"=w2573:string)  [unwired: 6 in]
              n924 = Concatenate Strings(w2577, w2573) -> (w2576:string)
            }
          }
          n925 = case shown="\"真\", 默认" w2435 {
            tunnel: w2435 -> [w2553 w2565]
            tunnel: [w2553 w2562] -> w2436
            tunnel: w2434 -> [_ w2558]
            frame "" {
            }
            frame "真", Default {
              n926 = call "核查数据编码整合输出.vi"("字段结束"=FALSE, "数据标识"="N" ("字符串"), "数据类型"="-Check=", "污染物编码"="w21011", "数据值"=w2565) -> ("编码输出"=w2563:string)  [unwired: 6 in]
              n927 = call "核查数据编码整合输出.vi"("字段结束"=TRUE, "数据标识"="N" ("字符串"), "数据类型"="-StandardValue=", "污染物编码"="w21011", "数据值"=w2558) -> ("编码输出"=w2559:string)  [unwired: 6 in]
              n928 = Concatenate Strings(w2563, w2559) -> (w2562:string)
            }
          }
          n929 = case shown="\"真\", 默认" w2433 {
            tunnel: w2433 -> [w2539 w2551]
            tunnel: [w2539 w2548] -> w2431
            tunnel: w2432 -> [_ w2544]
            frame "" {
            }
            frame "真", Default {
              n930 = call "核查数据编码整合输出.vi"("字段结束"=FALSE, "数据标识"="N" ("字符串"), "数据类型"="-Check=", "污染物编码"="w21001", "数据值"=w2551) -> ("编码输出"=w2549:string)  [unwired: 6 in]
              n931 = call "核查数据编码整合输出.vi"("字段结束"=TRUE, "数据标识"="N" ("字符串"), "数据类型"="-StandardValue=", "污染物编码"="w21001", "数据值"=w2544) -> ("编码输出"=w2545:string)  [unwired: 6 in]
              n932 = Concatenate Strings(w2549, w2545) -> (w2548:string)
            }
          }
          n933 = call "规范时间戳.vi"("字符串"=w2444) -> ("result string"=w2443:string)  [unwired: 10 in]
          n934 = Format Into String(format string="DataTime=%s;%s%s%s%s%s%s%s%s%s" ("格式字符串"), w2443, w2440, w2437, w2436, w2431, w2429, w2403, w2402, w2401, w2400) -> (resulting string=w2446:string)  [unwired: 2 in, 1 out]
          n935 = Empty String/Path?(string/path=w2443) -> (empty?=w2447:bool)
          n936 = case shown="假" w2447 {
            tunnel: [w2597 ""] -> w2445
            tunnel: w2446 -> [w2597 _]
            frame False {
              n937 = global read "全局 小时数据发送次数.vi" "小时数据发送次数"() -> (w2596:i32)
              n938 = Increment(x=w2596) -> (x+1=w2595:i32)
              n939 = global write "全局 小时数据发送次数.vi" "小时数据发送次数"(w2595) -> ()
            }
            frame True {
              n940 = global read "全局 小时数据发送次数.vi" "小时数据发送次数"() -> (w2599:i32)
              n941 = Increment(x=w2599) -> (x+1=w2598:i32)
              n942 = global write "全局 小时数据发送次数.vi" "小时数据发送次数"(w2598) -> ()
            }
          }
        }
        frame "返回执行结果" {
        }
      }
    }
    frame "空白测试", "跨度核查", "零点核查" {
      # "提取空白测试数据/零点核查数据/跨度核查数据"
      n943 = global read "全局 小时数据发送次数.vi" "小时数据发送次数"() -> (w2609:i32)
      n944 = global read "全局 小时数据发送次数.vi" "小时数据发送次数"() -> (w2611:i32)
      n945 = global read "全局 小时数据发送次数.vi" "小时数据发送次数"() -> (w2607:i32)
      n946 = global read "全局 小时数据发送次数.vi" "小时数据发送次数"() -> (w2603:i32)
      n947 = global read "全局 小时数据发送次数.vi" "小时数据发送次数"() -> (w2605:i32)
      n948 = Index Array(array=w2617, index (row)=w2609) -> (element=w2608:string[])  [unwired: 1 in]
      n949 = Index Array(array=w2618, index (row)=w2611) -> (element=w2610:string[])  [unwired: 1 in]
      n950 = Index Array(array=w2616, index (row)=w2607) -> (element=w2606:string[])  [unwired: 1 in]
      n951 = Index Array(array=w2613, index (row)=w2603) -> (element=w2602:string[])  [unwired: 1 in]
      n952 = Index Array(array=w2615, index (row)=w2605) -> (element=w2604:string[])  [unwired: 1 in]
      n953 = global read "全局1.vi" "枚举"() -> (w2612:enum16{"返回请求应答", "上传数据", "返回执行结果"})
      n954 = case shown="\"上传数据\"" w2612 {
        tunnel: ["QnRtn=1" w2641 "ExeRtn=1"] -> w2614
        tunnel: w2610 -> [_ w2661 _]
        tunnel: w2606 -> [_ w2660 _]
        tunnel: w2604 -> [_ w2659 _]
        tunnel: w2608 -> [_ w2657 _]
        tunnel: w2602 -> [_ w2645 _]
        frame "返回请求应答", Default {
          (unwired) 0 ("当前包数")
          n955 = global read "全局 数据数组大小.vi" "数据数组大小"() -> (w2620:i32)
          n956 = Equal To 0?(x=w2620) -> (x = 0?=w2619:bool)
          n957 = case shown="真" w2619 {
            frame False {
            }
            frame True {
              n958 = global read "全局 小时数据发送次数.vi" "小时数据发送次数"() -> (w2623:i32)
              n959 = Increment(x=w2623) -> (x+1=w2622:i32)
              n960 = global write "全局 小时数据发送次数.vi" "小时数据发送次数"(w2622) -> ()
            }
          }
        }
        frame "上传数据" {
          # "将非空数组的时间戳写入"
          n961 = Index Array(array=w2659, index #1=0 ("索引"), index #2=3 ("索引"), index #3=7 ("索引")) -> (element #2=w2628:string, element #3=w2627:string)  [unwired: 1 out]
          n962 = Index Array(array=w2657, index #1=0 ("索引"), index #2=3 ("索引"), index #3=7 ("索引")) -> (element #1=w2640:string, element #2=w2635:string, element #3=w2634:string)
          n963 = Index Array(array=w2661, index #1=0 ("索引"), index #2=3 ("索引"), index #3=7 ("索引")) -> (element #2=w2637:string, element #3=w2636:string)  [unwired: 1 out]
          n964 = Index Array(array=w2660, index #1=0 ("索引"), index #2=3 ("索引"), index #3=7 ("索引")) -> (element #2=w2630:string, element #3=w2632:string)  [unwired: 1 out]
          n965 = Index Array(array=w2645, index #1=0 ("索引"), index #2=3 ("索引"), index #3=7 ("索引")) -> (element #2=w2625:string, element #3=w2626:string)  [unwired: 1 out]
          n966 = case shown="\"真\", 默认" w2628 {
            tunnel: [w2688 w2700] -> w2629
            tunnel: w2628 -> [w2688 w2690]
            tunnel: w2627 -> [_ w2689]
            frame "" {
            }
            frame "真", Default {
              # "总氮"
              n967 = call "核查数据编码整合输出.vi"("字段结束"=TRUE, "数据标识"="N" ("字符串"), "数据类型"="-SpanValue=", "污染物编码"="w21001", "数据精度"=3 ("精度"), "数据值"="0") -> ("编码输出"=w2692:string)  [unwired: 5 in]
              n968 = call "核查数据编码整合输出.vi"("字段结束"=FALSE, "数据标识"="N" ("字符串"), "数据类型"="-StandardValue=", "污染物编码"="w21001", "数据精度"=3 ("精度"), "数据值"=w2689) -> ("编码输出"=w2702:string)  [unwired: 5 in]
              n969 = call "核查数据编码整合输出.vi"("字段结束"=FALSE, "数据标识"="N" ("字符串"), "数据类型"="-Check=", "污染物编码"="w21001", "数据精度"=3 ("精度"), "数据值"=w2690) -> ("编码输出"=w2701:string)  [unwired: 5 in]
              n970 = Concatenate Strings(w2701, w2702, w2692) -> (w2700:string)
            }
          }
          n971 = case shown="\"真\", 默认" w2625 {
            tunnel: [w2665 w2677] -> w2624
            tunnel: w2625 -> [w2665 w2667]
            tunnel: w2626 -> [_ w2666]
            frame "" {
            }
            frame "真", Default {
              # "CODCr"
              n972 = call "核查数据编码整合输出.vi"("字段结束"=TRUE, "数据标识"="N" ("字符串"), "数据类型"="-SpanValue=", "污染物编码"="w01018", "数据精度"=3 ("精度"), "数据值"="0") -> ("编码输出"=w2669:string)  [unwired: 5 in]
              n973 = call "核查数据编码整合输出.vi"("字段结束"=FALSE, "数据标识"="N" ("字符串"), "数据类型"="-StandardValue=", "污染物编码"="w01018", "数据精度"=3 ("精度"), "数据值"=w2666) -> ("编码输出"=w2686:string)  [unwired: 5 in]
              n974 = call "核查数据编码整合输出.vi"("字段结束"=FALSE, "数据标识"="N" ("字符串"), "数据类型"="-Check=", "污染物编码"="w01018", "数据精度"=3 ("精度"), "数据值"=w2667) -> ("编码输出"=w2687:string)  [unwired: 5 in]
              n975 = Concatenate Strings(w2687, w2686, w2669) -> (w2677:string)
            }
          }
          n976 = case shown="\"真\", 默认" w2630 {
            tunnel: w2630 -> [w2711 w2723]
            tunnel: w2632 -> [_ w2722]
            tunnel: [w2711 w2721] -> w2631
            frame "" {
            }
            frame "真", Default {
              # "总磷"
              n977 = call "核查数据编码整合输出.vi"("字段结束"=TRUE, "数据标识"="N" ("字符串"), "数据类型"="-SpanValue=", "污染物编码"="w21011", "数据精度"=3 ("精度"), "数据值"="0") -> ("编码输出"=w2716:string)  [unwired: 5 in]
              n978 = call "核查数据编码整合输出.vi"("字段结束"=FALSE, "数据标识"="N" ("字符串"), "数据类型"="-StandardValue=", "污染物编码"="w21011", "数据精度"=3 ("精度"), "数据值"=w2722) -> ("编码输出"=w2732:string)  [unwired: 5 in]
              n979 = call "核查数据编码整合输出.vi"("字段结束"=FALSE, "数据标识"="N" ("字符串"), "数据类型"="-Check=", "污染物编码"="w21011", "数据精度"=3 ("精度"), "数据值"=w2723) -> ("编码输出"=w2733:string)  [unwired: 5 in]
              n980 = Concatenate Strings(w2733, w2732, w2716) -> (w2721:string)
            }
          }
          n981 = case shown="\"真\", 默认" w2635 {
            tunnel: w2635 -> [w2734 w2748]
            tunnel: w2634 -> [_ w2747]
            tunnel: [w2734 w2744] -> w2633
            frame "" {
            }
            frame "真", Default {
              # "NH3"
              n982 = call "核查数据编码整合输出.vi"("字段结束"=FALSE, "数据标识"="N" ("字符串"), "数据类型"="-Check=", "污染物编码"="w21003", "数据精度"=3 ("精度"), "数据值"=w2748) -> ("编码输出"=w2745:string)  [unwired: 5 in]
              n983 = call "核查数据编码整合输出.vi"("字段结束"=FALSE, "数据标识"="N" ("字符串"), "数据类型"="-StandardValue=", "污染物编码"="w21003", "数据精度"=3 ("精度"), "数据值"=w2747) -> ("编码输出"=w2746:string)  [unwired: 5 in]
              n984 = call "核查数据编码整合输出.vi"("字段结束"=TRUE, "数据标识"="N" ("字符串"), "数据类型"="-SpanValue=", "污染物编码"="w21003", "数据精度"=3 ("精度"), "数据值"="0") -> ("编码输出"=w2737:string)  [unwired: 5 in]
              n985 = Concatenate Strings(w2745, w2746, w2737) -> (w2744:string)
            }
          }
          n986 = case shown="\"真\", 默认" w2637 {
            tunnel: w2637 -> [w2757 w2775]
            tunnel: [w2757 w2771] -> w2638
            tunnel: w2636 -> [_ w2763]
            frame "" {
            }
            frame "真", Default {
              # "CODMn"
              n987 = call "核查数据编码整合输出.vi"("字段结束"=FALSE, "数据标识"="N" ("字符串"), "数据类型"="-Check=", "污染物编码"="w01019", "数据值"=w2775) -> ("编码输出"=w2772:string)  [unwired: 6 in]
              n988 = call "核查数据编码整合输出.vi"("字段结束"=FALSE, "数据标识"="N" ("字符串"), "数据类型"="-StandardValue=", "污染物编码"="w01019", "数据值"=w2763) -> ("编码输出"=w2767:string)  [unwired: 6 in]
              n989 = call "核查数据编码整合输出.vi"("字段结束"=TRUE, "数据标识"="N" ("字符串"), "数据类型"="-SpanValue=", "污染物编码"="w01019", "数据值"="0") -> ("编码输出"=w2762:string)  [unwired: 6 in]
              n990 = Concatenate Strings(w2772, w2767, w2762) -> (w2771:string)
            }
          }
          n991 = call "规范时间戳.vi"("字符串"=w2640) -> ("result string"=w2639:string)  [unwired: 10 in]
          n992 = Format Into String(format string="DataTime=%s;%s%s%s%s%s" ("格式字符串"), w2639, w2638, w2633, w2631, w2629, w2624) -> (resulting string=w2642:string)  [unwired: 2 in, 1 out]
          n993 = Empty String/Path?(string/path=w2639) -> (empty?=w2643:bool)
          n994 = case shown="假" w2643 {
            tunnel: [w2779 ""] -> w2641
            tunnel: w2642 -> [w2779 _]
            frame False {
              n995 = global read "全局 小时数据发送次数.vi" "小时数据发送次数"() -> (w2778:i32)
              n996 = Increment(x=w2778) -> (x+1=w2777:i32)
              n997 = global write "全局 小时数据发送次数.vi" "小时数据发送次数"(w2777) -> ()
            }
            frame True {
              n998 = global read "全局 小时数据发送次数.vi" "小时数据发送次数"() -> (w2781:i32)
              n999 = Increment(x=w2781) -> (x+1=w2780:i32)
              n1000 = global write "全局 小时数据发送次数.vi" "小时数据发送次数"(w2780) -> ()
            }
          }
        }
        frame "返回执行结果" {
        }
      }
    }
    frame "提取加标回收" {
      # "提取加标回收数据"
      n1001 = global read "全局1.vi" "枚举"() -> (w2790:enum16{"返回请求应答", "上传数据", "返回执行结果"})
      n1002 = case shown="\"上传数据\"" w2790 {
        tunnel: ["QnRtn=1" w3019 "ExeRtn=1"] -> w2784
        tunnel: w2788 -> [_ w3021 _]
        tunnel: w2789 -> [_ w2827 _]
        tunnel: w2787 -> [_ w2826 _]
        tunnel: w2786 -> [_ w2825 _]
        tunnel: w2785 -> [_ w2824 _]
        frame "返回请求应答", Default {
          n1003 = global read "全局 数据数组大小.vi" "数据数组大小"() -> (w2791:i32)
          n1004 = Equal To 0?(x=w2791) -> (x = 0?=w2792:bool)
          n1005 = case shown="真" w2792 {
            frame False {
            }
            frame True {
              n1006 = global read "全局 小时数据发送次数.vi" "小时数据发送次数"() -> (w2795:i32)
              n1007 = Increment(x=w2795) -> (x+1=w2794:i32)
              n1008 = global write "全局 小时数据发送次数.vi" "小时数据发送次数"(w2794) -> ()
            }
          }
        }
        frame "上传数据" {
          # "w01001-Check=63.0,w01001-WaterTime=20160801080000,w01001-Water=45.23,w01001-Chroma=1000,w01001-Volume=0.2,w01001-DVolume=200,w01003-Flag=N;"
          # "CODCr"
          # "总氮"
          # "总磷"
          # "NH3"
          # "CODMn"
          n1009 = global read "全局 小时数据发送次数.vi" "小时数据发送次数"() -> (w3022:i32)
          n1010 = Index Array(array=w2825, index (row)=w3022) -> (element=w2815:string[])  [unwired: 1 in]
          n1011 = Index Array(array=w3021, index (row)=w3022) -> (element=w3026:string[])  [unwired: 1 in]
          n1012 = Index Array(array=w2827, index (row)=w3022) -> (element=w2822:string[])  [unwired: 1 in]
          n1013 = Index Array(array=w2815, index #1=4 ("索引"), index #2=2 ("索引"), index #3=3 ("索引"), index #4=5 ("索引"), index #5=6 ("索引"), index #6=7 ("索引")) -> (element #1=w2807:string, element #2=w2806:string, element #3=w2805:string, element #4=w2804:string, element #5=w2803:string, element #6=w2802:string)
          n1014 = Index Array(array=w2826, index (row)=w3022) -> (element=w2823:string[])  [unwired: 1 in]
          n1015 = Index Array(array=w2824, index (row)=w3022) -> (element=w2814:string[])  [unwired: 1 in]
          n1016 = Index Array(array=w2822, index #1=4 ("索引"), index #2=2 ("索引"), index #3=3 ("索引"), index #4=5 ("索引"), index #5=6 ("索引"), index #6=7 ("索引")) -> (element #1=w2821:string, element #2=w2820:string, element #3=w2819:string, element #4=w2818:string, element #5=w2817:string, element #6=w2816:string)
          n1017 = Index Array(array=w3026, index #1=0 ("索引"), index #2=4 ("索引"), index #3=2 ("索引"), index #4=3 ("索引"), index #5=5 ("索引"), index #6=6 ("索引"), index #7=7 ("索引")) -> (element #1=w3024:string, element #2=w3016:string, element #3=w2860:string, element #4=w3008:string, element #5=w3005:string, element #6=w3001:string, element #7=w3000:string)
          n1018 = Index Array(array=w2823, index #1=4 ("索引"), index #2=2 ("索引"), index #3=3 ("索引"), index #4=5 ("索引"), index #5=6 ("索引"), index #6=7 ("索引")) -> (element #1=w2813:string, element #2=w2812:string, element #3=w2811:string, element #4=w2810:string, element #5=w2809:string, element #6=w2808:string)
          n1019 = Index Array(array=w2814, index #1=4 ("索引"), index #2=2 ("索引"), index #3=3 ("索引"), index #4=5 ("索引"), index #5=6 ("索引"), index #6=7 ("索引")) -> (element #1=w2801:string, element #2=w2800:string, element #3=w2799:string, element #4=w2798:string, element #5=w2797:string, element #6=w2796:string)
          n1020 = call "规范时间戳.vi"("字符串"=w3024) -> ("result string"=w3023:string)  [unwired: 10 in]
          n1021 = call "规范时间戳.vi"("字符串"=w2860) -> ("result string"=w2859:string)  [unwired: 10 in]
          n1022 = call "规范时间戳.vi"("字符串"=w2806) -> ("result string"=w2836:string)  [unwired: 10 in]
          n1023 = call "规范时间戳.vi"("字符串"=w2812) -> ("result string"=w2837:string)  [unwired: 10 in]
          n1024 = call "规范时间戳.vi"("字符串"=w2820) -> ("result string"=w2838:string)  [unwired: 10 in]
          n1025 = call "规范时间戳.vi"("字符串"=w2800) -> ("result string"=w2835:string)  [unwired: 10 in]
          n1026 = call "核查数据编码整合输出.vi"("字段结束"=FALSE, "数据标识"="N" ("字符串"), "数据类型"="-Check=", "污染物编码"="w21011", "数据值"=w2813) -> ("编码输出"=w2953:string)  [unwired: 6 in]
          n1027 = call "核查数据编码整合输出.vi"("字段结束"=FALSE, "数据标识"="N" ("字符串"), "数据类型"="-WaterTime=", "污染物编码"="w21011", "数据值"=w2837) -> ("编码输出"=w2936:string)  [unwired: 6 in]
          n1028 = call "核查数据编码整合输出.vi"("字段结束"=FALSE, "数据标识"="N" ("字符串"), "数据类型"="-Water=", "污染物编码"="w21011", "数据值"=w2811) -> ("编码输出"=w2935:string)  [unwired: 6 in]
          n1029 = call "核查数据编码整合输出.vi"("字段结束"=TRUE, "数据标识"="N" ("字符串"), "数据类型"="-DVolume=", "污染物编码"="w21011", "数据值"=w2808) -> ("编码输出"=w2932:string)  [unwired: 6 in]
          n1030 = call "核查数据编码整合输出.vi"("字段结束"=FALSE, "数据标识"="N" ("字符串"), "数据类型"="-Chroma=", "污染物编码"="w21011", "数据值"=w2810) -> ("编码输出"=w2934:string)  [unwired: 6 in]
          n1031 = call "核查数据编码整合输出.vi"("字段结束"=FALSE, "数据标识"="N" ("字符串"), "数据类型"="-Volume=", "污染物编码"="w21011", "数据值"=w2809) -> ("编码输出"=w2933:string)  [unwired: 6 in]
          n1032 = call "核查数据编码整合输出.vi"("字段结束"=FALSE, "数据标识"="N" ("字符串"), "数据类型"="-WaterTime=", "污染物编码"="w21001", "数据值"=w2836) -> ("编码输出"=w2916:string)  [unwired: 6 in]
          n1033 = call "核查数据编码整合输出.vi"("字段结束"=FALSE, "数据类型"="-Volume=", "污染物编码"="w01019", "数据值"=w3001) -> ("编码输出"=w2993:string)  [unwired: 7 in]
          n1034 = call "核查数据编码整合输出.vi"("字段结束"=FALSE, "数据标识"="N" ("字符串"), "数据类型"="-Check=", "污染物编码"="w21001", "数据值"=w2807) -> ("编码输出"=w2917:string)  [unwired: 6 in]
          n1035 = call "核查数据编码整合输出.vi"("字段结束"=FALSE, "数据标识"="N" ("字符串"), "数据类型"="-Water=", "污染物编码"="w21001", "数据值"=w2805) -> ("编码输出"=w2915:string)  [unwired: 6 in]
          n1036 = call "核查数据编码整合输出.vi"("字段结束"=FALSE, "数据标识"="N" ("字符串"), "数据类型"="-Chroma=", "污染物编码"="w21001", "数据值"=w2804) -> ("编码输出"=w2914:string)  [unwired: 6 in]
          n1037 = call "核查数据编码整合输出.vi"("字段结束"=FALSE, "数据标识"="N" ("字符串"), "数据类型"="-Volume=", "污染物编码"="w21001", "数据值"=w2803) -> ("编码输出"=w2913:string)  [unwired: 6 in]
          n1038 = call "核查数据编码整合输出.vi"("字段结束"=TRUE, "数据标识"="N" ("字符串"), "数据类型"="-DVolume=", "污染物编码"="w21001", "数据值"=w2802) -> ("编码输出"=w2912:string)  [unwired: 6 in]
          n1039 = call "核查数据编码整合输出.vi"("字段结束"=TRUE, "数据类型"="-DVolume=", "污染物编码"="w01019", "数据值"=w3000) -> ("编码输出"=w2992:string)  [unwired: 7 in]
          n1040 = call "核查数据编码整合输出.vi"("字段结束"=FALSE, "数据类型"="-Chroma=", "污染物编码"="w01019", "数据值"=w3005) -> ("编码输出"=w2994:string)  [unwired: 7 in]
          n1041 = call "核查数据编码整合输出.vi"("字段结束"=FALSE, "数据标识"="N" ("字符串"), "数据类型"="-Check=", "污染物编码"="w21003", "数据值"=w2821) -> ("编码输出"=w2966:string)  [unwired: 6 in]
          n1042 = call "核查数据编码整合输出.vi"("字段结束"=FALSE, "数据标识"="N" ("字符串"), "数据类型"="-WaterTime=", "污染物编码"="w21003", "数据值"=w2838) -> ("编码输出"=w2965:string)  [unwired: 6 in]
          n1043 = call "核查数据编码整合输出.vi"("字段结束"=FALSE, "数据标识"="N" ("字符串"), "数据类型"="-Check=", "污染物编码"="w01019", "数据值"=w3016) -> ("编码输出"=w2997:string)  [unwired: 6 in]
          n1044 = call "核查数据编码整合输出.vi"("字段结束"=FALSE, "数据类型"="-WaterTime=", "污染物编码"="w01019", "数据值"=w2859) -> ("编码输出"=w2996:string)  [unwired: 7 in]
          n1045 = call "核查数据编码整合输出.vi"("字段结束"=FALSE, "数据标识"="N" ("字符串"), "数据类型"="-Water=", "污染物编码"="w21003", "数据值"=w2819) -> ("编码输出"=w2964:string)  [unwired: 6 in]
          n1046 = call "核查数据编码整合输出.vi"("字段结束"=FALSE, "数据类型"="-Water=", "污染物编码"="w01019", "数据值"=w3008) -> ("编码输出"=w2995:string)  [unwired: 7 in]
          n1047 = call "核查数据编码整合输出.vi"("字段结束"=FALSE, "数据标识"="N" ("字符串"), "数据类型"="-Chroma=", "污染物编码"="w21003", "数据值"=w2818) -> ("编码输出"=w2963:string)  [unwired: 6 in]
          n1048 = call "核查数据编码整合输出.vi"("字段结束"=FALSE, "数据标识"="N" ("字符串"), "数据类型"="-Volume=", "污染物编码"="w21003", "数据值"=w2817) -> ("编码输出"=w2962:string)  [unwired: 6 in]
          n1049 = call "核查数据编码整合输出.vi"("字段结束"=TRUE, "数据标识"="N" ("字符串"), "数据类型"="-DVolume=", "污染物编码"="w21003", "数据值"=w2816) -> ("编码输出"=w2961:string)  [unwired: 6 in]
          n1050 = call "核查数据编码整合输出.vi"("字段结束"=FALSE, "数据标识"="N" ("字符串"), "数据类型"="-Check=", "污染物编码"="w01018", "数据值"=w2801) -> ("编码输出"=w2889:string)  [unwired: 6 in]
          n1051 = call "核查数据编码整合输出.vi"("字段结束"=FALSE, "数据标识"="N" ("字符串"), "数据类型"="-Water=", "污染物编码"="w01018", "数据值"=w2799) -> ("编码输出"=w2887:string)  [unwired: 6 in]
          n1052 = call "核查数据编码整合输出.vi"("字段结束"=FALSE, "数据标识"="N" ("字符串"), "数据类型"="-WaterTime=", "污染物编码"="w01018", "数据值"=w2835) -> ("编码输出"=w2888:string)  [unwired: 6 in]
          n1053 = call "核查数据编码整合输出.vi"("字段结束"=FALSE, "数据标识"="N" ("字符串"), "数据类型"="-Chroma=", "污染物编码"="w01018", "数据值"=w2798) -> ("编码输出"=w2886:string)  [unwired: 6 in]
          n1054 = call "核查数据编码整合输出.vi"("字段结束"=FALSE, "数据标识"="N" ("字符串"), "数据类型"="-Volume=", "污染物编码"="w01018", "数据值"=w2797) -> ("编码输出"=w2885:string)  [unwired: 6 in]
          n1055 = call "核查数据编码整合输出.vi"("字段结束"=TRUE, "数据标识"="N" ("字符串"), "数据类型"="-DVolume=", "污染物编码"="w01018", "数据值"=w2796) -> ("编码输出"=w2884:string)  [unwired: 6 in]
          n1056 = Concatenate Strings(w2953, w2936, w2935, w2934, w2933, w2932) -> (w2928:string)
          n1057 = Concatenate Strings(w2997, w2996, w2995, w2994, w2993, w2992) -> (w2991:string)
          n1058 = Concatenate Strings(w2966, w2965, w2964, w2963, w2962, w2961) -> (w2960:string)
          n1059 = Concatenate Strings(w2917, w2916, w2915, w2914, w2913, w2912) -> (w2871:string)
          n1060 = Empty String/Path?(string/path=w3023) -> (empty?=w3018:bool)
          n1061 = Concatenate Strings(w2889, w2888, w2887, w2886, w2885, w2884) -> (w2870:string)
          n1062 = Format Into String(format string="DataTime=%s;%s%s%s%s%s" ("格式字符串"), w3023, w2991, w2960, w2928, w2871, w2870) -> (resulting string=w3020:string)  [unwired: 2 in, 1 out]
          n1063 = case shown="真" w3018 {
            tunnel: [w3031 ""] -> w3019
            tunnel: w3020 -> [w3031 _]
            frame False {
              n1064 = global read "全局 小时数据发送次数.vi" "小时数据发送次数"() -> (w3030:i32)
              n1065 = Increment(x=w3030) -> (x+1=w3029:i32)
              n1066 = global write "全局 小时数据发送次数.vi" "小时数据发送次数"(w3029) -> ()
            }
            frame True {
              n1067 = global read "全局 小时数据发送次数.vi" "小时数据发送次数"() -> (w3033:i32)
              n1068 = Increment(x=w3033) -> (x+1=w3032:i32)
              n1069 = global write "全局 小时数据发送次数.vi" "小时数据发送次数"(w3032) -> ()
            }
          }
        }
        frame "返回执行结果" {
        }
      }
    }
    frame "提取平行样" {
      # "提取平行样数据"
      n1070 = global read "全局1.vi" "枚举"() -> (w3042:enum16{"返回请求应答", "上传数据", "返回执行结果"})
      n1071 = case shown="\"返回请求应答\", 默认" w3042 {
        tunnel: ["QnRtn=1" w3100 "ExeRtn=1"] -> w3041
        tunnel: w3040 -> [_ w3092 _]
        tunnel: w3039 -> [_ w3103 _]
        tunnel: w3038 -> [_ w3102 _]
        tunnel: w3036 -> [_ w3060 _]
        tunnel: w3037 -> [_ w3050 _]
        frame "返回请求应答", Default {
          n1072 = global read "全局 数据数组大小.vi" "数据数组大小"() -> (w3043:i32)
          n1073 = Equal To 0?(x=w3043) -> (x = 0?=w3044:bool)
          n1074 = case shown="真" w3044 {
            frame False {
            }
            frame True {
              n1075 = global read "全局 小时数据发送次数.vi" "小时数据发送次数"() -> (w3047:i32)
              n1076 = Increment(x=w3047) -> (x+1=w3046:i32)
              n1077 = global write "全局 小时数据发送次数.vi" "小时数据发送次数"(w3046) -> ()
            }
          }
        }
        frame "上传数据" {
          # "CODMn"
          n1078 = global read "全局 小时数据发送次数.vi" "小时数据发送次数"() -> (w3048:i32)
          n1079 = Index Array(array=w3092, index (row)=w3048) -> (element=w3097:string[])  [unwired: 1 in]
          n1080 = Index Array(array=w3050, index (row)=w3048) -> (element=w3054:string[])  [unwired: 1 in]
          n1081 = Index Array(array=w3102, index (row)=w3048) -> (element=w3073:string[])  [unwired: 1 in]
          n1082 = Index Array(array=w3060, index (row)=w3048) -> (element=w3065:string[])  [unwired: 1 in]
          n1083 = Index Array(array=w3103, index (row)=w3048) -> (element=w3082:string[])  [unwired: 1 in]
          n1084 = Index Array(array=w3054, index #1=0 ("索引"), index #2=2 ("索引"), index #3=3 ("索引"), index #4=4 ("索引")) -> (element #2=w3051:string, element #3=w3053:string, element #4=w3052:string)  [unwired: 1 out]
          n1085 = Index Array(array=w3073, index #1=0 ("索引"), index #2=2 ("索引"), index #3=3 ("索引"), index #4=4 ("索引")) -> (element #2=w3070:string, element #3=w3072:string, element #4=w3071:string)  [unwired: 1 out]
          n1086 = Index Array(array=w3065, index #1=0 ("索引"), index #2=2 ("索引"), index #3=3 ("索引"), index #4=4 ("索引")) -> (element #2=w3068:string, element #3=w3066:string, element #4=w3067:string)  [unwired: 1 out]
          n1087 = Index Array(array=w3097, index #1=0 ("索引"), index #2=2 ("索引"), index #3=3 ("索引"), index #4=4 ("索引")) -> (element #1=w3090:string, element #2=w3088:string, element #3=w3093:string, element #4=w3095:string)
          n1088 = Index Array(array=w3082, index #1=0 ("索引"), index #2=2 ("索引"), index #3=3 ("索引"), index #4=4 ("索引")) -> (element #2=w3079:string, element #3=w3081:string, element #4=w3080:string)  [unwired: 1 out]
          n1089 = call "规范时间戳.vi"("字符串"=w3090) -> ("result string"=w3091:string)  [unwired: 10 in]
          n1090 = case shown="\"真\", 默认" w3051 {
            selector: w3051 -> [w3105 _]
            tunnel: w3051 -> [_ w3122]
            tunnel: w3052 -> [_ w3114]
            tunnel: w3053 -> [_ w3111]
            tunnel: [w3105 w3106] -> w3049
            frame "" {
            }
            frame "真", Default {
              # "CODCr"
              n1091 = call "规范时间戳.vi"("字符串"=w3111) -> ("result string"=w3110:string)  [unwired: 10 in]
              n1092 = call "核查数据编码整合输出.vi"("字段结束"=FALSE, "数据标识"="N" ("字符串"), "数据类型"="-Check=", "污染物编码"="w01018", "数据值"=w3122) -> ("编码输出"=w3109:string)  [unwired: 6 in]
              n1093 = call "核查数据编码整合输出.vi"("字段结束"=FALSE, "数据类型"="-WaterTime=", "污染物编码"="w01018", "数据值"=w3110) -> ("编码输出"=w3108:string)  [unwired: 7 in]
              n1094 = call "核查数据编码整合输出.vi"("字段结束"=TRUE, "数据类型"="-Water=", "污染物编码"="w01018", "数据值"=w3114) -> ("编码输出"=w3107:string)  [unwired: 7 in]
              n1095 = Concatenate Strings(w3109, w3108, w3107) -> (w3106:string)
            }
          }
          n1096 = case shown="\"真\", 默认" w3088 {
            selector: w3088 -> [w3181 _]
            tunnel: w3088 -> [_ w3198]
            tunnel: w3095 -> [_ w3190]
            tunnel: w3093 -> [_ w3187]
            tunnel: [w3181 w3182] -> w3087
            frame "" {
            }
            frame "真", Default {
              # "CODMn"
              n1097 = call "规范时间戳.vi"("字符串"=w3187) -> ("result string"=w3186:string)  [unwired: 10 in]
              n1098 = call "核查数据编码整合输出.vi"("字段结束"=FALSE, "数据标识"="N" ("字符串"), "数据类型"="-Check=", "污染物编码"="w01019", "数据值"=w3198) -> ("编码输出"=w3185:string)  [unwired: 6 in]
              n1099 = call "核查数据编码整合输出.vi"("字段结束"=FALSE, "数据类型"="-WaterTime=", "污染物编码"="w01019", "数据值"=w3186) -> ("编码输出"=w3184:string)  [unwired: 7 in]
              n1100 = call "核查数据编码整合输出.vi"("字段结束"=TRUE, "数据类型"="-Water=", "污染物编码"="w01019", "数据值"=w3190) -> ("编码输出"=w3183:string)  [unwired: 7 in]
              n1101 = Concatenate Strings(w3185, w3184, w3183) -> (w3182:string)
            }
          }
          n1102 = case shown="\"真\", 默认" w3079 {
            selector: w3079 -> [w3162 _]
            tunnel: w3079 -> [_ w3179]
            tunnel: w3080 -> [_ w3171]
            tunnel: w3081 -> [_ w3168]
            tunnel: [w3162 w3163] -> w3078
            frame "" {
            }
            frame "真", Default {
              # "NH3"
              n1103 = call "规范时间戳.vi"("字符串"=w3168) -> ("result string"=w3167:string)  [unwired: 10 in]
              n1104 = call "核查数据编码整合输出.vi"("字段结束"=FALSE, "数据标识"="N" ("字符串"), "数据类型"="-Check=", "污染物编码"="w21003", "数据值"=w3179) -> ("编码输出"=w3166:string)  [unwired: 6 in]
              n1105 = call "核查数据编码整合输出.vi"("字段结束"=FALSE, "数据类型"="-WaterTime=", "污染物编码"="w21003", "数据值"=w3167) -> ("编码输出"=w3165:string)  [unwired: 7 in]
              n1106 = call "核查数据编码整合输出.vi"("字段结束"=TRUE, "数据类型"="-Water=", "污染物编码"="w21003", "数据值"=w3171) -> ("编码输出"=w3164:string)  [unwired: 7 in]
              n1107 = Concatenate Strings(w3166, w3165, w3164) -> (w3163:string)
            }
          }
          n1108 = case shown="\"真\", 默认" w3070 {
            selector: w3070 -> [w3143 _]
            tunnel: w3070 -> [_ w3160]
            tunnel: w3071 -> [_ w3152]
            tunnel: w3072 -> [_ w3149]
            tunnel: [w3143 w3144] -> w3069
            frame "" {
            }
            frame "真", Default {
              # "总磷"
              n1109 = call "规范时间戳.vi"("字符串"=w3149) -> ("result string"=w3148:string)  [unwired: 10 in]
              n1110 = call "核查数据编码整合输出.vi"("字段结束"=FALSE, "数据标识"="N" ("字符串"), "数据类型"="-Check=", "污染物编码"="w21011", "数据值"=w3160) -> ("编码输出"=w3147:string)  [unwired: 6 in]
              n1111 = call "核查数据编码整合输出.vi"("字段结束"=FALSE, "数据类型"="-WaterTime=", "污染物编码"="w21011", "数据值"=w3148) -> ("编码输出"=w3146:string)  [unwired: 7 in]
              n1112 = call "核查数据编码整合输出.vi"("字段结束"=TRUE, "数据类型"="-Water=", "污染物编码"="w21011", "数据值"=w3152) -> ("编码输出"=w3145:string)  [unwired: 7 in]
              n1113 = Concatenate Strings(w3147, w3146, w3145) -> (w3144:string)
            }
          }
          n1114 = case shown="\"真\", 默认" w3068 {
            selector: w3068 -> [w3124 _]
            tunnel: w3068 -> [_ w3141]
            tunnel: w3067 -> [_ w3133]
            tunnel: w3066 -> [_ w3130]
            tunnel: [w3124 w3125] -> w3059
            frame "" {
            }
            frame "真", Default {
              # "总氮"
              n1115 = call "规范时间戳.vi"("字符串"=w3130) -> ("result string"=w3129:string)  [unwired: 10 in]
              n1116 = call "核查数据编码整合输出.vi"("字段结束"=FALSE, "数据标识"="N" ("字符串"), "数据类型"="-Check=", "污染物编码"="w21001", "数据值"=w3141) -> ("编码输出"=w3128:string)  [unwired: 6 in]
              n1117 = call "核查数据编码整合输出.vi"("字段结束"=FALSE, "数据类型"="-WaterTime=", "污染物编码"="w21001", "数据值"=w3129) -> ("编码输出"=w3127:string)  [unwired: 7 in]
              n1118 = call "核查数据编码整合输出.vi"("字段结束"=TRUE, "数据类型"="-Water=", "污染物编码"="w21001", "数据值"=w3133) -> ("编码输出"=w3126:string)  [unwired: 7 in]
              n1119 = Concatenate Strings(w3128, w3127, w3126) -> (w3125:string)
            }
          }
          n1120 = Empty String/Path?(string/path=w3090) -> (empty?=w3099:bool)
          n1121 = Format Into String(format string="DataTime=%s;%s%s%s%s%s" ("格式字符串"), w3091, w3087, w3078, w3069, w3059, w3049) -> (resulting string=w3101:string)  [unwired: 2 in, 1 out]
          n1122 = case shown="真" w3099 {
            tunnel: [w3202 ""] -> w3100
            tunnel: w3101 -> [w3202 _]
            frame False {
              n1123 = global read "全局 小时数据发送次数.vi" "小时数据发送次数"() -> (w3201:i32)
              n1124 = Increment(x=w3201) -> (x+1=w3200:i32)
              n1125 = global write "全局 小时数据发送次数.vi" "小时数据发送次数"(w3200) -> ()
            }
            frame True {
              n1126 = global read "全局 小时数据发送次数.vi" "小时数据发送次数"() -> (w3204:i32)
              n1127 = Increment(x=w3204) -> (x+1=w3203:i32)
              n1128 = global write "全局 小时数据发送次数.vi" "小时数据发送次数"(w3203) -> ()
            }
          }
        }
        frame "返回执行结果" {
        }
      }
    }
    frame "提取集成干预" {
      # "提取平行样数据"
      n1129 = global read "全局1.vi" "枚举"() -> (w3218:enum16{"返回请求应答", "上传数据", "返回执行结果"})
      n1130 = case shown="\"返回请求应答\", 默认" w3218 {
        tunnel: ["QnRtn=1" w3327 "ExeRtn=1"] -> w3217
        tunnel: w3216 -> [_ w3319 _]
        tunnel: w3215 -> [_ w3305 _]
        tunnel: w3209 -> [_ w3295 _]
        tunnel: w3210 -> [_ w3285 _]
        tunnel: w3211 -> [_ w3265 _]
        tunnel: w3208 -> [_ w3255 _]
        tunnel: w3207 -> [_ w3256 _]
        tunnel: w3212 -> [_ w3245 _]
        tunnel: w3214 -> [_ w3236 _]
        tunnel: w3213 -> [_ w3224 _]
        frame "返回请求应答", Default {
          n1131 = global read "全局 数据数组大小.vi" "数据数组大小"() -> (w3219:i32)
          n1132 = Equal To 0?(x=w3219) -> (x = 0?=w3220:bool)
          n1133 = case shown="真" w3220 {
            frame False {
            }
            frame True {
              n1134 = global read "全局 小时数据发送次数.vi" "小时数据发送次数"() -> (w3223:i32)
              n1135 = Increment(x=w3223) -> (x+1=w3222:i32)
              n1136 = global write "全局 小时数据发送次数.vi" "小时数据发送次数"(w3222) -> ()
            }
          }
        }
        frame "上传数据" {
          # "CODMn"
          n1137 = global read "全局 小时数据发送次数.vi" "小时数据发送次数"() -> (w3235:i32)
          n1138 = Index Array(array=w3319, index (row)=w3235) -> (element=w3324:string[])  [unwired: 1 in]
          n1139 = Index Array(array=w3255, index (row)=w3235) -> (element=w3270:string[])  [unwired: 1 in]
          n1140 = Index Array(array=w3256, index (row)=w3235) -> (element=w3260:string[])  [unwired: 1 in]
          n1141 = Index Array(array=w3236, index (row)=w3235) -> (element=w3241:string[])  [unwired: 1 in]
          n1142 = Index Array(array=w3245, index (row)=w3235) -> (element=w3249:string[])  [unwired: 1 in]
          n1143 = Index Array(array=w3265, index (row)=w3235) -> (element=w3279:string[])  [unwired: 1 in]
          n1144 = Index Array(array=w3285, index (row)=w3235) -> (element=w3289:string[])  [unwired: 1 in]
          n1145 = Index Array(array=w3224) -> (element=w3231:string[])  [unwired: 2 in]
          n1146 = Index Array(array=w3295, index (row)=w3235) -> (element=w3299:string[])  [unwired: 1 in]
          n1147 = Index Array(array=w3305, index (row)=w3235) -> (element=w3309:string[])  [unwired: 1 in]
          n1148 = Index Array(array=w3270, index #1=0 ("索引"), index #2=2 ("索引"), index #3=3 ("索引"), index #4=4 ("索引")) -> (element #2=w3267:string, element #3=w3269:string, element #4=w3268:string)  [unwired: 1 out]
          n1149 = Index Array(array=w3260, index #1=0 ("索引"), index #2=2 ("索引"), index #3=3 ("索引"), index #4=4 ("索引")) -> (element #2=w3257:string, element #3=w3259:string, element #4=w3258:string)  [unwired: 1 out]
          n1150 = Index Array(array=w3241, index #1=0 ("索引"), index #2=2 ("索引"), index #3=3 ("索引"), index #4=4 ("索引")) -> (element #2=w3244:string, element #3=w3242:string, element #4=w3243:string)  [unwired: 1 out]
          n1151 = Index Array(array=w3249, index #1=0 ("索引"), index #2=2 ("索引"), index #3=3 ("索引"), index #4=4 ("索引")) -> (element #2=w3246:string, element #3=w3248:string, element #4=w3247:string)  [unwired: 1 out]
          n1152 = Index Array(array=w3279, index #1=0 ("索引"), index #2=2 ("索引"), index #3=3 ("索引"), index #4=4 ("索引")) -> (element #2=w3276:string, element #3=w3278:string, element #4=w3277:string)  [unwired: 1 out]
          n1153 = Index Array(array=w3289, index #1=0 ("索引"), index #2=2 ("索引"), index #3=3 ("索引"), index #4=4 ("索引")) -> (element #2=w3286:string, element #3=w3288:string, element #4=w3287:string)  [unwired: 1 out]
          n1154 = Index Array(array=w3231, index #1=0 ("索引"), index #2=2 ("索引"), index #4=4 ("索引")) -> (element #2=w3234:string, element #3=w3232:string, element #4=w3233:string)  [unwired: 1 in, 1 out]
          n1155 = Index Array(array=w3299, index #1=0 ("索引"), index #2=2 ("索引"), index #3=3 ("索引"), index #4=4 ("索引")) -> (element #2=w3296:string, element #3=w3298:string, element #4=w3297:string)  [unwired: 1 out]
          n1156 = Index Array(array=w3309, index #1=0 ("索引"), index #2=2 ("索引"), index #3=3 ("索引"), index #4=4 ("索引")) -> (element #2=w3306:string, element #3=w3308:string, element #4=w3307:string)  [unwired: 1 out]
          n1157 = Index Array(array=w3324, index #1=0 ("索引"), index #2=2 ("索引"), index #3=3 ("索引"), index #4=4 ("索引")) -> (element #1=w3317:string, element #2=w3315:string, element #3=w3320:string, element #4=w3322:string)
          n1158 = call "规范时间戳.vi"("字符串"=w3317) -> ("result string"=w3318:string)  [unwired: 10 in]
          n1159 = case shown="\"真\", 默认" w3267 {
            selector: w3267 -> [w3406 _]
            tunnel: w3267 -> [_ w3423]
            tunnel: w3268 -> [_ w3415]
            tunnel: w3269 -> [_ w3412]
            tunnel: [w3406 w3407] -> w3266
            frame "" {
            }
            frame "真", Default {
              # "电导率"
              n1160 = call "规范时间戳.vi"("字符串"=w3412) -> ("result string"=w3411:string)  [unwired: 10 in]
              n1161 = call "核查数据编码整合输出.vi"("字段结束"=FALSE, "数据标识"="N" ("字符串"), "数据类型"="-Check=", "污染物编码"="w01014", "数据值"=w3423) -> ("编码输出"=w3410:string)  [unwired: 6 in]
              n1162 = call "核查数据编码整合输出.vi"("字段结束"=FALSE, "数据类型"="-WaterTime=", "污染物编码"="w01014", "数据值"=w3411) -> ("编码输出"=w3409:string)  [unwired: 7 in]
              n1163 = call "核查数据编码整合输出.vi"("字段结束"=TRUE, "数据类型"="-Water=", "污染物编码"="w01014", "数据值"=w3415) -> ("编码输出"=w3408:string)  [unwired: 7 in]
              n1164 = Concatenate Strings(w3410, w3409, w3408) -> (w3407:string)
            }
          }
          n1165 = case shown="\"真\", 默认" w3257 {
            selector: w3257 -> [w3387 _]
            tunnel: w3257 -> [_ w3404]
            tunnel: w3258 -> [_ w3396]
            tunnel: w3259 -> [_ w3393]
            tunnel: [w3387 w3388] -> w3254
            frame "" {
            }
            frame "真", Default {
              # "浊度"
              n1166 = call "规范时间戳.vi"("字符串"=w3393) -> ("result string"=w3392:string)  [unwired: 10 in]
              n1167 = call "核查数据编码整合输出.vi"("字段结束"=FALSE, "数据标识"="N" ("字符串"), "数据类型"="-Check=", "污染物编码"="w01003", "数据值"=w3404) -> ("编码输出"=w3391:string)  [unwired: 6 in]
              n1168 = call "核查数据编码整合输出.vi"("字段结束"=FALSE, "数据类型"="-WaterTime=", "污染物编码"="w01003", "数据值"=w3392) -> ("编码输出"=w3390:string)  [unwired: 7 in]
              n1169 = call "核查数据编码整合输出.vi"("字段结束"=TRUE, "数据类型"="-Water=", "污染物编码"="w01003", "数据值"=w3396) -> ("编码输出"=w3389:string)  [unwired: 7 in]
              n1170 = Concatenate Strings(w3391, w3390, w3389) -> (w3388:string)
            }
          }
          n1171 = case shown="\"真\", 默认" w3244 {
            selector: w3244 -> [w3349 _]
            tunnel: w3244 -> [_ w3366]
            tunnel: w3243 -> [_ w3358]
            tunnel: w3242 -> [_ w3355]
            tunnel: [w3349 w3350] -> w3226
            frame "" {
            }
            frame "真", Default {
              # "总氮"
              n1172 = call "规范时间戳.vi"("字符串"=w3355) -> ("result string"=w3354:string)  [unwired: 10 in]
              n1173 = call "核查数据编码整合输出.vi"("字段结束"=FALSE, "数据标识"="N" ("字符串"), "数据类型"="-Check=", "污染物编码"="w21001", "数据值"=w3366) -> ("编码输出"=w3353:string)  [unwired: 6 in]
              n1174 = call "核查数据编码整合输出.vi"("字段结束"=FALSE, "数据类型"="-WaterTime=", "污染物编码"="w21001", "数据值"=w3354) -> ("编码输出"=w3352:string)  [unwired: 7 in]
              n1175 = call "核查数据编码整合输出.vi"("字段结束"=TRUE, "数据类型"="-Water=", "污染物编码"="w21001", "数据值"=w3358) -> ("编码输出"=w3351:string)  [unwired: 7 in]
              n1176 = Concatenate Strings(w3353, w3352, w3351) -> (w3350:string)
            }
          }
          n1177 = case shown="\"真\", 默认" w3246 {
            selector: w3246 -> [w3368 _]
            tunnel: w3246 -> [_ w3385]
            tunnel: w3247 -> [_ w3377]
            tunnel: w3248 -> [_ w3374]
            tunnel: [w3368 w3369] -> w3227
            frame "" {
            }
            frame "真", Default {
              # "总磷"
              n1178 = call "规范时间戳.vi"("字符串"=w3374) -> ("result string"=w3373:string)  [unwired: 10 in]
              n1179 = call "核查数据编码整合输出.vi"("字段结束"=FALSE, "数据标识"="N" ("字符串"), "数据类型"="-Check=", "污染物编码"="w21011", "数据值"=w3385) -> ("编码输出"=w3372:string)  [unwired: 6 in]
              n1180 = call "核查数据编码整合输出.vi"("字段结束"=FALSE, "数据类型"="-WaterTime=", "污染物编码"="w21011", "数据值"=w3373) -> ("编码输出"=w3371:string)  [unwired: 7 in]
              n1181 = call "核查数据编码整合输出.vi"("字段结束"=TRUE, "数据类型"="-Water=", "污染物编码"="w21011", "数据值"=w3377) -> ("编码输出"=w3370:string)  [unwired: 7 in]
              n1182 = Concatenate Strings(w3372, w3371, w3370) -> (w3369:string)
            }
          }
          n1183 = case shown="\"真\", 默认" w3276 {
            selector: w3276 -> [w3425 _]
            tunnel: w3276 -> [_ w3442]
            tunnel: w3277 -> [_ w3434]
            tunnel: w3278 -> [_ w3431]
            tunnel: [w3425 w3426] -> w3275
            frame "" {
            }
            frame "真", Default {
              # "DO"
              n1184 = call "规范时间戳.vi"("字符串"=w3431) -> ("result string"=w3430:string)  [unwired: 10 in]
              n1185 = call "核查数据编码整合输出.vi"("字段结束"=FALSE, "数据标识"="N" ("字符串"), "数据类型"="-Check=", "污染物编码"="w01009", "数据值"=w3442) -> ("编码输出"=w3429:string)  [unwired: 6 in]
              n1186 = call "核查数据编码整合输出.vi"("字段结束"=FALSE, "数据类型"="-WaterTime=", "污染物编码"="w01009", "数据值"=w3430) -> ("编码输出"=w3428:string)  [unwired: 7 in]
              n1187 = call "核查数据编码整合输出.vi"("字段结束"=TRUE, "数据类型"="-Water=", "污染物编码"="w01009", "数据值"=w3434) -> ("编码输出"=w3427:string)  [unwired: 7 in]
              n1188 = Concatenate Strings(w3429, w3428, w3427) -> (w3426:string)
            }
          }
          n1189 = case shown="\"真\", 默认" w3286 {
            selector: w3286 -> [w3444 _]
            tunnel: w3286 -> [_ w3461]
            tunnel: w3287 -> [_ w3453]
            tunnel: w3288 -> [_ w3450]
            tunnel: [w3444 w3445] -> w3284
            frame "" {
            }
            frame "真", Default {
              # "PH"
              n1190 = call "规范时间戳.vi"("字符串"=w3450) -> ("result string"=w3449:string)  [unwired: 10 in]
              n1191 = call "核查数据编码整合输出.vi"("字段结束"=FALSE, "数据标识"="N" ("字符串"), "数据类型"="-Check=", "污染物编码"="w01001", "数据值"=w3461) -> ("编码输出"=w3448:string)  [unwired: 6 in]
              n1192 = call "核查数据编码整合输出.vi"("字段结束"=FALSE, "数据类型"="-WaterTime=", "污染物编码"="w01001", "数据值"=w3449) -> ("编码输出"=w3447:string)  [unwired: 7 in]
              n1193 = call "核查数据编码整合输出.vi"("字段结束"=TRUE, "数据类型"="-Water=", "污染物编码"="w01001", "数据值"=w3453) -> ("编码输出"=w3446:string)  [unwired: 7 in]
              n1194 = Concatenate Strings(w3448, w3447, w3446) -> (w3445:string)
            }
          }
          n1195 = case shown="\"真\", 默认" w3234 {
            selector: w3234 -> [w3330 _]
            tunnel: w3234 -> [_ w3347]
            tunnel: w3233 -> [_ w3339]
            tunnel: w3232 -> [_ w3336]
            tunnel: [w3330 w3331] -> w3225
            frame "" {
            }
            frame "真", Default {
              # "CODCr"
              n1196 = call "规范时间戳.vi"("字符串"=w3336) -> ("result string"=w3335:string)  [unwired: 10 in]
              n1197 = call "核查数据编码整合输出.vi"("字段结束"=FALSE, "数据标识"="N" ("字符串"), "数据类型"="-Check=", "污染物编码"="w01018", "数据值"=w3347) -> ("编码输出"=w3334:string)  [unwired: 6 in]
              n1198 = call "核查数据编码整合输出.vi"("字段结束"=FALSE, "数据类型"="-WaterTime=", "污染物编码"="w01018", "数据值"=w3335) -> ("编码输出"=w3333:string)  [unwired: 7 in]
              n1199 = call "核查数据编码整合输出.vi"("字段结束"=TRUE, "数据类型"="-Water=", "污染物编码"="w01018", "数据值"=w3339) -> ("编码输出"=w3332:string)  [unwired: 7 in]
              n1200 = Concatenate Strings(w3334, w3333, w3332) -> (w3331:string)
            }
          }
          n1201 = case shown="\"真\", 默认" w3296 {
            selector: w3296 -> [w3463 _]
            tunnel: w3296 -> [_ w3480]
            tunnel: w3297 -> [_ w3472]
            tunnel: w3298 -> [_ w3469]
            tunnel: [w3463 w3464] -> w3294
            frame "" {
            }
            frame "真", Default {
              # "水温"
              n1202 = call "规范时间戳.vi"("字符串"=w3469) -> ("result string"=w3468:string)  [unwired: 10 in]
              n1203 = call "核查数据编码整合输出.vi"("字段结束"=FALSE, "数据标识"="N" ("字符串"), "数据类型"="-Check=", "污染物编码"="w01010", "数据值"=w3480) -> ("编码输出"=w3467:string)  [unwired: 6 in]
              n1204 = call "核查数据编码整合输出.vi"("字段结束"=FALSE, "数据类型"="-WaterTime=", "污染物编码"="w01010", "数据值"=w3468) -> ("编码输出"=w3466:string)  [unwired: 7 in]
              n1205 = call "核查数据编码整合输出.vi"("字段结束"=TRUE, "数据类型"="-Water=", "污染物编码"="w01010", "数据值"=w3472) -> ("编码输出"=w3465:string)  [unwired: 7 in]
              n1206 = Concatenate Strings(w3467, w3466, w3465) -> (w3464:string)
            }
          }
          n1207 = case shown="\"真\", 默认" w3306 {
            selector: w3306 -> [w3482 _]
            tunnel: w3306 -> [_ w3499]
            tunnel: w3307 -> [_ w3491]
            tunnel: w3308 -> [_ w3488]
            tunnel: [w3482 w3483] -> w3304
            frame "" {
            }
            frame "真", Default {
              # "NH3"
              n1208 = call "规范时间戳.vi"("字符串"=w3488) -> ("result string"=w3487:string)  [unwired: 10 in]
              n1209 = call "核查数据编码整合输出.vi"("字段结束"=FALSE, "数据标识"="N" ("字符串"), "数据类型"="-Check=", "污染物编码"="w21003", "数据值"=w3499) -> ("编码输出"=w3486:string)  [unwired: 6 in]
              n1210 = call "核查数据编码整合输出.vi"("字段结束"=FALSE, "数据类型"="-WaterTime=", "污染物编码"="w21003", "数据值"=w3487) -> ("编码输出"=w3485:string)  [unwired: 7 in]
              n1211 = call "核查数据编码整合输出.vi"("字段结束"=TRUE, "数据类型"="-Water=", "污染物编码"="w21003", "数据值"=w3491) -> ("编码输出"=w3484:string)  [unwired: 7 in]
              n1212 = Concatenate Strings(w3486, w3485, w3484) -> (w3483:string)
            }
          }
          n1213 = case shown="\"真\", 默认" w3315 {
            selector: w3315 -> [w3501 _]
            tunnel: w3315 -> [_ w3518]
            tunnel: w3322 -> [_ w3510]
            tunnel: w3320 -> [_ w3507]
            tunnel: [w3501 w3502] -> w3314
            frame "" {
            }
            frame "真", Default {
              # "CODMn"
              n1214 = call "规范时间戳.vi"("字符串"=w3507) -> ("result string"=w3506:string)  [unwired: 10 in]
              n1215 = call "核查数据编码整合输出.vi"("字段结束"=FALSE, "数据标识"="N" ("字符串"), "数据类型"="-Check=", "污染物编码"="w01019", "数据值"=w3518) -> ("编码输出"=w3505:string)  [unwired: 6 in]
              n1216 = call "核查数据编码整合输出.vi"("字段结束"=FALSE, "数据类型"="-WaterTime=", "污染物编码"="w01019", "数据值"=w3506) -> ("编码输出"=w3504:string)  [unwired: 7 in]
              n1217 = call "核查数据编码整合输出.vi"("字段结束"=TRUE, "数据类型"="-Water=", "污染物编码"="w01019", "数据值"=w3510) -> ("编码输出"=w3503:string)  [unwired: 7 in]
              n1218 = Concatenate Strings(w3505, w3504, w3503) -> (w3502:string)
            }
          }
          n1219 = Empty String/Path?(string/path=w3317) -> (empty?=w3326:bool)
          n1220 = Format Into String(format string="DataTime=%s;%s%s%s%s%s%s%s%s%s%s" ("格式字符串"), w3318, w3314, w3304, w3294, w3284, w3275, w3266, w3254, w3227, w3226, w3225) -> (resulting string=w3328:string)  [unwired: 2 in, 1 out]
          n1221 = case shown="真" w3326 {
            tunnel: [w3522 ""] -> w3327
            tunnel: w3328 -> [w3522 _]
            frame False {
              n1222 = global read "全局 小时数据发送次数.vi" "小时数据发送次数"() -> (w3521:i32)
              n1223 = Increment(x=w3521) -> (x+1=w3520:i32)
              n1224 = global write "全局 小时数据发送次数.vi" "小时数据发送次数"(w3520) -> ()
            }
            frame True {
              n1225 = global read "全局 小时数据发送次数.vi" "小时数据发送次数"() -> (w3524:i32)
              n1226 = Increment(x=w3524) -> (x+1=w3523:i32)
              n1227 = global write "全局 小时数据发送次数.vi" "小时数据发送次数"(w3523) -> ()
            }
          }
        }
        frame "返回执行结果" {
        }
      }
    }
    frame "操作日志" {
      n1228 = global read "全局 小时数据发送次数.vi" "小时数据发送次数"() -> (w3534:i32)
      n1229 = global read "全局 小时数据发送次数.vi" "小时数据发送次数"() -> (w3536:i32)
      n1230 = global read "全局 小时数据发送次数.vi" "小时数据发送次数"() -> (w3532:i32)
      n1231 = global read "全局 小时数据发送次数.vi" "小时数据发送次数"() -> (w3531:i32)
      n1232 = global read "全局 小时数据发送次数.vi" "小时数据发送次数"() -> (w3528:i32)
      n1233 = Index Array(array=w3542, index (row)=w3534) -> (element=w3533:string[])  [unwired: 1 in]
      n1234 = Index Array(array=w3541, index (row)=w3536) -> (element=w3535:string[])  [unwired: 1 in]
      n1235 = Index Array(array=w3539, index (row)=w3532) -> (element=w3530:string[])  [unwired: 1 in]
      n1236 = Index Array(array=w3538, index (row)=w3531) -> (element=w3529:string[])  [unwired: 1 in]
      n1237 = global read "全局1.vi" "枚举"() -> (w3537:enum16{"返回请求应答", "上传数据", "返回执行结果"})
      n1238 = Index Array(array=w3540, index (row)=w3528) -> (element=w3527:string[])  [unwired: 1 in]
      n1239 = case shown="\"返回执行结果\"" w3537 {
        tunnel: ["QnRtn=1" w3549 "ExeRtn=1"] -> w3543
        tunnel: w3535 -> [_ w3570 _]
        tunnel: w3533 -> [_ w3568 _]
        tunnel: w3530 -> [_ w3566 _]
        tunnel: w3529 -> [_ w3565 _]
        tunnel: w3527 -> [_ w3563 _]
        frame "返回请求应答", Default {
          n1240 = global read "全局 数据数组大小.vi" "数据数组大小"() -> (w3546:i32)
          n1241 = Equal To 0?(x=w3546) -> (x = 0?=w3545:bool)
          n1242 = case shown="真" w3545 {
            frame False {
            }
            frame True {
              n1243 = global read "全局 小时数据发送次数.vi" "小时数据发送次数"() -> (w3548:i32)
              n1244 = Increment(x=w3548) -> (x+1=w3547:i32)
              n1245 = global write "全局 小时数据发送次数.vi" "小时数据发送次数"(w3547) -> ()
            }
          }
        }
        frame "上传数据" {
          n1246 = Index Array(array=w3565, index #1=0 ("索引"), index #2=2 ("索引")) -> (element #1=w3564:string, element #2=w3554:string)
          n1247 = Index Array(array=w3570, index #1=0 ("索引"), index #2=2 ("索引")) -> (element #1=w3569:string, element #2=w3556:string)
          n1248 = Index Array(array=w3563, index #1=0 ("索引"), index #2=2 ("索引")) -> (element #1=w3562:string, element #2=w3558:string)
          n1249 = Index Array(array=w3566, index #1=0 ("索引"), index #2=2 ("索引")) -> (element #1=w3571:string, element #2=w3552:string)
          n1250 = Index Array(array=w3568, index #1=0 ("索引"), index #2=2 ("索引")) -> (element #1=w3567:string, element #2=w3561:string)
          n1251 = Empty String/Path?(string/path=w3554) -> (empty?=w3555:bool)
          n1252 = Empty String/Path?(string/path=w3556) -> (empty?=w3557:bool)
          n1253 = Empty String/Path?(string/path=w3552) -> (empty?=w3553:bool)
          n1254 = case shown="假" w3557 {
            tunnel: [w3607 ""] -> w3583
            tunnel: w3556 -> [w3606 _]
            tunnel: w3569 -> [w3605 _]
            frame False {
              # "氨氮"
              n1255 = call "规范时间戳.vi"("字符串"=w3605) -> ("result string"=w3608:string)  [unwired: 10 in]
              n1256 = Format Into String(format string="DataTime=%s;PolId=w21003,i11001-Info=//%s//;" ("格式字符串"), w3608, w3606) -> (resulting string=w3607:string)  [unwired: 2 in, 1 out]
            }
            frame True {
            }
          }
          n1257 = case shown="假" w3555 {
            tunnel: [w3599 ""] -> w3578
            tunnel: w3564 -> [w3601 _]
            tunnel: w3554 -> [w3600 _]
            frame False {
              # "总氮"
              n1258 = call "规范时间戳.vi"("字符串"=w3601) -> ("result string"=w3603:string)  [unwired: 10 in]
              n1259 = Format Into String(format string="DataTime=%s;PolId=w21001,i11001-Info=//%s//;" ("格式字符串"), w3603, w3600) -> (resulting string=w3599:string)  [unwired: 2 in, 1 out]
            }
            frame True {
            }
          }
          n1260 = Empty String/Path?(string/path=w3558) -> (empty?=w3559:bool)
          n1261 = case shown="假" w3553 {
            tunnel: [w3596 ""] -> w3579
            tunnel: w3571 -> [w3594 _]
            tunnel: w3552 -> [w3593 _]
            frame False {
              # "总磷"
              n1262 = call "规范时间戳.vi"("字符串"=w3594) -> ("result string"=w3597:string)  [unwired: 10 in]
              n1263 = Format Into String(format string="DataTime=%s;PolId=w21011,i11001-Info=//%s//;" ("格式字符串"), w3597, w3593) -> (resulting string=w3596:string)  [unwired: 2 in, 1 out]
            }
            frame True {
            }
          }
          n1264 = case shown="假" w3559 {
            tunnel: [w3615 ""] -> w3582
            tunnel: w3562 -> [w3612 _]
            tunnel: w3558 -> [w3611 _]
            frame False {
              # "系统日志"
              n1265 = call "规范时间戳.vi"("字符串"=w3612) -> ("result string"=w3614:string)  [unwired: 10 in]
              n1266 = Format Into String(format string="DataTime=%s;PolId=w00000,i21001-Info=//%s//;" ("格式字符串"), w3614, w3611) -> (resulting string=w3615:string)  [unwired: 2 in, 1 out]
            }
            frame True {
            }
          }
          n1267 = Empty String/Path?(string/path=w3561) -> (empty?=w3560:bool)
          n1268 = case shown="假" w3560 {
            tunnel: [w3619 ""] -> w3584
            tunnel: w3567 -> [w3618 _]
            tunnel: w3561 -> [w3617 _]
            frame False {
              # "高锰酸钾盐"
              n1269 = call "规范时间戳.vi"("字符串"=w3618) -> ("result string"=w3620:string)  [unwired: 10 in]
              n1270 = Format Into String(format string="DataTime=%s;PolId=w01019,i11001-Info=//%s//;" ("格式字符串"), w3620, w3617) -> (resulting string=w3619:string)  [unwired: 2 in, 1 out]
            }
            frame True {
            }
          }
          n1271 = Concatenate Strings(w3584, w3583, w3582, w3579, w3578) -> (w3550:string)
          n1272 = Empty String/Path?(string/path=w3550) -> (empty?=w3551:bool)
          n1273 = case shown="假" w3551 {
            tunnel: [w3589 ""] -> w3549
            tunnel: w3550 -> [w3589 _]
            frame False {
              n1274 = global read "全局 小时数据发送次数.vi" "小时数据发送次数"() -> (w3588:i32)
              n1275 = Increment(x=w3588) -> (x+1=w3587:i32)
              n1276 = global write "全局 小时数据发送次数.vi" "小时数据发送次数"(w3587) -> ()
            }
            frame True {
              n1277 = global read "全局 小时数据发送次数.vi" "小时数据发送次数"() -> (w3591:i32)
              n1278 = Increment(x=w3591) -> (x+1=w3590:i32)
              n1279 = global write "全局 小时数据发送次数.vi" "小时数据发送次数"(w3590) -> ()
            }
          }
        }
        frame "返回执行结果" {
        }
      }
    }
    frame "仪器参数" {
      n1280 = global read "全局 小时数据发送次数.vi" "小时数据发送次数"() -> (w3630:i32)
      n1281 = global read "全局 小时数据发送次数.vi" "小时数据发送次数"() -> (w3632:i32)
      n1282 = global read "全局 小时数据发送次数.vi" "小时数据发送次数"() -> (w3628:i32)
      n1283 = global read "全局 小时数据发送次数.vi" "小时数据发送次数"() -> (w3627:i32)
      n1284 = global read "全局 小时数据发送次数.vi" "小时数据发送次数"() -> (w3624:i32)
      n1285 = Index Array(array=w3638, index (row)=w3630) -> (element=w3629:string[])  [unwired: 1 in]
      n1286 = Index Array(array=w3637, index (row)=w3632) -> (element=w3631:string[])  [unwired: 1 in]
      n1287 = Index Array(array=w3635, index (row)=w3628) -> (element=w3626:string[])  [unwired: 1 in]
      n1288 = Index Array(array=w3634, index (row)=w3627) -> (element=w3625:string[])  [unwired: 1 in]
      n1289 = global read "全局1.vi" "枚举"() -> (w3633:enum16{"返回请求应答", "上传数据", "返回执行结果"})
      n1290 = Index Array(array=w3636, index (row)=w3624) -> ()  [unwired: 1 in, 1 out]
      n1291 = case shown="\"上传数据\"" w3633 {
        tunnel: ["QnRtn=1" w3717 "ExeRtn=1"] -> w3639
        tunnel: w3631 -> [_ w3684 _]
        tunnel: w3629 -> [_ w3712 _]
        tunnel: w3626 -> [_ w3665 _]
        tunnel: w3625 -> [_ w3646 _]
        frame "返回请求应答", Default {
          n1292 = global read "全局 数据数组大小.vi" "数据数组大小"() -> (w3642:i32)
          n1293 = Equal To 0?(x=w3642) -> (x = 0?=w3641:bool)
          n1294 = case shown="真" w3641 {
            frame False {
            }
            frame True {
              n1295 = global read "全局 小时数据发送次数.vi" "小时数据发送次数"() -> (w3644:i32)
              n1296 = Increment(x=w3644) -> (x+1=w3643:i32)
              n1297 = global write "全局 小时数据发送次数.vi" "小时数据发送次数"(w3643) -> ()
            }
          }
        }
        frame "上传数据" {
          n1298 = Index Array(array=w3665, index #1=0 ("索引"), index #2=2 ("索引")) -> (element #1=w3667:string, element #2=w3666:string, element #3=w3679:string, element #4=w3678:string, element #5=w3677:string, element #6=w3676:string, element #7=w3675:string, element #8=w3674:string, element #9=w3673:string, element #10=w3672:string, element #11=w3671:string, element #12=w3670:string, element #13=w3669:string, element #14=w3668:string)  [unwired: 12 in]
          n1299 = Index Array(array=w3646, index #1=0 ("索引"), index #2=2 ("索引")) -> (element #1=w3662:string, element #2=w3663:string, element #3=w3650:string, element #4=w3651:string, element #5=w3652:string, element #6=w3653:string, element #7=w3654:string, element #8=w3655:string, element #9=w3656:string, element #10=w3657:string, element #11=w3658:string, element #12=w3659:string, element #13=w3660:string, element #14=w3661:string)  [unwired: 12 in]
          n1300 = Index Array(array=w3684, index #1=0 ("索引"), index #2=2 ("索引")) -> (element #1=w3700:string, element #2=w3701:string, element #3=w3688:string, element #4=w3689:string, element #5=w3690:string, element #6=w3691:string, element #7=w3692:string, element #8=w3693:string, element #9=w3694:string, element #10=w3695:string, element #11=w3696:string, element #12=w3697:string, element #13=w3698:string, element #14=w3699:string)  [unwired: 12 in]
          n1301 = Index Array(array=w3712, index #1=0 ("索引"), index #2=2 ("索引")) -> (element #1=w3703:string, element #2=w3702:string, element #3=w3716:string, element #4=w3715:string, element #5=w3714:string, element #6=w3713:string, element #7=w3711:string, element #8=w3710:string, element #9=w3709:string, element #10=w3708:string, element #11=w3707:string, element #12=w3706:string, element #13=w3705:string, element #14=w3704:string)  [unwired: 12 in]
          n1302 = Empty String/Path?(string/path=w3666) -> (empty?=w3680:bool)
          n1303 = Empty String/Path?(string/path=w3663) -> (empty?=w3649:bool)
          n1304 = Empty String/Path?(string/path=w3701) -> (empty?=w3687:bool)
          n1305 = Empty String/Path?(string/path=w3702) -> (empty?=w3720:bool)
          n1306 = case shown="假" w3680 {
            tunnel: [w3783 ""] -> w3664
            tunnel: w3667 -> [w3782 _]
            tunnel: w3666 -> [w3776 _]
            tunnel: w3679 -> [w3775 _]
            tunnel: w3678 -> [w3774 _]
            tunnel: w3677 -> [w3773 _]
            tunnel: w3676 -> [w3772 _]
            tunnel: w3675 -> [w3780 _]
            tunnel: w3674 -> [w3771 _]
            tunnel: w3673 -> [w3770 _]
            tunnel: w3672 -> [w3769 _]
            tunnel: w3671 -> [w3768 _]
            tunnel: w3670 -> [w3767 _]
            tunnel: w3669 -> [w3766 _]
            tunnel: w3668 -> [w3779 _]
            frame False {
              # "总磷"
              n1307 = Build Array(w3776, w3775, w3774, w3773, w3772, w3771, w3770, w3769, w3768, w3767, w3766) -> (w3777:string[])
              n1308 = call "规范时间戳.vi"("字符串"=w3782) -> ("result string"=w3784:string)  [unwired: 10 in]
              n1309 = call "字符串精度转换.vi"("数组输入"=w3777) -> ("数组输出"=w3778:string[])  [unwired: 9 in, 1 out]
              n1310 = Index Array(array=w3778) -> (element #1=w3765:string, element #2=w3764:string, element #3=w3763:string, element #4=w3762:string, element #5=w3761:string, element #6=w3760:string, element #7=w3759:string, element #8=w3758:string, element #9=w3757:string, element #10=w3756:string, element #11=w3755:string)  [unwired: 11 in]
              n1311 = Format Into String(format string="DataTime=%s;PolId=w21011,i13001-Info=%s,i13002-Info=%s,i13003-Info=%s,i13004-Info=%s,i13005-Info=%s,i13006-Info=%s,i13007-Info=%s,i13008-Info=%s,i13009-Info=%s,i13010-Info=%s,i13011-Info=%s,i13012-Info=%s,i13013-Info=%s;" ("格式字符串"), w3784, w3765, w3764, w3763, w3762, w3761, w3780, w3760, w3759, w3758, w3757, w3756, w3755, w3779) -> (resulting string=w3783:string)  [unwired: 2 in, 1 out]
            }
            frame True {
            }
          }
          n1312 = case shown="假" w3649 {
            tunnel: [w3752 ""] -> w3645
            tunnel: w3662 -> [w3751 _]
            tunnel: w3663 -> [w3745 _]
            tunnel: w3650 -> [w3744 _]
            tunnel: w3651 -> [w3743 _]
            tunnel: w3652 -> [w3742 _]
            tunnel: w3653 -> [w3741 _]
            tunnel: w3654 -> [w3749 _]
            tunnel: w3655 -> [w3740 _]
            tunnel: w3656 -> [w3739 _]
            tunnel: w3657 -> [w3738 _]
            tunnel: w3658 -> [w3737 _]
            tunnel: w3659 -> [w3736 _]
            tunnel: w3660 -> [w3735 _]
            tunnel: w3661 -> [w3748 _]
            frame False {
              # "总氮"
              n1313 = Build Array(w3745, w3744, w3743, w3742, w3741, w3740, w3739, w3738, w3737, w3736, w3735) -> (w3746:string[])
              n1314 = call "规范时间戳.vi"("字符串"=w3751) -> ("result string"=w3753:string)  [unwired: 10 in]
              n1315 = call "字符串精度转换.vi"("数组输入"=w3746) -> ("数组输出"=w3747:string[])  [unwired: 9 in, 1 out]
              n1316 = Index Array(array=w3747) -> (element #1=w3734:string, element #2=w3733:string, element #3=w3732:string, element #4=w3731:string, element #5=w3730:string, element #6=w3729:string, element #7=w3728:string, element #8=w3727:string, element #9=w3726:string, element #10=w3725:string, element #11=w3724:string)  [unwired: 11 in]
              n1317 = Format Into String(format string="DataTime=%s;PolId=w21001,i13001-Info=%s,i13002-Info=%s,i13003-Info=%s,i13004-Info=%s,i13005-Info=%s,i13006-Info=%s,i13007-Info=%s,i13008-Info=%s,i13009-Info=%s,i13010-Info=%s,i13011-Info=%s,i13012-Info=%s,i13013-Info=%s;" ("格式字符串"), w3753, w3734, w3733, w3732, w3731, w3730, w3749, w3729, w3728, w3727, w3726, w3725, w3724, w3748) -> (resulting string=w3752:string)  [unwired: 2 in, 1 out]
            }
            frame True {
            }
          }
          n1318 = case shown="假" w3687 {
            tunnel: [w3814 ""] -> w3683
            tunnel: w3700 -> [w3813 _]
            tunnel: w3701 -> [w3809 _]
            tunnel: w3688 -> [w3808 _]
            tunnel: w3689 -> [w3807 _]
            tunnel: w3690 -> [w3806 _]
            tunnel: w3691 -> [w3805 _]
            tunnel: w3692 -> [w3798 _]
            tunnel: w3693 -> [w3799 _]
            tunnel: w3694 -> [w3800 _]
            tunnel: w3695 -> [w3801 _]
            tunnel: w3696 -> [w3802 _]
            tunnel: w3697 -> [w3803 _]
            tunnel: w3698 -> [w3804 _]
            tunnel: w3699 -> [w3797 _]
            frame False {
              # "氨氮"
              n1319 = Build Array(w3809, w3808, w3807, w3806, w3805, w3799, w3800, w3801, w3802, w3803, w3804) -> (w3810:string[])
              n1320 = call "规范时间戳.vi"("字符串"=w3813) -> ("result string"=w3815:string)  [unwired: 10 in]
              n1321 = call "字符串精度转换.vi"("数组输入"=w3810) -> ("数组输出"=w3811:string[])  [unwired: 9 in, 1 out]
              n1322 = Index Array(array=w3811) -> (element #1=w3796:string, element #2=w3795:string, element #3=w3794:string, element #4=w3793:string, element #5=w3792:string, element #6=w3791:string, element #7=w3790:string, element #8=w3789:string, element #9=w3788:string, element #10=w3787:string, element #11=w3786:string)  [unwired: 11 in]
              n1323 = Format Into String(format string="DataTime=%s;PolId=w21003,i13001-Info=%s,i13002-Info=%s,i13003-Info=%s,i13004-Info=%s,i13005-Info=%s,i13006-Info=%s,i13007-Info=%s,i13008-Info=%s,i13009-Info=%s,i13010-Info=%s,i13011-Info=%s,i13012-Info=%s,i13013-Info=%s;" ("格式字符串"), w3815, w3796, w3795, w3794, w3793, w3792, w3798, w3791, w3790, w3789, w3788, w3787, w3786, w3797) -> (resulting string=w3814:string)  [unwired: 2 in, 1 out]
            }
            frame True {
            }
          }
          n1324 = case shown="假" w3720 {
            tunnel: [w3851 ""] -> w3722
            tunnel: w3703 -> [w3850 _]
            tunnel: w3702 -> [w3846 _]
            tunnel: w3716 -> [w3845 _]
            tunnel: w3715 -> [w3844 _]
            tunnel: w3714 -> [w3843 _]
            tunnel: w3713 -> [w3842 _]
            tunnel: w3711 -> [w3848 _]
            tunnel: w3710 -> [w3834 _]
            tunnel: w3709 -> [w3833 _]
            tunnel: w3708 -> [w3832 _]
            tunnel: w3707 -> [w3831 _]
            tunnel: w3706 -> [w3830 _]
            tunnel: w3705 -> [w3829 _]
            tunnel: w3704 -> [w3847 _]
            frame False {
              # "高锰酸钾盐"
              n1325 = Build Array(w3846, w3845, w3844, w3843, w3842, w3834, w3833, w3832, w3831, w3830, w3829) -> (w3841:string[])
              n1326 = call "规范时间戳.vi"("字符串"=w3850) -> ("result string"=w3852:string)  [unwired: 10 in]
              n1327 = call "字符串精度转换.vi"("数组输入"=w3841) -> ("数组输出"=w3840:string[])  [unwired: 9 in, 1 out]
              n1328 = Index Array(array=w3840) -> (element #1=w3839:string, element #2=w3838:string, element #3=w3837:string, element #4=w3836:string, element #5=w3835:string, element #6=w3828:string, element #7=w3827:string, element #8=w3826:string, element #9=w3825:string, element #10=w3824:string, element #11=w3823:string)  [unwired: 11 in]
              n1329 = Format Into String(format string="DataTime=%s;PolId=w01019,i13001-Info=%s,i13002-Info=%s,i13003-Info=%s,i13004-Info=%s,i13005-Info=%s,i13006-Info=%s,i13007-Info=%s,i13008-Info=%s,i13009-Info=%s,i13010-Info=%s,i13011-Info=%s,i13012-Info=%s,i13013-Info=%s;" ("格式字符串"), w3852, w3839, w3838, w3837, w3836, w3835, w3848, w3828, w3827, w3826, w3825, w3824, w3823, w3847) -> (resulting string=w3851:string)  [unwired: 2 in, 1 out]
            }
            frame True {
            }
          }
          n1330 = Concatenate Strings(w3722, w3683, w3664, w3645) -> (w3718:string)
          n1331 = Empty String/Path?(string/path=w3718) -> (empty?=w3719:bool)
          n1332 = case shown="假" w3719 {
            tunnel: [w3819 ""] -> w3717
            tunnel: w3718 -> [w3819 _]
            frame False {
              n1333 = global read "全局 小时数据发送次数.vi" "小时数据发送次数"() -> (w3818:i32)
              n1334 = Increment(x=w3818) -> (x+1=w3817:i32)
              n1335 = global write "全局 小时数据发送次数.vi" "小时数据发送次数"(w3817) -> ()
            }
            frame True {
              n1336 = global read "全局 小时数据发送次数.vi" "小时数据发送次数"() -> (w3821:i32)
              n1337 = Increment(x=w3821) -> (x+1=w3820:i32)
              n1338 = global write "全局 小时数据发送次数.vi" "小时数据发送次数"(w3820) -> ()
            }
          }
        }
        frame "返回执行结果" {
        }
      }
    }
    frame "提取仪器参数" {
      n1339 = global read "全局 小时数据发送次数.vi" "小时数据发送次数"() -> (w3864:i32)
      n1340 = global read "全局 小时数据发送次数.vi" "小时数据发送次数"() -> (w3866:i32)
      n1341 = global read "全局 小时数据发送次数.vi" "小时数据发送次数"() -> (w3862:i32)
      n1342 = global read "全局 小时数据发送次数.vi" "小时数据发送次数"() -> (w3857:i32)
      n1343 = global read "全局 小时数据发送次数.vi" "小时数据发送次数"() -> (w3861:i32)
      n1344 = global read "全局 小时数据发送次数.vi" "小时数据发送次数"() -> (w3858:i32)
      n1345 = Index Array(array=w3872, index (row)=w3864) -> (element=w3863:string[])  [unwired: 1 in]
      n1346 = Index Array(array=w3871, index (row)=w3866) -> (element=w3865:string[])  [unwired: 1 in]
      n1347 = Index Array(array=w3869, index (row)=w3862) -> (element=w3860:string[])  [unwired: 1 in]
      n1348 = Index Array(array=w3856, index (row)=w3857) -> (element=w3855:string[])  [unwired: 1 in]
      n1349 = Index Array(array=w3868, index (row)=w3861) -> (element=w3859:string[])  [unwired: 1 in]
      n1350 = global read "全局1.vi" "枚举"() -> (w3867:enum16{"返回请求应答", "上传数据", "返回执行结果"})
      n1351 = Index Array(array=w3870, index (row)=w3858) -> ()  [unwired: 1 in, 1 out]
      n1352 = case shown="\"上传数据\"" w3867 {
        tunnel: ["QnRtn=1" w3916 "ExeRtn=1"] -> w3873
        tunnel: w3865 -> [_ w3908 _]
        tunnel: w3863 -> [_ w3915 _]
        tunnel: w3860 -> [_ w3903 _]
        tunnel: w3859 -> [_ w3898 _]
        tunnel: w3855 -> [_ w3893 _]
        frame "返回请求应答", Default {
          n1353 = global read "全局 数据数组大小.vi" "数据数组大小"() -> (w3876:i32)
          n1354 = Equal To 0?(x=w3876) -> (x = 0?=w3875:bool)
          n1355 = case shown="假" w3875 {
            frame False {
            }
            frame True {
              n1356 = global read "全局 小时数据发送次数.vi" "小时数据发送次数"() -> (w3878:i32)
              n1357 = Increment(x=w3878) -> (x+1=w3877:i32)
              n1358 = global write "全局 小时数据发送次数.vi" "小时数据发送次数"(w3877) -> ()
            }
          }
        }
        frame "上传数据" {
          n1359 = global read "全局 提取仪器参数.vi" "参数编码"() -> (w3884:string)
          n1360 = global read "全局 提取仪器参数.vi" "参数编码"() -> (w3883:string)
          n1361 = global read "全局 提取仪器参数.vi" "参数编码"() -> (w3886:string)
          n1362 = global read "全局 提取仪器参数.vi" "参数编码"() -> (w3888:string)
          n1363 = global read "全局 提取仪器参数.vi" "参数编码"() -> (w3885:string)
          n1364 = case shown="\"i13001\", 默认" w3884 {
            tunnel: [2 ("索引") 3 ("索引") 4 ("索引") 5 ("索引") 6 ("索引") 7 ("索引") 8 ("索引") 9 ("索引") 10 ("索引") 11 ("索引") 12 ("索引") 13 ("索引") 14 ("索引")] -> w3881
            frame "i13001", Default {
            }
            frame "i13002" {
            }
            frame "i13003" {
            }
            frame "i13004" {
            }
            frame "i13005" {
            }
            frame "i13006" {
            }
            frame "i13007" {
            }
            frame "i13008" {
            }
            frame "i13009" {
            }
            frame "i13010" {
            }
            frame "i13011" {
            }
            frame "i13012" {
            }
            frame "i13013" {
            }
          }
          n1365 = Index Array(array=w3903, index #1=0 ("索引"), index #2=w3881) -> (element #1=w3905:string, element #2=w3904:string)
          n1366 = case shown="\"i13001\", 默认" w3883 {
            tunnel: [2 ("索引") 3 ("索引") 4 ("索引") 5 ("索引") 6 ("索引") 7 ("索引") 8 ("索引") 9 ("索引") 10 ("索引") 11 ("索引") 12 ("索引") 13 ("索引") 14 ("索引")] -> w3882
            frame "i13001", Default {
            }
            frame "i13002" {
            }
            frame "i13003" {
            }
            frame "i13004" {
            }
            frame "i13005" {
            }
            frame "i13006" {
            }
            frame "i13007" {
            }
            frame "i13008" {
            }
            frame "i13009" {
            }
            frame "i13010" {
            }
            frame "i13011" {
            }
            frame "i13012" {
            }
            frame "i13013" {
            }
          }
          n1367 = Index Array(array=w3898, index #1=0 ("索引"), index #2=w3882) -> (element #1=w3901:string, element #2=w3902:string)
          n1368 = case shown="\"i13006\"" w3886 {
            tunnel: [2 ("索引") 3 ("索引") 4 ("索引") 5 ("索引") 6 ("索引") 7 ("索引") 8 ("索引") 9 ("索引") 10 ("索引") 11 ("索引") 12 ("索引") 13 ("索引") 14 ("索引")] -> w3879
            frame "i13001", Default {
            }
            frame "i13002" {
            }
            frame "i13003" {
            }
            frame "i13004" {
            }
            frame "i13005" {
            }
            frame "i13006" {
            }
            frame "i13007" {
            }
            frame "i13008" {
            }
            frame "i13009" {
            }
            frame "i13010" {
            }
            frame "i13011" {
            }
            frame "i13012" {
            }
            frame "i13013" {
            }
          }
          n1369 = Index Array(array=w3893, index #1=0 ("索引"), index #2=w3879) -> (element #1=w3895:string, element #2=w3894:string)
          n1370 = case shown="\"i13001\", 默认" w3888 {
            tunnel: [2 ("索引") 3 ("索引") 4 ("索引") 5 ("索引") 6 ("索引") 7 ("索引") 8 ("索引") 9 ("索引") 10 ("索引") 11 ("索引") 12 ("索引") 13 ("索引") 14 ("索引")] -> w3887
            frame "i13001", Default {
            }
            frame "i13002" {
            }
            frame "i13003" {
            }
            frame "i13004" {
            }
            frame "i13005" {
            }
            frame "i13006" {
            }
            frame "i13007" {
            }
            frame "i13008" {
            }
            frame "i13009" {
            }
            frame "i13010" {
            }
            frame "i13011" {
            }
            frame "i13012" {
            }
            frame "i13013" {
            }
          }
          n1371 = Index Array(array=w3915, index #1=0 ("索引"), index #2=w3887) -> (element #1=w3914:string, element #2=w3913:string)
          n1372 = case shown="\"i13001\", 默认" w3885 {
            tunnel: [2 ("索引") 3 ("索引") 4 ("索引") 5 ("索引") 6 ("索引") 7 ("索引") 8 ("索引") 9 ("索引") 10 ("索引") 11 ("索引") 12 ("索引") 13 ("索引") 14 ("索引")] -> w3880
            frame "i13001", Default {
            }
            frame "i13002" {
            }
            frame "i13003" {
            }
            frame "i13004" {
            }
            frame "i13005" {
            }
            frame "i13006" {
            }
            frame "i13007" {
            }
            frame "i13008" {
            }
            frame "i13009" {
            }
            frame "i13010" {
            }
            frame "i13011" {
            }
            frame "i13012" {
            }
            frame "i13013" {
            }
          }
          n1373 = Index Array(array=w3908, index #1=0 ("索引"), index #2=w3880) -> (element #1=w3911:string, element #2=w3912:string)
          n1374 = Empty String/Path?(string/path=w3904) -> (empty?=w3906:bool)
          n1375 = Empty String/Path?(string/path=w3902) -> (empty?=w3900:bool)
          n1376 = Empty String/Path?(string/path=w3894) -> (empty?=w3896:bool)
          n1377 = Empty String/Path?(string/path=w3912) -> (empty?=w3910:bool)
          n1378 = Empty String/Path?(string/path=w3913) -> (empty?=w3919:bool)
          n1379 = case shown="假" w3906 {
            tunnel: [w4022 ""] -> w3890
            tunnel: w3905 -> [w4021 _]
            tunnel: w3904 -> [w4016 _]
            frame False {
              # "总磷"
              n1380 = global read "全局 提取仪器参数.vi" "参数编码"() -> (w4017:string)
              n1381 = call "规范时间戳.vi"("字符串"=w4021) -> ("result string"=w4023:string)  [unwired: 10 in]
              n1382 = case shown="\"假\", 默认" w4017 {
                tunnel: w4016 -> [w4025 w4027]
                tunnel: [w4024 w4026] -> w4015
                frame "假", Default {
                  n1383 = call "字符串精度转换.vi"("输入字符串"=w4025) -> ("输出字符串"=w4024:string)  [unwired: 9 in, 1 out]
                }
                frame "i13006", "i13013" {
                  n1384 = call "规范时间戳.vi"("字符串"=w4027) -> ("result string"=w4026:string)  [unwired: 10 in]
                }
              }
              n1385 = Concatenate Strings("DataTime=%s;PolId=w21011," ("格式字符串"), w4017, "-Info=%s;" ("格式字符串")) -> (w4018:string)
              n1386 = Format Into String(format string=w4018, w4023, w4015) -> (resulting string=w4022:string)  [unwired: 2 in, 1 out]
            }
            frame True {
            }
          }
          n1387 = case shown="假" w3900 {
            tunnel: [w4008 ""] -> w3889
            tunnel: w3901 -> [w4007 _]
            tunnel: w3902 -> [w4002 _]
            frame False {
              # "总氮"
              n1388 = global read "全局 提取仪器参数.vi" "参数编码"() -> (w4003:string)
              n1389 = call "规范时间戳.vi"("字符串"=w4007) -> ("result string"=w4009:string)  [unwired: 10 in]
              n1390 = case shown="\"假\", 默认" w4003 {
                tunnel: w4002 -> [w4011 w4013]
                tunnel: [w4010 w4012] -> w4001
                frame "假", Default {
                  n1391 = call "字符串精度转换.vi"("输入字符串"=w4011) -> ("输出字符串"=w4010:string)  [unwired: 9 in, 1 out]
                }
                frame "i13006", "i13013" {
                  n1392 = call "规范时间戳.vi"("字符串"=w4013) -> ("result string"=w4012:string)  [unwired: 10 in]
                }
              }
              n1393 = Concatenate Strings("DataTime=%s;PolId=w21001," ("格式字符串"), w4003, "-Info=%s;" ("格式字符串")) -> (w4004:string)
              n1394 = Format Into String(format string=w4004, w4009, w4001) -> (resulting string=w4008:string)  [unwired: 2 in, 1 out]
            }
            frame True {
            }
          }
          n1395 = case shown="假" w3896 {
            tunnel: [w3994 ""] -> w3892
            tunnel: w3895 -> [w3993 _]
            tunnel: w3894 -> [w3989 _]
            frame False {
              # "化学需氧量"
              n1396 = global read "全局 提取仪器参数.vi" "参数编码"() -> (w3987:string)
              n1397 = call "规范时间戳.vi"("字符串"=w3993) -> ("result string"=w3995:string)  [unwired: 10 in]
              n1398 = case shown="\"假\", 默认" w3987 {
                tunnel: w3989 -> [w3997 w3999]
                tunnel: [w3996 w3998] -> w3988
                frame "假", Default {
                  n1399 = call "字符串精度转换.vi"("输入字符串"=w3997) -> ("输出字符串"=w3996:string)  [unwired: 9 in, 1 out]
                }
                frame "i13006", "i13013" {
                  n1400 = call "规范时间戳.vi"("字符串"=w3999) -> ("result string"=w3998:string)  [unwired: 10 in]
                }
              }
              n1401 = Concatenate Strings("DataTime=%s;PolId=w01018," ("格式字符串"), w3987, "-Info=%s;" ("格式字符串")) -> (w3990:string)
              n1402 = Format Into String(format string=w3990, w3995, w3988) -> (resulting string=w3994:string)  [unwired: 2 in, 1 out]
            }
            frame True {
            }
          }
          n1403 = case shown="假" w3910 {
            tunnel: [w4036 ""] -> w3891
            tunnel: w3911 -> [w4035 _]
            tunnel: w3912 -> [w4030 _]
            frame False {
              # "氨氮"
              n1404 = global read "全局 提取仪器参数.vi" "参数编码"() -> (w4031:string)
              n1405 = call "规范时间戳.vi"("字符串"=w4035) -> ("result string"=w4037:string)  [unwired: 10 in]
              n1406 = case shown="\"假\", 默认" w4031 {
                tunnel: w4030 -> [w4039 w4041]
                tunnel: [w4038 w4040] -> w4029
                frame "假", Default {
                  n1407 = call "字符串精度转换.vi"("输入字符串"=w4039) -> ("输出字符串"=w4038:string)  [unwired: 9 in, 1 out]
                }
                frame "i13006", "i13013" {
                  n1408 = call "规范时间戳.vi"("字符串"=w4041) -> ("result string"=w4040:string)  [unwired: 10 in]
                }
              }
              n1409 = Concatenate Strings("DataTime=%s;PolId=w21003," ("格式字符串"), w4031, "-Info=%s;" ("格式字符串")) -> (w4032:string)
              n1410 = Format Into String(format string=w4032, w4037, w4029) -> (resulting string=w4036:string)  [unwired: 2 in, 1 out]
            }
            frame True {
            }
          }
          n1411 = case shown="假" w3919 {
            tunnel: [w4056 ""] -> w3920
            tunnel: w3914 -> [w4055 _]
            tunnel: w3913 -> [w4051 _]
            frame False {
              # "高锰酸钾盐"
              n1412 = global read "全局 提取仪器参数.vi" "参数编码"() -> (w4049:string)
              n1413 = call "规范时间戳.vi"("字符串"=w4055) -> ("result string"=w4057:string)  [unwired: 10 in]
              n1414 = case shown="\"假\", 默认" w4049 {
                tunnel: w4051 -> [w4059 w4061]
                tunnel: [w4058 w4060] -> w4050
                frame "假", Default {
                  n1415 = call "字符串精度转换.vi"("输入字符串"=w4059) -> ("输出字符串"=w4058:string)  [unwired: 9 in, 1 out]
                }
                frame "i13006", "i13013" {
                  n1416 = call "规范时间戳.vi"("字符串"=w4061) -> ("result string"=w4060:string)  [unwired: 10 in]
                }
              }
              n1417 = Concatenate Strings("DataTime=%s;PolId=w01019," ("格式字符串"), w4049, "-Info=%s;" ("格式字符串")) -> (w4052:string)
              n1418 = Format Into String(format string=w4052, w4057, w4050) -> (resulting string=w4056:string)  [unwired: 2 in, 1 out]
            }
            frame True {
            }
          }
          n1419 = Concatenate Strings(w3920, w3892, w3891, w3890, w3889) -> (w3917:string)
          n1420 = Empty String/Path?(string/path=w3917) -> (empty?=w3918:bool)
          n1421 = case shown="假" w3918 {
            tunnel: [w4045 ""] -> w3916
            tunnel: w3917 -> [w4045 _]
            frame False {
              n1422 = global read "全局 小时数据发送次数.vi" "小时数据发送次数"() -> (w4044:i32)
              n1423 = Increment(x=w4044) -> (x+1=w4043:i32)
              n1424 = global write "全局 小时数据发送次数.vi" "小时数据发送次数"(w4043) -> ()
            }
            frame True {
              n1425 = global read "全局 小时数据发送次数.vi" "小时数据发送次数"() -> (w4047:i32)
              n1426 = Increment(x=w4047) -> (x+1=w4046:i32)
              n1427 = global write "全局 小时数据发送次数.vi" "小时数据发送次数"(w4046) -> ()
            }
          }
        }
        frame "返回执行结果" {
        }
      }
    }
    frame "报警信息" {
      n1428 = global read "全局 小时数据发送次数.vi" "小时数据发送次数"() -> (w4071:i32)
      n1429 = global read "全局 小时数据发送次数.vi" "小时数据发送次数"() -> (w4073:i32)
      n1430 = global read "全局 小时数据发送次数.vi" "小时数据发送次数"() -> (w4069:i32)
      n1431 = global read "全局 小时数据发送次数.vi" "小时数据发送次数"() -> (w4068:i32)
      n1432 = global read "全局 小时数据发送次数.vi" "小时数据发送次数"() -> (w4065:i32)
      n1433 = Index Array(array=w4079, index (row)=w4071) -> (element=w4070:string[])  [unwired: 1 in]
      n1434 = Index Array(array=w4078, index (row)=w4073) -> (element=w4072:string[])  [unwired: 1 in]
      n1435 = Index Array(array=w4076, index (row)=w4069) -> (element=w4067:string[])  [unwired: 1 in]
      n1436 = Index Array(array=w4075, index (row)=w4068) -> (element=w4066:string[])  [unwired: 1 in]
      n1437 = global read "全局1.vi" "枚举"() -> (w4074:enum16{"返回请求应答", "上传数据", "返回执行结果"})
      n1438 = Index Array(array=w4077, index (row)=w4065) -> (element=w4064:string[])  [unwired: 1 in]
      n1439 = case shown="\"上传数据\"" w4074 {
        tunnel: ["QnRtn=1" w4086 "ExeRtn=1"] -> w4080
        tunnel: w4072 -> [_ w4107 _]
        tunnel: w4070 -> [_ w4105 _]
        tunnel: w4067 -> [_ w4103 _]
        tunnel: w4066 -> [_ w4102 _]
        tunnel: w4064 -> [_ w4100 _]
        frame "返回请求应答", Default {
          n1440 = global read "全局 数据数组大小.vi" "数据数组大小"() -> (w4083:i32)
          n1441 = Equal To 0?(x=w4083) -> (x = 0?=w4082:bool)
          n1442 = case shown="真" w4082 {
            frame False {
            }
            frame True {
              n1443 = global read "全局 小时数据发送次数.vi" "小时数据发送次数"() -> (w4085:i32)
              n1444 = Increment(x=w4085) -> (x+1=w4084:i32)
              n1445 = global write "全局 小时数据发送次数.vi" "小时数据发送次数"(w4084) -> ()
            }
          }
        }
        frame "上传数据" {
          n1446 = global read "全局 小时数据发送次数.vi" "小时数据发送次数"() -> (w4115:i32)
          n1447 = Increment(x=w4115) -> (x+1=w4114:i32)
          n1448 = global write "全局 小时数据发送次数.vi" "小时数据发送次数"(w4114) -> ()
          n1449 = Index Array(array=w4102, index #1=0 ("索引"), index #2=2 ("索引")) -> (element #1=w4101:string, element #2=w4091:string)
          n1450 = Index Array(array=w4107, index #1=0 ("索引"), index #2=2 ("索引")) -> (element #1=w4106:string, element #2=w4093:string)
          n1451 = Empty String/Path?(string/path=w4093) -> (empty?=w4094:bool)
          n1452 = Index Array(array=w4100, index #1=0 ("索引"), index #2=2 ("索引")) -> (element #1=w4099:string, element #2=w4095:string)
          n1453 = Index Array(array=w4103, index #1=0 ("索引"), index #2=2 ("索引")) -> (element #1=w4108:string, element #2=w4089:string)
          n1454 = Index Array(array=w4105, index #1=0 ("索引"), index #2=2 ("索引")) -> (element #1=w4104:string, element #2=w4098:string)
          n1455 = Empty String/Path?(string/path=w4091) -> (empty?=w4092:bool)
          n1456 = case shown="假" w4094 {
            tunnel: [w4146 ""] -> w4122
            tunnel: w4093 -> [_ _]
            tunnel: w4106 -> [w4145 _]
            frame False {
              w4144 = "0" ("输入 2")
              # "氨氮"
              n1457 = call "规范时间戳.vi"("字符串"=w4145) -> ("result string"=w4147:string)  [unwired: 10 in]
              n1458 = Format Into String(format string="DataTime=%s;PolId=w21003,i12001-Info=%s,i12031-Info=%s;" ("格式字符串"), w4147, w4144, w4144) -> (resulting string=w4146:string)  [unwired: 2 in, 1 out]
            }
            frame True {
            }
          }
          n1459 = Empty String/Path?(string/path=w4095) -> (empty?=w4096:bool)
          n1460 = Empty String/Path?(string/path=w4098) -> (empty?=w4097:bool)
          n1461 = Empty String/Path?(string/path=w4089) -> (empty?=w4090:bool)
          n1462 = case shown="假" w4096 {
            tunnel: [w4154 ""] -> w4121
            tunnel: w4099 -> [w4151 _]
            tunnel: w4095 -> [_ _]
            frame False {
              w4150 = "0" ("输入 2")
              # "系统日志"
              n1463 = call "规范时间戳.vi"("字符串"=w4151) -> ("result string"=w4153:string)  [unwired: 10 in]
              n1464 = Format Into String(format string="DataTime=%s;PolId=w00000,i22001-Info=%s,i22003-Info=%s;" ("格式字符串"), w4153, w4150, w4150) -> (resulting string=w4154:string)  [unwired: 2 in, 1 out]
            }
            frame True {
            }
          }
          n1465 = case shown="假" w4092 {
            tunnel: [w4139 ""] -> w4117
            tunnel: w4101 -> [w4140 _]
            tunnel: w4091 -> [_ _]
            frame False {
              w4138 = "0" ("输入 2")
              # "总氮"
              n1466 = call "规范时间戳.vi"("字符串"=w4140) -> ("result string"=w4142:string)  [unwired: 10 in]
              n1467 = Format Into String(format string="DataTime=%s;PolId=w21001,i12001-Info=%s,i12031-Info=%s;" ("格式字符串"), w4142, w4138, w4138) -> (resulting string=w4139:string)  [unwired: 2 in, 1 out]
            }
            frame True {
            }
          }
          n1468 = case shown="假" w4090 {
            tunnel: [w4136 ""] -> w4118
            tunnel: w4108 -> [w4134 _]
            tunnel: w4089 -> [_ _]
            frame False {
              w4132 = "0" ("输入 2")
              # "总磷"
              n1469 = call "规范时间戳.vi"("字符串"=w4134) -> ("result string"=w4133:string)  [unwired: 10 in]
              n1470 = Format Into String(format string="DataTime=%s;PolId=w21011,i12001-Info=%s,i12031-Info=%s;" ("格式字符串"), w4133, w4132, w4132) -> (resulting string=w4136:string)  [unwired: 2 in, 1 out]
            }
            frame True {
            }
          }
          n1471 = case shown="假" w4097 {
            tunnel: [w4159 ""] -> w4123
            tunnel: w4104 -> [w4158 _]
            tunnel: w4098 -> [_ _]
            frame False {
              # "高锰酸钾盐"
              n1472 = call "规范时间戳.vi"("字符串"=w4158) -> ("result string"=w4160:string)  [unwired: 10 in]
              n1473 = Format Into String(format string="DataTime=%s;PolId=w01019,i12001-Info=%s,i12031-Info=%s;" ("格式字符串"), w4160, "0" ("输入 2"), "0" ("输入 3")) -> (resulting string=w4159:string)  [unwired: 2 in, 1 out]
            }
            frame True {
            }
          }
          n1474 = Concatenate Strings(w4123, w4122, w4121, w4118, w4117) -> (w4087:string)
          n1475 = Empty String/Path?(string/path=w4087) -> (empty?=w4088:bool)
          n1476 = case shown="假" w4088 {
            tunnel: [w4128 ""] -> w4086
            tunnel: w4087 -> [w4128 _]
            frame False {
              n1477 = global read "全局 小时数据发送次数.vi" "小时数据发送次数"() -> (w4127:i32)
              n1478 = Increment(x=w4127) -> (x+1=w4126:i32)
              n1479 = global write "全局 小时数据发送次数.vi" "小时数据发送次数"(w4126) -> ()
            }
            frame True {
              n1480 = global read "全局 小时数据发送次数.vi" "小时数据发送次数"() -> (w4130:i32)
              n1481 = Increment(x=w4130) -> (x+1=w4129:i32)
              n1482 = global write "全局 小时数据发送次数.vi" "小时数据发送次数"(w4129) -> ()
            }
          }
        }
        frame "返回执行结果" {
        }
      }
    }
    frame "系统状态" {
      # "DataTime=20100301145000;PolId=w01018,i12001-Info=1,i12003-Info=0"
      # "100  当前模式\n101  CODMn状态  （0待机，1运行）\n102  氨氮状态\n103  总磷状态\n104  总氮状态\n105  CODCr状态\n106  运行周期"
      n1483 = global read "全局1.vi" "register values"() -> (w4189:u16[])
      n1484 = Index Array(array=w4189, index #1=1 ("索引")) -> (element #1=w4184:u16, element #2=w4180:u16, element #3=w4174:u16, element #4=w4173:u16, element #5=w4169:u16)  [unwired: 4 in]
      n1485 = Number To Decimal String(number=w4184) -> (decimal integer string=w4183:string)  [unwired: 1 in]
      n1486 = Number To Decimal String(number=w4169) -> (decimal integer string=w4171:string)  [unwired: 1 in]
      n1487 = Number To Decimal String(number=w4174) -> (decimal integer string=w4175:string)  [unwired: 1 in]
      n1488 = Number To Decimal String(number=w4180) -> (decimal integer string=w4179:string)  [unwired: 1 in]
      n1489 = Number To Decimal String(number=w4173) -> (decimal integer string=w4172:string)  [unwired: 1 in]
      n1490 = Format Into String(format string="PolId=w01019,i12001-Info=%s;" ("格式字符串"), w4183) -> (resulting string=w4182:string)  [unwired: 2 in, 1 out]
      n1491 = Format Into String(format string="PolId=w01018,i12001-Info=%s;" ("格式字符串"), w4171) -> (resulting string=w4166:string)  [unwired: 2 in, 1 out]
      n1492 = Format Into String(format string="PolId=w21003,i12001-Info=%s;" ("格式字符串"), w4179) -> (resulting string=w4178:string)  [unwired: 2 in, 1 out]
      n1493 = Format Into String(format string="PolId=w21011,i12001-Info=%s;" ("格式字符串"), w4175) -> (resulting string=w4168:string)  [unwired: 2 in, 1 out]
      n1494 = Format Into String(format string="PolId=w21001,i12001-Info=%s;" ("格式字符串"), w4172) -> (resulting string=w4167:string)  [unwired: 2 in, 1 out]
      n1495 = Get Date/Time In Seconds() -> (seconds since 1Jan1904=w4187:timestamp)
      n1496 = Format Date/Time String(time format string (%c)="%Y%m%d%H%M%S" ("时间格式字符串(%c)"), seconds (now)=w4187) -> (date/time string=w4164:string)  [unwired: 1 in]
      n1497 = Format Into String(format string="DataTime=%s;%s%s%s%s%s" ("格式字符串"), w4164, w4182, w4178, w4168, w4167, w4166) -> (resulting string=w4186:string)  [unwired: 2 in, 1 out]
    }
    frame "运行模式" {
      # "DataTime=20100301145000;PolId=w01018,i12001-Info=1,i12003-Info=0"
      # "100  当前模式\n101  CODMn状态  （0待机，1运行）\n102  氨氮状态\n103  总磷状态\n104  总氮状态\n105  CODCr状态\n106  运行周期"
      n1498 = global read "全局1.vi" "register values"() -> (w4200:u16[])
      n1499 = Index Array(array=w4200, index=0 ("索引")) -> (element=w4192:u16)
      n1500 = Number To Decimal String(number=w4192) -> (decimal integer string=w4194:string)  [unwired: 1 in]
      n1501 = Format Into String(format string="RunMode=%s;" ("格式字符串"), w4194) -> (resulting string=w4191:string)  [unwired: 2 in, 1 out]
      n1502 = Get Date/Time In Seconds() -> (seconds since 1Jan1904=w4198:timestamp)
      n1503 = Format Date/Time String(time format string (%c)="%Y%m%d%H%M%S" ("时间格式字符串(%c)"), seconds (now)=w4198) -> (date/time string=w4195:string)  [unwired: 1 in]
      n1504 = Format Into String(format string="DataTime=%s;%s" ("格式字符串"), w4195, w4191) -> (resulting string=w4197:string)  [unwired: 2 in, 1 out]
    }
    frame "测量周期" {
      # "DataTime=20100301145000;PolId=w01018,i12001-Info=1,i12003-Info=0"
      # "100  当前模式\n101  CODMn状态  （0待机，1运行）\n102  氨氮状态\n103  总磷状态\n104  总氮状态\n105  CODCr状态\n106  运行周期"
      n1505 = global read "全局1.vi" "register values"() -> (w4211:u16[])
      n1506 = Index Array(array=w4211, index=6 ("索引")) -> (element=w4203:u16)
      n1507 = Number To Decimal String(number=w4203) -> (decimal integer string=w4204:string)  [unwired: 1 in]
      n1508 = Format Into String(format string="RunInterval=%s;" ("格式字符串"), w4204) -> (resulting string=w4202:string)  [unwired: 2 in, 1 out]
      n1509 = Get Date/Time In Seconds() -> (seconds since 1Jan1904=w4209:timestamp)
      n1510 = Format Date/Time String(time format string (%c)="%Y%m%d%H%M%S" ("时间格式字符串(%c)"), seconds (now)=w4209) -> (date/time string=w4206:string)  [unwired: 1 in]
      n1511 = Format Into String(format string="DataTime=%s;%s" ("格式字符串"), w4206, w4202) -> (resulting string=w4208:string)  [unwired: 2 in, 1 out]
    }
    frame "超标留样" {
      # "DataTime=20100301145000;PolId=w01018,i12001-Info=1,i12003-Info=0"
      # "100  当前模式\n101  CODMn状态  （0待机，1运行）\n102  氨氮状态\n103  总磷状态\n104  总氮状态\n105  CODCr状态\n106  运行周期"
      n1512 = global read "全局1.vi" "register values"() -> (w4222:u16[])
      n1513 = Index Array(array=w4222, index=7 ("索引")) -> (element=w4214:u16)
      n1514 = Number To Decimal String(number=w4214) -> (decimal integer string=w4215:string)  [unwired: 1 in]
      n1515 = Format Into String(format string="VaseNo=%s;" ("格式字符串"), w4215) -> (resulting string=w4213:string)  [unwired: 2 in, 1 out]
      n1516 = Get Date/Time In Seconds() -> (seconds since 1Jan1904=w4220:timestamp)
      n1517 = Format Date/Time String(time format string (%c)="%Y%m%d%H%M%S" ("时间格式字符串(%c)"), seconds (now)=w4220) -> (date/time string=w4217:string)  [unwired: 1 in]
      n1518 = Format Into String(format string="DataTime=%s;%s" ("格式字符串"), w4217, w4213) -> (resulting string=w4219:string)  [unwired: 2 in, 1 out]
    }
  }
  n1519 = Equal?(x="table输入", y="反控命令") -> (x = y?=w35:bool)
  n1520 = case shown="假" w35 {
    tunnel: [w4225 w4229] -> w37
    frame False {
      n1521 = global read "全局1.vi" "枚举"() -> (w4224:enum16{"返回请求应答", "上传数据", "返回执行结果"})
      n1522 = case shown="\"上传数据\"" w4224 {
        tunnel: ["91" ("CN") w4227 "91" ("CN")] -> w4225
        frame "返回请求应答", Default {
        }
        frame "上传数据" {
          n1523 = global read "全局1.vi" "系统编码ST"() -> (w4227:string)
        }
        frame "返回执行结果" {
        }
      }
    }
    frame True {
      n1524 = global read "全局 反控命令枚举.vi" "反控命令枚举"() -> (w4230:enum16{"返回请求应答", "返回执行结果"})
      n1525 = case shown="\"返回执行结果\"" w4230 {
        tunnel: ["91" "91"] -> w4229
        frame "返回请求应答", Default {
        }
        frame "返回执行结果" {
        }
      }
    }
  }
  n1526 = case shown="\"心跳包\", 默认" "table输入" {
    tunnel: ["9015" ("ST") w4243 w4251 w4259 w4266 w4273 w4281 w4289 w4302 w4317 w4326 w4335 w4352 w4360 w4368 w4376 w4384 w4392 w4399 "3020" ("ST") "3042" ("ST") "3056" ("ST") "3015" ("ST")] -> w41
    tunnel: ["9" ("ST") "8" ("ST") "8" ("ST") "8" ("ST") "8" ("ST") "8" ("ST") "8" ("ST") "8" ("ST") "9" ("ST") "9" ("ST") w4329 "8" ("ST") "8" ("ST") "8" ("ST") "8" ("ST") "8" ("ST") "8" ("ST") "8" ("ST") "8" ("ST") "9" ("ST") "9" ("ST") "9" ("ST") "9" ("ST")] -> w40
    tunnel: w26 -> [_ w4241 w4249 w4260 w4267 w4274 w4282 w4290 w4303 w4319 w4328 w4338 w4354 w4362 w4370 w4378 w4386 w4394 w4401 w4407 w4411 w4415 w4419]
    tunnel: [_ w4241 w4249 w4260 w4267 w4274 w4282 w4290 w4303 w4319 w4328 w4338 w4354 w4362 w4370 w4378 w4386 w4394 w4401 w4407 w4411 w4415 w4419] -> w39
    tunnel: [w4233 w4240 w4248 w4256 w4264 w4271 w4279 w4287 w4295 w4316 w4325 w4337 w4350 w4358 w4366 w4374 w4382 w4390 w4398 w4406 w4410 w4414 w4418] -> w27
    frame "心跳包", Default {
      # "心跳包"
      n1527 = Get Date/Time In Seconds() -> (seconds since 1Jan1904=w4236:timestamp)
      n1528 = Format Date/Time String(time format string (%c)="%Y%m%d%H%M%S%3u" ("时间格式字符串(%c)"), seconds (now)=w4236) -> (date/time string=w4235:string)  [unwired: 1 in]
      n1529 = Search and Replace String(input string=w4235, search string="." ("搜索字符串")) -> (result string=w4233:string)  [unwired: 6 in, 3 out]
    }
    frame "提取数采仪时间" {
      n1530 = global read "全局1.vi" "枚举"() -> (w4244:enum16{"返回请求应答", "上传数据", "返回执行结果"})
      n1531 = case shown="\"返回执行结果\"" w4244 {
        tunnel: ["9011" ("CN") "1014" ("CN") "9012" ("CN")] -> w4243
        frame "返回请求应答", Default {
        }
        frame "上传数据" {
        }
        frame "返回执行结果" {
        }
      }
      n1532 = local read "QN"() -> (w4240:string)
    }
    frame "提取实时数据间隔" {
      n1533 = global read "全局1.vi" "枚举"() -> (w4252:enum16{"返回请求应答", "上传数据", "返回执行结果"})
      n1534 = case shown="\"上传数据\"" w4252 {
        tunnel: ["9011" ("CN") "1061" ("CN") "9012" ("CN")] -> w4251
        frame "返回请求应答", Default {
        }
        frame "上传数据" {
        }
        frame "返回执行结果" {
        }
      }
      n1535 = local read "QN"() -> (w4248:string)
    }
    frame "反控命令" {
      n1536 = global read "全局 反控命令枚举.vi" "反控命令枚举"() -> (w4257:enum16{"返回请求应答", "返回执行结果"})
      n1537 = case shown="\"返回请求应答\", 默认" w4257 {
        tunnel: ["9011" ("CN") "9012" ("CN")] -> w4259
        frame "返回请求应答", Default {
        }
        frame "返回执行结果" {
        }
      }
      n1538 = local read "QN"() -> (w4256:string)
    }
    frame "超标留样返回" {
      n1539 = global read "全局1.vi" "枚举"() -> (w4263:enum16{"返回请求应答", "上传数据", "返回执行结果"})
      n1540 = case shown="\"上传数据\"" w4263 {
        tunnel: ["9011" ("CN") "3015" ("CN") "9012" ("CN")] -> w4266
        frame "返回请求应答", Default {
        }
        frame "上传数据" {
        }
        frame "返回执行结果" {
        }
      }
      n1541 = local read "QN"() -> (w4264:string)
    }
    frame "提取经纬度环境信息" {
      n1542 = global read "全局1.vi" "枚举"() -> (w4275:enum16{"返回请求应答", "上传数据", "返回执行结果"})
      n1543 = case shown="\"上传数据\"" w4275 {
        tunnel: ["9011" ("CN") "3041" ("CN") "9012" ("CN")] -> w4273
        frame "返回请求应答", Default {
        }
        frame "上传数据" {
        }
        frame "返回执行结果" {
        }
      }
      n1544 = local read "QN"() -> (w4271:string)
    }
    frame "提取现场系统信息" {
      n1545 = global read "全局1.vi" "枚举"() -> (w4283:enum16{"返回请求应答", "上传数据", "返回执行结果"})
      n1546 = case shown="\"上传数据\"" w4283 {
        tunnel: ["9011" ("CN") "3040" ("CN") "9012" ("CN")] -> w4281
        frame "返回请求应答", Default {
        }
        frame "上传数据" {
        }
        frame "返回执行结果" {
        }
      }
      n1547 = local read "QN"() -> (w4279:string)
    }
    frame "提取监测仪表时间" {
      n1548 = global read "全局1.vi" "枚举"() -> (w4291:enum16{"返回请求应答", "上传数据", "返回执行结果"})
      n1549 = case shown="\"返回执行结果\"" w4291 {
        tunnel: ["9011" ("CN") "1011" ("CN") "9012" ("CN")] -> w4289
        frame "返回请求应答", Default {
        }
        frame "上传数据" {
        }
        frame "返回执行结果" {
        }
      }
      n1550 = local read "QN"() -> (w4287:string)
    }
    frame "实时数据" {
      n1551 = global read "全局1.vi" "枚举"() -> (w4301:enum16{"返回请求应答", "上传数据", "返回执行结果"})
      n1552 = case shown="\"上传数据\"" w4301 {
        tunnel: ["9011" ("CN") w4306 "9012" ("CN")] -> w4302
        frame "返回请求应答", Default {
        }
        frame "上传数据" {
          n1553 = global read "全局 实时数据参数.vi" "实时数据参数"() -> (w4305:string)
          n1554 = case shown="\"平行样测试\"" w4305 {
            tunnel: ["2011" ("CN") "2064" ("CN") "2082" ("CN") "2063" ("CN") "2062" ("CN") "2065" ("CN") "2066" ("CN") "fff" ("CN")] -> w4306
            frame "水样测试", Default {
            }
            frame "平行样测试" {
            }
            frame "集成干预测试" {
            }
            frame "加标回收测试" {
            }
            frame "核查数据" {
            }
            frame "空白测试" {
            }
            frame "跨度核查" {
            }
            frame "" {
            }
          }
        }
        frame "返回执行结果" {
        }
      }
      n1555 = Get Date/Time In Seconds() -> (seconds since 1Jan1904=w4298:timestamp)
      n1556 = Format Date/Time String(time format string (%c)="%Y%m%d%H%M%S%3u" ("时间格式字符串(%c)"), seconds (now)=w4298) -> (date/time string=w4297:string)  [unwired: 1 in]
      n1557 = Search and Replace String(input string=w4297, search string="." ("搜索字符串")) -> (result string=w4295:string)  [unwired: 6 in, 3 out]
    }
    frame "小时数据" {
      # "监测小时数据"
      n1558 = global read "全局1.vi" "枚举"() -> (w4318:enum16{"返回请求应答", "上传数据", "返回执行结果"})
      n1559 = case shown="\"返回请求应答\", 默认" w4318 {
        tunnel: ["9011" ("CN") "2061" ("CN") "9012" ("CN")] -> w4317
        frame "返回请求应答", Default {
        }
        frame "上传数据" {
        }
        frame "返回执行结果" {
        }
      }
      n1560 = local read "QN"() -> (w4316:string)
    }
    frame "提取小时数据" {
      # "监测小时数据"
      n1561 = global read "断电保存全局.vi" "数据组合发送"() -> (w4324:bool)
      n1562 = global read "全局1.vi" "枚举"() -> (w4327:enum16{"返回请求应答", "上传数据", "返回执行结果"})
      n1563 = case shown="\"上传数据\"" w4327 {
        tunnel: ["9011" ("CN") "2061" ("CN") "9012" ("CN")] -> w4326
        frame "返回请求应答", Default {
        }
        frame "上传数据" {
        }
        frame "返回执行结果" {
        }
      }
      n1564 = case shown="真" w4324 {
        tunnel: ["8" ("ST") "9" ("ST")] -> w4329
        frame False {
        }
        frame True {
        }
      }
      n1565 = local read "QN"() -> (w4325:string)
    }
    frame "提取实时数据" {
      # "提取实时数据"
      n1566 = global read "全局1.vi" "枚举"() -> (w4336:enum16{"返回请求应答", "上传数据", "返回执行结果"})
      n1567 = case shown="\"上传数据\"" w4336 {
        tunnel: ["9011" ("CN") w4342 "9012" ("CN")] -> w4335
        frame "返回请求应答", Default {
        }
        frame "上传数据" {
          n1568 = global read "全局 实时数据参数.vi" "实时数据参数"() -> (w4341:string)
          n1569 = case shown="\"平行样测试\"" w4341 {
            tunnel: ["2011" ("CN") "2064" ("CN") "2063" ("CN") "2065" ("CN") "2066" ("CN") "fff" ("CN")] -> w4342
            frame "水样测试", Default {
            }
            frame "平行样测试" {
            }
            frame "加标回收测试" {
            }
            frame "空白测试" {
            }
            frame "跨度核查" {
            }
            frame "" {
            }
          }
        }
        frame "返回执行结果" {
        }
      }
      n1570 = local read "QN"() -> (w4337:string)
    }
    frame "跨度核查" {
      # "跨度核查"
      n1571 = global read "全局1.vi" "枚举"() -> (w4353:enum16{"返回请求应答", "上传数据", "返回执行结果"})
      n1572 = case shown="\"上传数据\"" w4353 {
        tunnel: ["9011" ("CN") "2066" ("ST") "9012" ("CN")] -> w4352
        frame "返回请求应答", Default {
        }
        frame "上传数据" {
        }
        frame "返回执行结果" {
        }
      }
      n1573 = local read "QN"() -> (w4350:string)
    }
    frame "提取加标回收" {
      # "提取加标回收"
      n1574 = global read "全局1.vi" "枚举"() -> (w4361:enum16{"返回请求应答", "上传数据", "返回执行结果"})
      n1575 = case shown="\"上传数据\"" w4361 {
        tunnel: ["9011" ("CN") "2063" ("ST") "9012" ("CN")] -> w4360
        frame "返回请求应答", Default {
        }
        frame "上传数据" {
        }
        frame "返回执行结果" {
        }
      }
      n1576 = local read "QN"() -> (w4358:string)
    }
    frame "提取平行样" {
      # "提取平行样"
      n1577 = global read "全局1.vi" "枚举"() -> (w4369:enum16{"返回请求应答", "上传数据", "返回执行结果"})
      n1578 = case shown="\"上传数据\"" w4369 {
        tunnel: ["9011" ("CN") "2064" ("ST") "9012" ("CN")] -> w4368
        frame "返回请求应答", Default {
        }
        frame "上传数据" {
        }
        frame "返回执行结果" {
        }
      }
      n1579 = local read "QN"() -> (w4366:string)
    }
    frame "空白测试", "零点核查" {
      # "零点核查"
      n1580 = global read "全局1.vi" "枚举"() -> (w4377:enum16{"返回请求应答", "上传数据", "返回执行结果"})
      n1581 = case shown="\"上传数据\"" w4377 {
        tunnel: ["9011" ("CN") "2065" ("ST") "9012" ("CN")] -> w4376
        frame "返回请求应答", Default {
        }
        frame "上传数据" {
        }
        frame "返回执行结果" {
        }
      }
      n1582 = local read "QN"() -> (w4374:string)
    }
    frame "核查数据" {
      # "核查数据"
      n1583 = global read "全局1.vi" "枚举"() -> (w4385:enum16{"返回请求应答", "上传数据", "返回执行结果"})
      n1584 = case shown="\"上传数据\"" w4385 {
        tunnel: ["9011" ("CN") "2062" ("ST") "9012" ("CN")] -> w4384
        frame "返回请求应答", Default {
        }
        frame "上传数据" {
        }
        frame "返回执行结果" {
        }
      }
      n1585 = local read "QN"() -> (w4382:string)
    }
    frame "提取集成干预" {
      # "核查数据"
      n1586 = global read "全局1.vi" "枚举"() -> (w4393:enum16{"返回请求应答", "上传数据", "返回执行结果"})
      n1587 = case shown="\"上传数据\"" w4393 {
        tunnel: ["9011" ("CN") "2082" ("ST") "9012" ("CN")] -> w4392
        frame "返回请求应答", Default {
        }
        frame "上传数据" {
        }
        frame "返回执行结果" {
        }
      }
      n1588 = local read "QN"() -> (w4390:string)
    }
    frame "报警信息", "操作日志", "提取仪器参数", "仪器参数" {
      n1589 = global read "全局1.vi" "枚举"() -> (w4400:enum16{"返回请求应答", "上传数据", "返回执行结果"})
      n1590 = case shown="\"上传数据\"" w4400 {
        tunnel: ["9011" ("CN") "3020" ("CN") "9012" ("CN")] -> w4399
        frame "返回请求应答", Default {
        }
        frame "上传数据" {
        }
        frame "返回执行结果" {
        }
      }
      n1591 = local read "QN"() -> (w4398:string)
    }
    frame "系统状态" {
      n1592 = local read "QN"() -> (w4406:string)
    }
    frame "运行模式" {
      n1593 = local read "QN"() -> (w4410:string)
    }
    frame "测量周期" {
      n1594 = local read "QN"() -> (w4414:string)
    }
    frame "超标留样" {
      n1595 = local read "QN"() -> (w4418:string)
    }
  }
  n1596 = Bundle By Name(cluster="数据块", "ST"=w37, "CN"=w41, "FLAG"=w40, "CP"=w39, "QN"=w27, "MN"="MN", "PW"="PW", "PNUM"=w31, "PNO"=w31) -> (w38:T1)
  n1597 = case shown="\"假\", 默认" "table输入" {
    tunnel: [FALSE w4423] -> w15
    frame "假", Default {
    }
    frame "提取经纬度环境信息", "提取现场系统信息" {
      n1598 = global read "全局1.vi" "枚举"() -> (w4425:enum16{"返回请求应答", "上传数据", "返回执行结果"})
      n1599 = Equal?(x=w4425, y=enum16{"返回请求应答", "上传数据", "返回执行结果"}."上传数据" ("枚举")) -> (x = y?=w4423:bool)
    }
  }
  n1600 = call "HJ212-2017.vi"("PWD？"=w15, "数据段"=w38) -> ("通讯包字符串"=w45:string, "通讯包"=→"通讯包":T2)  [unwired: 7 in, 1 out]
  "通讯包字符串" <- w45
  n1601 = String Length(string=w45) -> (length=→"长度":i32)
  "错误常量" <- "错误常量 2"
  "小时数据发送次数" <- 0 ("小时数据发送次数")
  "核查数据发送次数" <- 0 ("核查数据发送次数")
